vi "MC_7_26_12b_JW.vi"() -> ()   [LabVIEW 2011]
uses:
  <vilib>/Utility/file.llb/Read From Spreadsheet File (string).vi
  <vilib>/Utility/inputDevices.llb/keyboardAcquire.vi
  <vilib>/Utility/file.llb/Write To Spreadsheet File (DBL).vi
  <vilib>/Utility/file.llb/Write To Spreadsheet File (string).vi
  <vilib>/regexp/Match Regular Expression.xnode
panel:
  in  "Room Temp":dbl=294.0
  out "No Image 2":path=path "\\\\acad1\\physics/Jurchescu-group/JW-PD/Image Not Found.png"
  out "Save1 Array":string[][](array[string])
  out "XY Graph-Lin":cluster{dbl[], dbl[]}[](graph)
  out "Lin Vd":dbl
  out "Lin-Vg Array-Used":dbl[](array[numeric])
  out "Lin Id-Used":dbl[](array[numeric])
  out "Comments":string
  out "Folder Index":dbl caption="Length"
  out "Current \nRecord":string[](array[string])
  out "Transformer \nHeaders":string[](array[string])
  out "Current Device ID":string
  out "Column":string
  out "Row":string
  out "Rec: Concentration":dbl
  out "Rec: Solvent":string
  out "Rec: Method":string
  in  "?":T1(tab)
  out "Rec: Material":string
  in  "Treatment Concentration (mM):":dbl=30.0
  in  "Surface Treatment:":string
  in  "# Drops*:":dbl=inf
  in  "Solution Temp (C):":dbl=55.0
  in  "Relative Humidity (%):":dbl=nan
  in  "Room Temp (F):":dbl=nan
  in  "Time (s):":dbl=80.0
  out "Accel (RPM/s):":dbl
  in  "RPM:":dbl=1000.0
  in  "Wait Time (s):":dbl=10.0
  in  "Sample #:":dbl=1.0
  in  "Fabricator:":string="Jeremy"
  in  "Data File":path
  out "Data Folder":path
  in  "Image Folder":path
  out "Image File":path=path "D:/UserData/Desktop/Jeremy/WFU/Research/Programs/VI mods/Image Not Found.png"
  in  "Ramp (s):":dbl=3.0
  out "Calc: On/Off":dbl caption="On/Off-Sat" format="%#_4e"
  out "Calc: Off I-Sat":dbl caption="Off I-Sat" format="%#_4e"
  in  "Manuel-Dielectric":bool
  in  "Manuel-Length":bool
  out "Calc: VT-Lin":dbl
  out "New: VT-Lin":dbl
  out "Rec: VT-Lin":dbl caption="VT-Lin" format="%#_3g"
  out "Calc: Trap Density-STS":dbl format="%#_3e"
  out "New: Trap Density-STS":dbl format="%#_3e"
  out "Rec: Trap Density-STS":dbl caption="N-Sat (STS)" format="%#_3e"
  out "Calc: Trap Density-VT":dbl format="%#_3e"
  out "New: Trap Density-VT":dbl format="%#_3e"
  out "Rec: Trap Density-VT":dbl caption="N-Sat (VT)" format="%#_3e"
  out "Calc: Mobility-Lin":dbl format="%#_4e"
  out "New: Mobility-Lin":dbl format="%#_4e"
  out "Rec: Mobility-Lin":dbl caption="Mobility-Lin" format="%#_4e"
  out "Calc: Mobility-Sat":dbl format="%#_4e"
  out "Rec: Length":dbl caption="Length" format="%#_3g"
  out "Rec: Width":dbl caption="Width" format="%#_4g"
  out "Rec: Dielectric (d)":dbl caption="Dielectric (d)" format="%#_3g"
  out "XY Graph":cluster{dbl[], dbl[]}[](graph)
  in  "NumPts":dbl=5.0
  in  "Cancel Button":bool
  in  "Next Button":bool
  in  "Previous Button":bool
  in  "Up Button":bool
  in  "Down Button":bool
  out "Data Name:":string
  in  "Save Changes?":bool
  in  "New: Dielectric":dbl
  in  "New: Length":dbl
  in  "New: Width":dbl
  out "New: Mobility-Sat":dbl format="%#_4e"
  in  "Slide":dbl(slide) step=1.0 scale=-14.3..89.0 scale format="%#_1p"
  in  "Blank Button":bool
  in  "Zoom":i16(slide)=-3 scale=-5.0..5.0
  out "Image Out 2":T2(plugin-control)
  out "Image Out":T2(plugin-control)
  in  "Magnification":u16(ring) items=["5x", "10x", "20x", "50x", "80x"]
  out "Total Width":dbl
  out "Distances":dbl[](array[numeric])
  in  "Undo Button":bool
  in  "Remove Button":bool
  out "Rec: Mobility-Sat":dbl caption="Mobility-Sat" format="%#_4e"
  out "Index":string
  out "Image Name":string
  in  "Export":bool
  out "Calc: VT-Sat":dbl format="%#_3g"
  out "New: VT-Sat":dbl format="%#_3g"
  in  "Manual-Width":bool caption="Manual"
  out "XY Graph 2":cluster{dbl[], dbl[]}[](graph)
  in  "Next Button 2":bool
  in  "Previous Button 2":bool
  in  "Slide 2":dbl(slide) step=1.0 scale=-1.0..82.0 scale format="%#_1p"
  out "Calc: STS":dbl format="%#_3g"
  out "New: STS":dbl format="%#_3g"
  in  "NumPts 2":dbl=5.0 caption="NumPts"
  out "Rec: VT-Sat":dbl caption="VT-Sat" format="%#_3g"
  out "Rec: STS":dbl caption="STS-Sat" format="%#_3g"
  out "Rec: On/Off":dbl caption="On/Off-Sat" format="%#_4e"
  in  "Save Changes? 2":bool
  in  "Save Changes? 3":bool
  out "Date Recorded":string="Date Recorded" caption="Measured"
  out "Date Created":string caption="Fabricated"
  out "Rec: Temp":dbl caption="Sample Temp"
  out "New: Temp":dbl
  out "Rec: Off I-Sat":dbl caption="Off I-Sat" format="%#_4e"
  out "String":string
  in  "No Image":path=path "\\\\acad1\\physics/Jurchescu-group/JW-PD/Image Not Found.png"
  in  "Project":path=path "\\\\acad1\\physics/Jurchescu-group/JW-PD/Group Library/Origin Project Files/DeviceData_7_25a_JWW.opj"
  out "Index 2":dbl
  out "Sat Id-Log-Used":dbl[](array[numeric])
  out "Vg Array-Log-Used":dbl[](array[numeric])
  out "ROI Descriptor out":T3 {"Contours"."Type" items=["No Selection", "Point", "Line", "Rectangle", "Oval", "Polygon", "Freehand Region", "Annulus", "Unused2", "Unused3", "Broken Line", "Freehand Line", "Rotated Rectangle"]}
  out "ROI Descriptor":T3 {"Contours"."Type" items=["No Selection", "Point", "Line", "Rectangle", "Oval", "Polygon", "Freehand Region", "Annulus", "Unused2", "Unused3", "Broken Line", "Freehand Line", "Rotated Rectangle"]}
  out "Numeric 3":dbl
  out "Array 6":dbl[][](array[numeric])
  out "Cluster":T4
  out "Array 5":dbl[](array[numeric])
  out "Array 4":dbl[](array[numeric])
  out "Array 3":dbl[](array[numeric])
  out "Numeric 2":dbl
  out "Numeric":dbl
  out "Sat Id-Used":dbl[](array[numeric])
  out "Sat Vg Array-Used":dbl[](array[numeric])
  out "MobVi Index":dbl
  in  "Row Start":dbl=20.0
  # "Data Locations"
  # "Data Location"
  # "Image Location"
  # "Sample Properties"
  # "*     Inf = Full coverage\n   NaN = Unknown or Not Applicable"
  # "Recorded"
  # "Calculated"
  # "Re-Calculated"
  # "Manual"
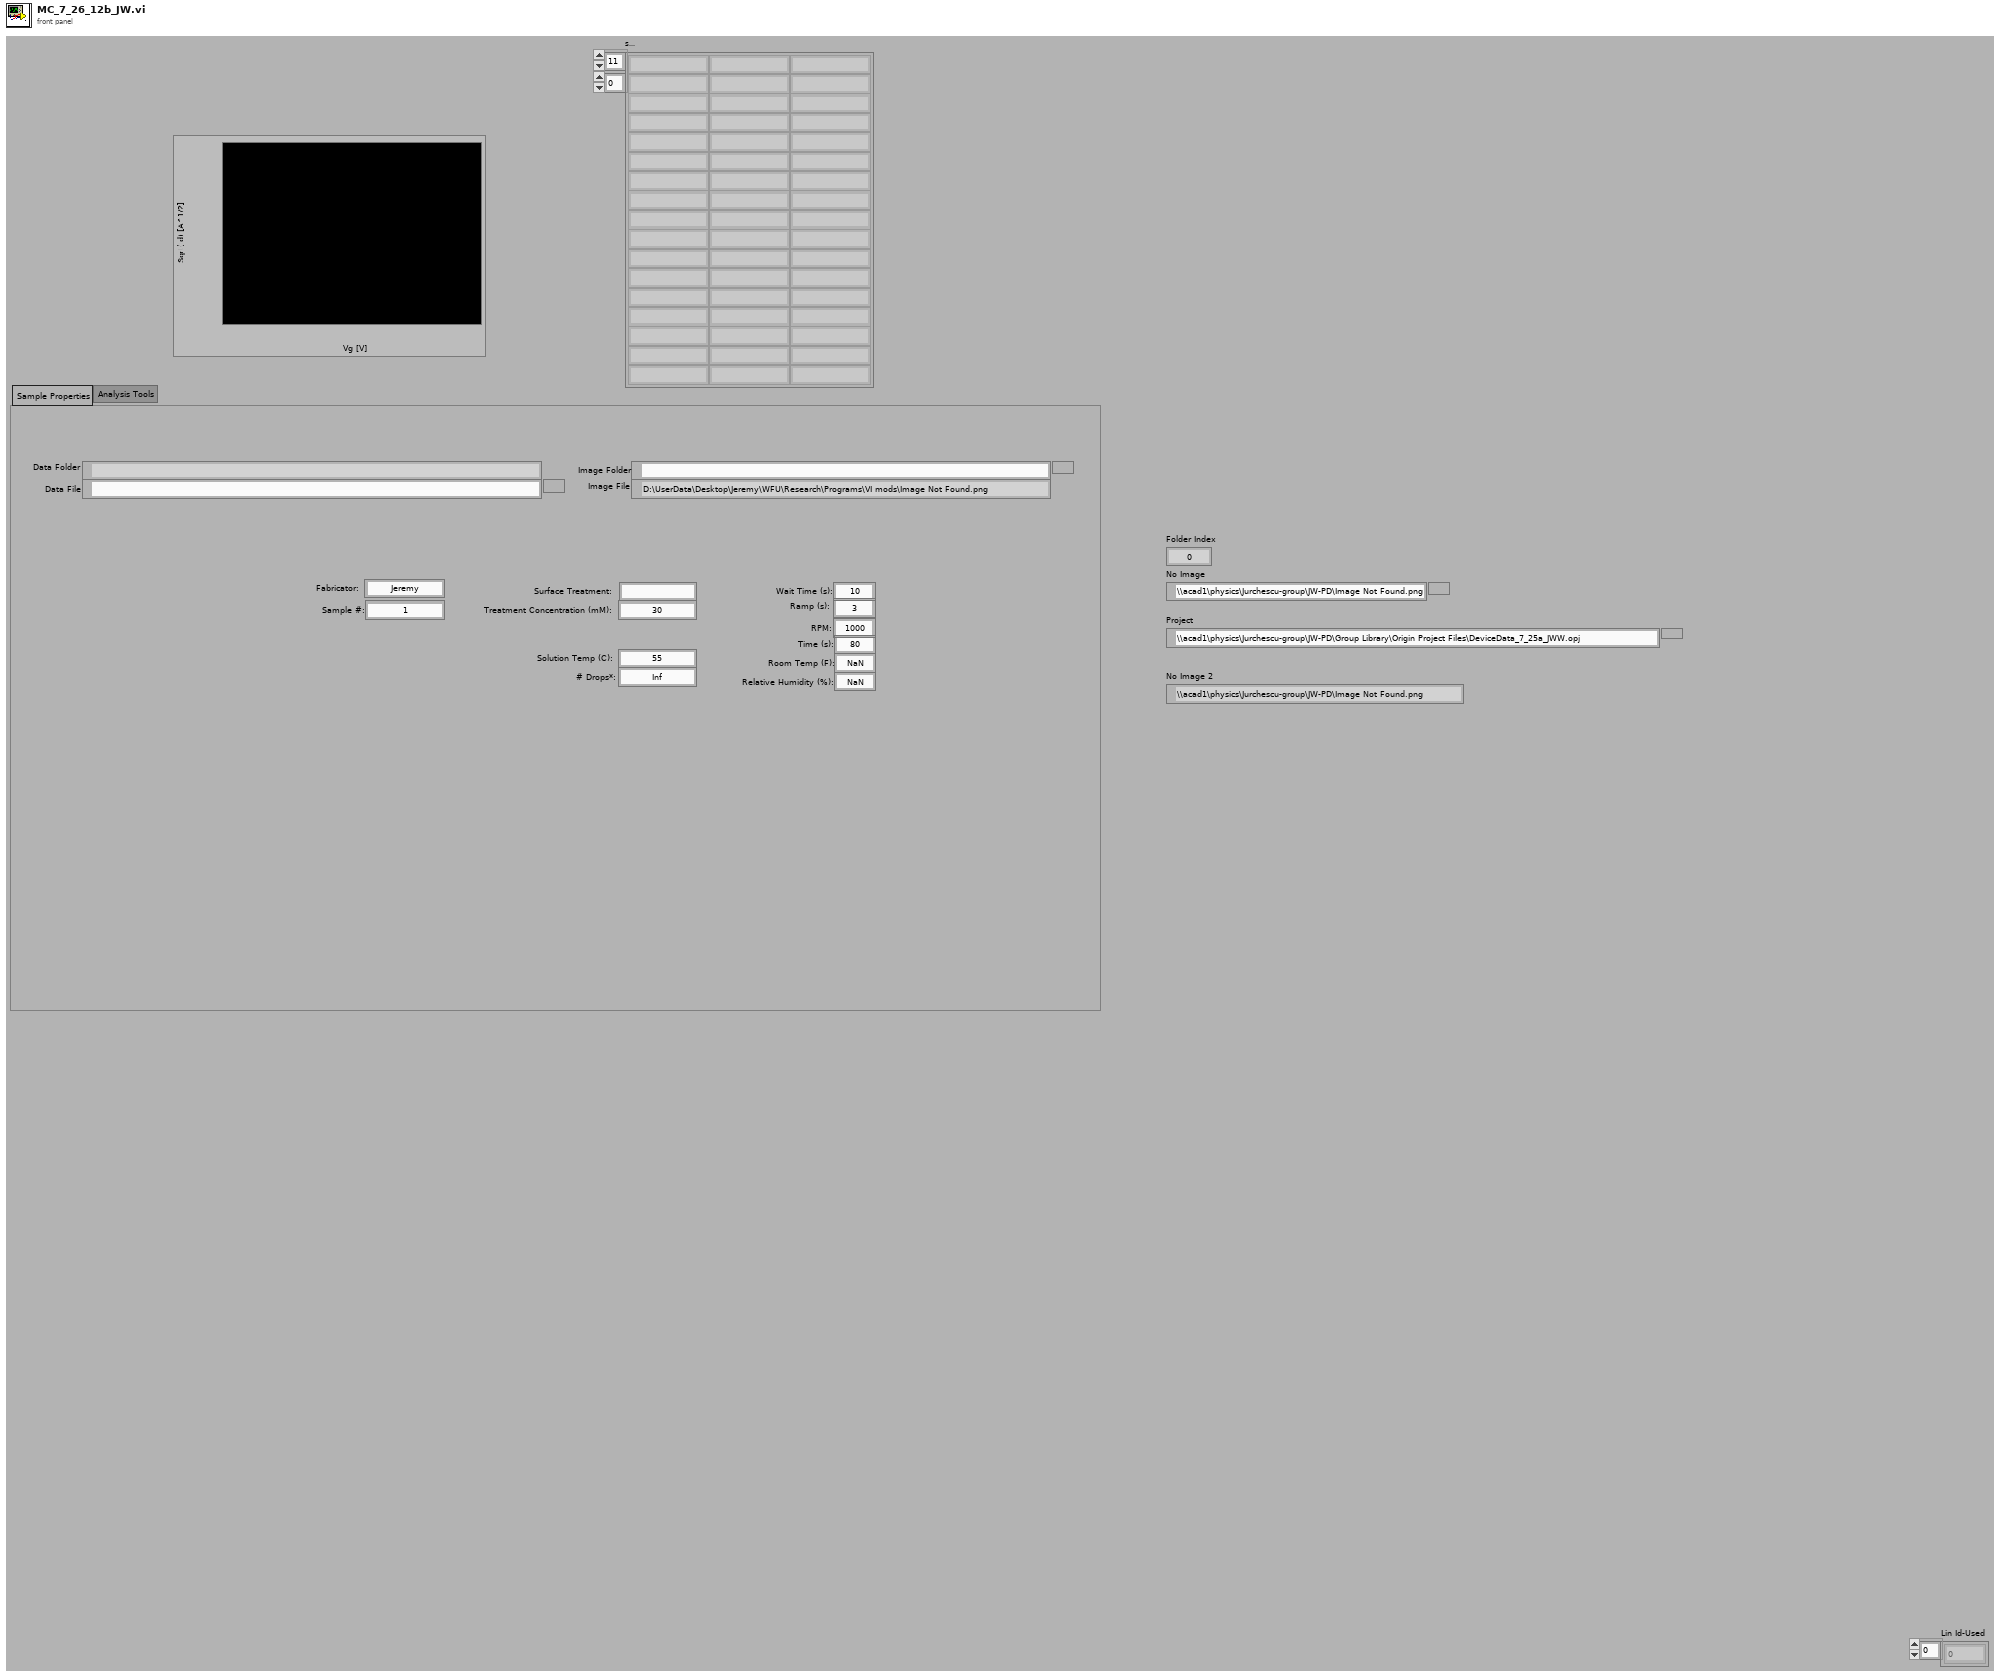
[diagram p1: front panel]
types:
  T1 = enum32{"Sample Properties", "Analysis Tools", "Current Database"}
  T2 = typedef "IMAQ Image.ctl" = refnum<image>
  T3 = typedef "ROI Descriptor" = cluster{"Global Rectangle":i32[], "Contours":cluster{"ID":enum32{"External", "Internal"}, "Type":u32, "Coordinates":i32[]}[]}
  T4 = cluster{"Numeric":dbl, "Numeric 2":dbl, "Numeric 3":dbl, "Numeric 4":dbl}
  T5 = cluster{"Mobility-Sat":dbl, "Moblitity-Lin":dbl, "On/Off":dbl, "Off Current":dbl, "Vt-Sat":dbl, "STS":dbl, "Trap Density-VT":dbl, "Trap Density-STS":dbl}
  T6 = cluster{"Date Recorded":string, "Index":string, "Length":dbl, "Width":dbl, "Sample Temp":dbl}
  T7 = cluster{"Date Created":string, "Material":string, "Solvent":string, "Concentration":dbl, "Method":string, "Dielectric (nm)":dbl, "Treatment":string, "Comments":string}
  T8 = cluster{"Mobility-Sat":dbl, "Vt-Sat":dbl, "Mobility-Lin":dbl, "Vt-Lin":dbl, "Off I-Sat":dbl, "On/Off I-Sat":dbl}
  T9 = cluster{"[0]":cluster{dbl[], dbl[]}, "[1]":cluster{dbl[], dbl[]}, "[2]":cluster{dbl[], dbl[]}, "[3]":cluster{dbl[], dbl[]}, "[4]":cluster{dbl[], dbl[]}, "[5]":cluster{dbl[], dbl[]}, "[6]":cluster{dbl[], dbl[]}, "[7]":cluster{dbl[], dbl[]}, "[8]":cluster{dbl[], dbl[]}}
  T10 = cluster{"Global Rectangle":i32[], "Contours":cluster{"Contour Type":u32, "ROI Type":u32, "Points":i32[]}[]}
  T11 = typedef "LVBoundsTypeDef.ctl" = cluster{"Width":u32, "Height":u32}
  T12 = enum16{"0", "1", "2", "3", "4", "5", "6", "7", "8", "9", "A", "B", "C", "D", "E", "F", "G", "H", "I", "J", "K", "L", "M", "N", "O", "P", "Q", "R", "S", "T", "U", "V", "W", "X", "Y", "Z", "F1", "F2", "F3", "F4", "F5", "F6", "F7", "F8", "F9", "F10", "F11", "F12", "F13", "F14", "F15", "ADD", "BACK", "BACKSLASH", "CAPITAL", "COMMA", "DECIMAL", "DELETE", "DIVIDE", "DOWN", "END", "EQUALS", "ESCAPE", "GRAVE (`)", "HOME", "INSERT", "LBRACKET", "LCONTROL", "LEFT", "L ALT", "LSHIFT", "LWIN", "MINUS", "MULTIPLY", "NEXT", "NUMLOCK", "NUMPAD_0", "NUMPAD_1", "NUMPAD_2", "NUMPAD_3", "NUMPAD_4", "NUMPAD_5", "NUMPAD_6", "NUMPAD_7", "NUMPAD_8", "NUMPAD_9", "PAUSE", "PERIOD", "PRIOR (PG UP)", "RBRACKET", "RCONTROL", "RETURN", "RIGHT", "R ALT", "RSHIFT", "RWIN", "SCROLL", "SEMICOLON", "SLASH", "SPACE", "SUBTRACT", "TAB", "UP", "ENTER (num pad)", "' (quote)"}[]
  T13 = enum16{"0", "1", "2", "3", "4", "5", "6", "7", "8", "9", "A", "B", "C", "D", "E", "F", "G", "H", "I", "J", "K", "L", "M", "N", "O", "P", "Q", "R", "S", "T", "U", "V", "W", "X", "Y", "Z", "F1", "F2", "F3", "F4", "F5", "F6", "F7", "F8", "F9", "F10", "F11", "F12", "F13", "F14", "F15", "ADD", "BACK", "BACKSLASH", "CAPITAL", "COMMA", "DECIMAL", "DELETE", "DIVIDE", "DOWN", "END", "EQUALS", "ESCAPE", "GRAVE (`)", "HOME", "INSERT", "LBRACKET", "LCONTROL", "LEFT", "L ALT", "LSHIFT", "LWIN", "MINUS", "MULTIPLY", "NEXT", "NUMLOCK", "NUMPAD_0", "NUMPAD_1", "NUMPAD_2", "NUMPAD_3", "NUMPAD_4", "NUMPAD_5", "NUMPAD_6", "NUMPAD_7", "NUMPAD_8", "NUMPAD_9", "PAUSE", "PERIOD", "PRIOR (PG UP)", "RBRACKET", "RCONTROL", "RETURN", "RIGHT", "R ALT", "RSHIFT", "RWIN", "SCROLL", "SEMICOLON", "SLASH", "SPACE", "SUBTRACT", "TAB", "UP", "ENTER (num pad)", "' (quote)"}
  T14 = cluster{"Contour Type":u32, "ROI Type":u32, "Points":i32[]}[]
  T15 = cluster{i32[], cluster{"Contour Type":u32, "ROI Type":u32, "Points":i32[]}[]}
  T16 = cluster{string, sgl, bool, bool, bool, bool, bool, bool, i32}
  T17 = cluster{i32, cluster{string, sgl, bool, bool, bool, bool, bool, bool, i32}, i32, i32}
  T18 = cluster{"Contour Type":u32, "ROI Type":u32, "Points":i32[]}
  T19 = cluster{"Points[0]":i32, "Points[1]":i32, "Points[2]":i32, "Points[3]":i32, "Points[4]":i32, "Points[5]":i32, "Points[6]":i32, "Points[7]":i32, "Points[8]":i32}
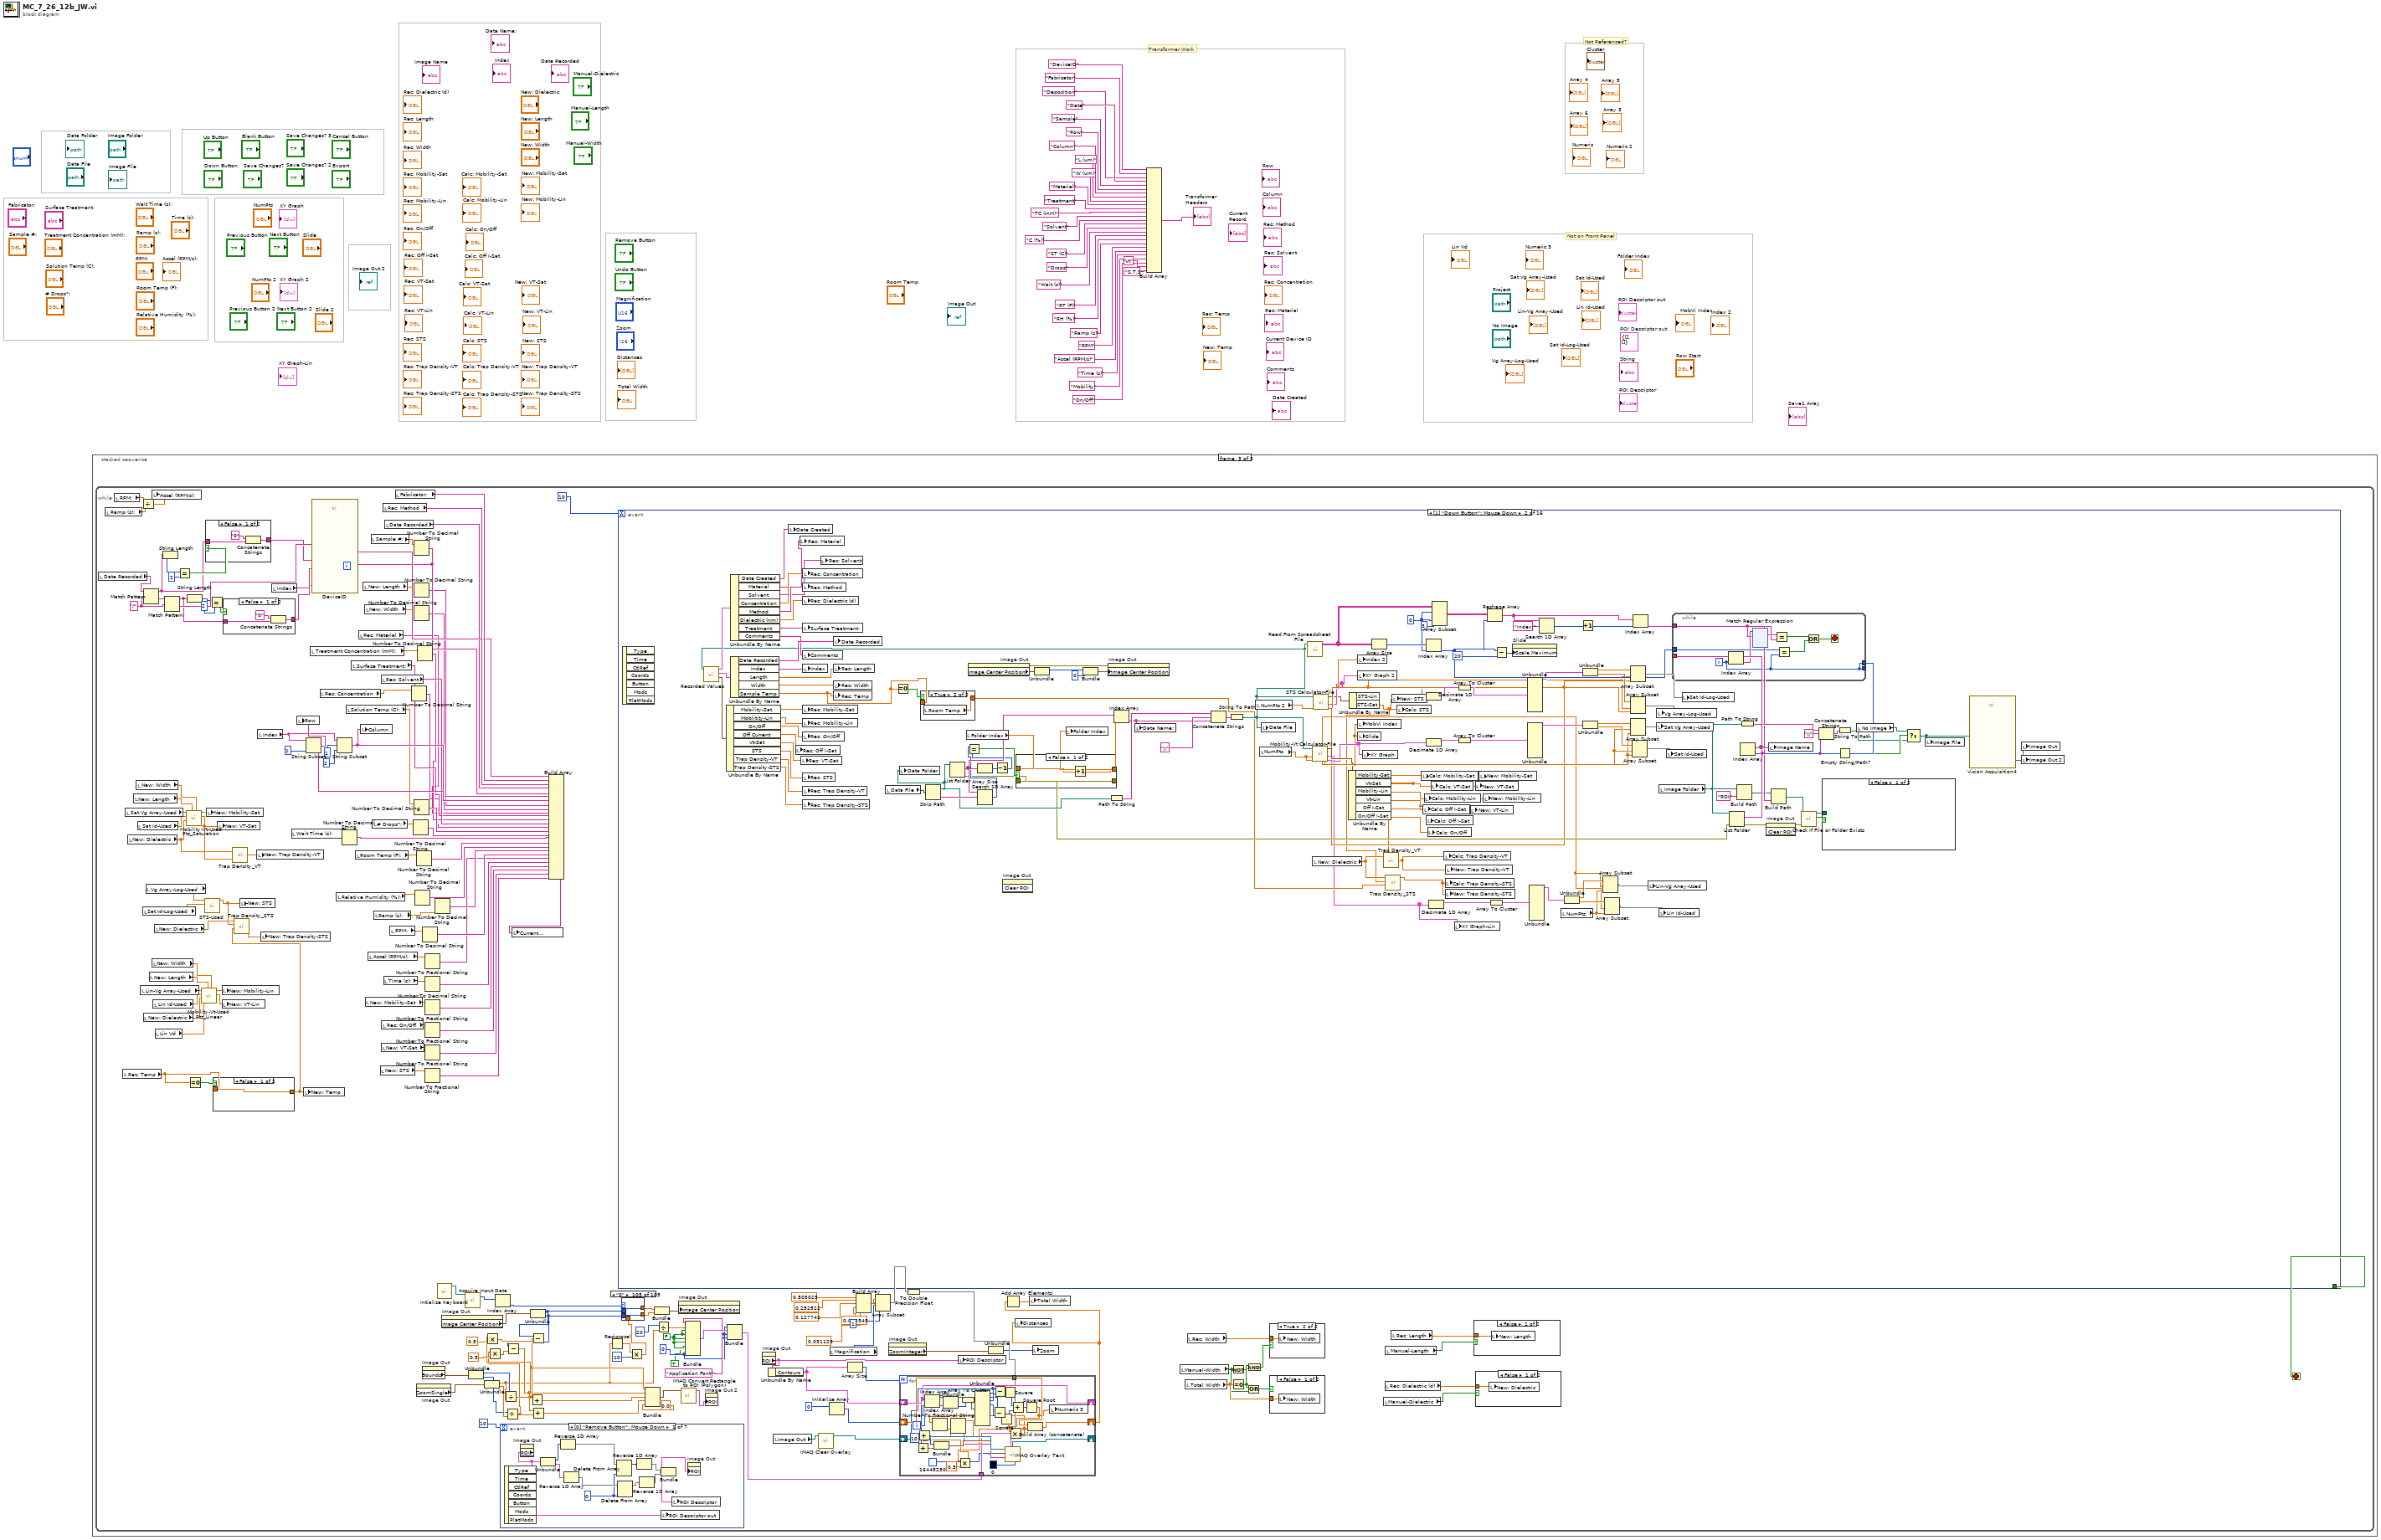
[diagram p0: block diagram]
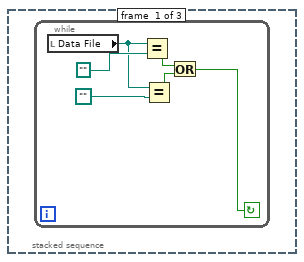
[diagram p2: hidden frame]
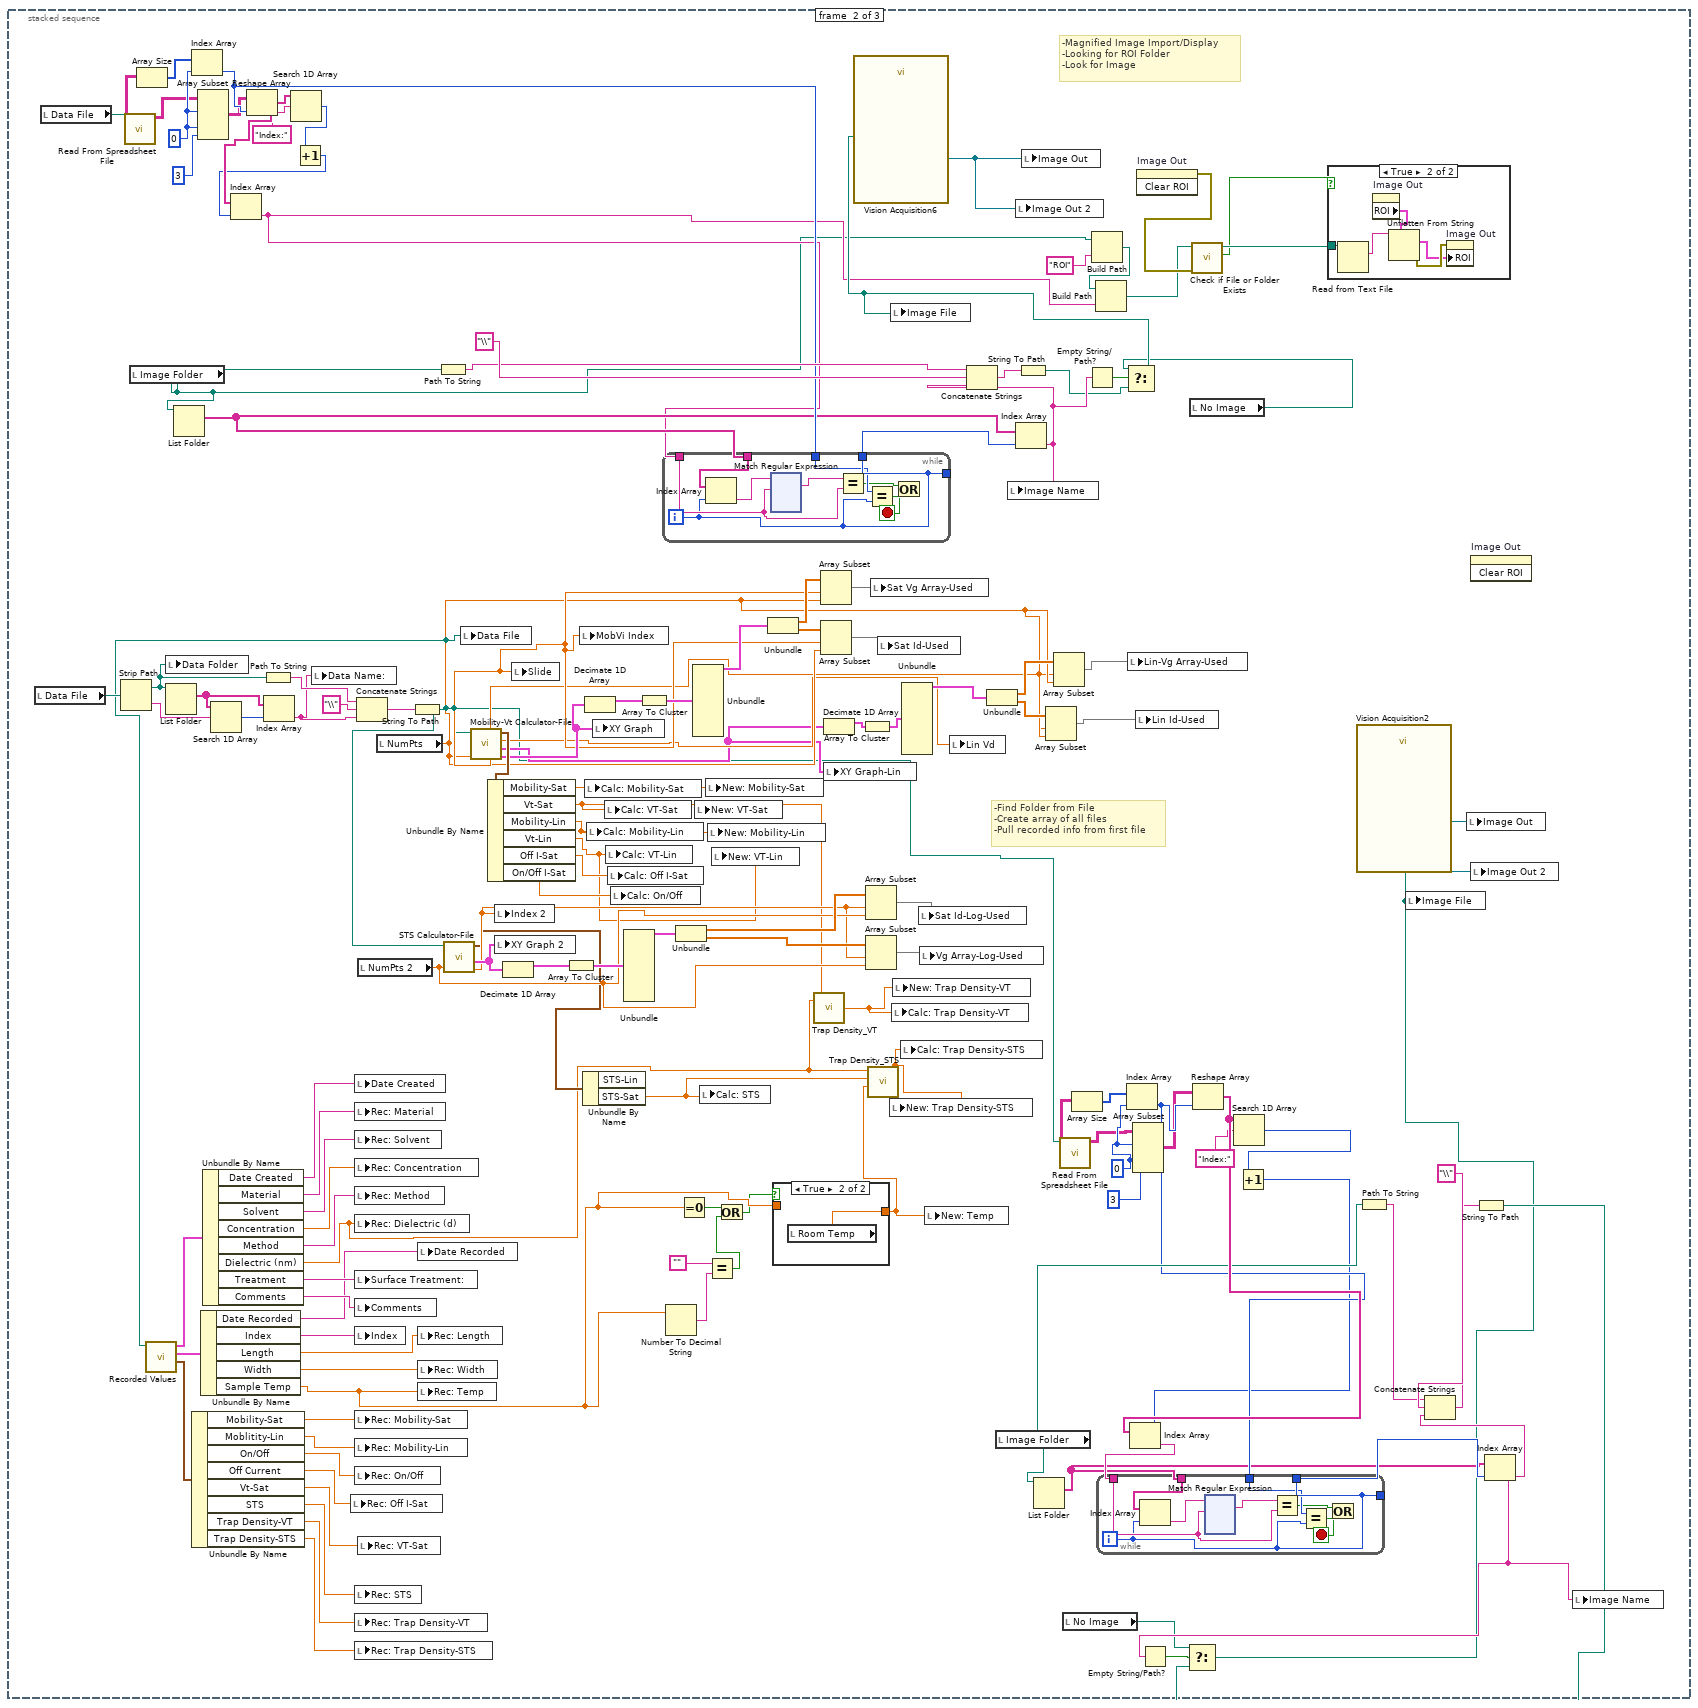
[diagram p3: hidden frame]
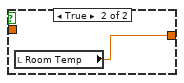
[diagram p6: hidden frame]
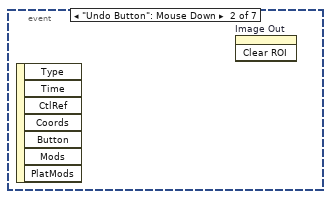
[diagram p13: hidden frame]
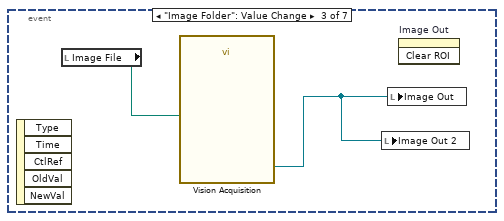
[diagram p14: hidden frame]
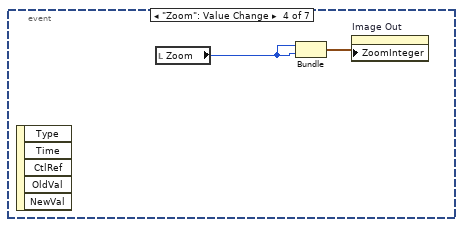
[diagram p15: hidden frame]
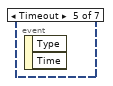
[diagram p16: hidden frame]
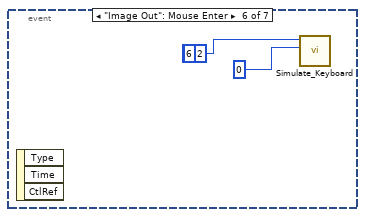
[diagram p17: hidden frame]
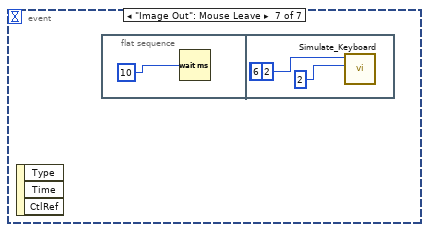
[diagram p18: hidden frame]
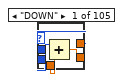
[diagram p19: hidden frame]
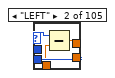
[diagram p20: hidden frame]
diagram:
  (unwired) T3 {"Global Rectangle"=[], "Contours"=[]}  # ROI Descriptor out
  # "Not Referenced?"
  # "Transformer Work"
  # "Not on Front Panel"
  n1 = stacked-sequence {
    frame #0 {
      n2 = while {
        stop <- w29 continue-if-true
        n3 = local read "Data File"() -> (w31:path)
        n4 = Equal?(x=w31, y=path "") -> (x = y?=w33:bool)
        n5 = Equal?(x=w31, y=path "") -> (x = y?=w32:bool)
        n6 = Or(x=w33, y=w32) -> (x .or. y?=w29:bool)
      }
    }
    frame #1 {
      w133 = 0
      w157 = 0
      # "-Find Folder from File\n-Create array of all files\n-Pull recorded info from first file"
      # "-Magnified Image Import/Display\n-Looking for ROI Folder\n-Look for Image"
      n7 = local read "Data File"() -> (w137:path)
      n8 = local read "Data File"() -> (w152:path)
      n9 = Strip Path(path=w137) -> (stripped path=w138:path, name=w124:string)
      n10 = call-poly <vilib>:"Read From Spreadsheet File.vi"("file path (dialog if empty)"=w152) -> ("all rows"=w155:string[][])  [unwired: 6 in, 4 out]
      n11 = local read "Image Folder"() -> (w94:path)
      n12 = Array Size(array=w155) -> (size(s)=w156:i32[])
      n13 = local write "Data Folder"(w138) -> ()
      n14 = List Folder(path=w138) -> (filenames=w128:string[])  [unwired: 3 in, 3 out]
      n15 = List Folder(path=w94) -> (filenames=w161:string[])  [unwired: 3 in, 3 out]
      n16 = Index Array(array=w156, index=w157) -> (element=w163:i32)
      n17 = Array Subset(array=w155, index (row)=w157, index (col)=w157, length (col)=3) -> (w154:string[][])  [unwired: 1 in]
      n18 = Search 1D Array(1D array=w128, element=w124) -> (index of element=w127:i32)  [unwired: 1 in]
      n19 = Reshape Array(w154, w163) -> (w168:string[])
      n20 = Path To String(path=w138) -> (string=w123:string)
      n21 = Index Array(array=w128, index=w127) -> (element=w93:string)
      n22 = Search 1D Array(1D array=w168, element="Index:") -> (index of element=w160:i32)  [unwired: 1 in]
      n23 = Increment(x=w160) -> (x+1=w159:i32)
      n24 = Index Array(array=w168, index=w159) -> (element=w95:string)
      n25 = local write "Data Name:"(w93) -> ()
      n26 = Concatenate Strings(w123, "\\", w93) -> (w125:string)
      n27 = local read "NumPts 2"() -> (w68:dbl)
      n28 = local read "NumPts"() -> (w59:dbl)
      n29 = String To Path(string=w125) -> (path=w52:path)
      n30 = call "Recorded Values.vi"("Path"=w52) -> ("Recorded Char"=w91:T5, "Recorded Prop"=w90:T6, "Fabrication Prop"=w92:T7)  [unwired: 8 in]
      n31 = Unbundle By Name(w91) -> ("Mobility-Sat"=w79:dbl, "Moblitity-Lin"=w78:dbl, "On/Off"=w77:dbl, "Off Current"=w76:dbl, "Vt-Sat"=w38:dbl, "STS"=w75:dbl, "Trap Density-VT"=w74:dbl, "Trap Density-STS"=w73:dbl)
      n32 = Unbundle By Name(w90) -> ("Date Recorded"=w83:string, "Index"=w82:string, "Length"=w81:dbl, "Width"=w80:dbl, "Sample Temp"=w44:dbl)
      n33 = Unbundle By Name(w92) -> ("Date Created"=w72:string, "Material"=w89:string, "Solvent"=w88:string, "Concentration"=w87:dbl, "Method"=w86:string, "Dielectric (nm)"=w48:dbl, "Treatment"=w85:string, "Comments"=w84:string)
      n34 = local write "Rec: Off I-Sat"(w76) -> ()
      n35 = local write "Date Created"(w72) -> ()
      n36 = local write "Rec: Material"(w89) -> ()
      n37 = local write "Rec: Solvent"(w88) -> ()
      n38 = local write "Rec: Concentration"(w87) -> ()
      n39 = local write "Rec: Method"(w86) -> ()
      n40 = local write "Rec: Dielectric (d)"(w48) -> ()
      n41 = local write "Surface Treatment:"(w85) -> ()
      n42 = local write "Comments"(w84) -> ()
      n43 = local write "Index"(w82) -> ()
      n44 = local write "Rec: Mobility-Sat"(w79) -> ()
      n45 = local write "Rec: Mobility-Lin"(w78) -> ()
      n46 = local write "Rec: On/Off"(w77) -> ()
      n47 = local write "Rec: STS"(w75) -> ()
      n48 = local write "Rec: Trap Density-VT"(w74) -> ()
      n49 = local write "Rec: Trap Density-STS"(w73) -> ()
      n50 = local write "Rec: VT-Sat"(w38) -> ()
      n51 = local write "Date Recorded"(w83) -> ()
      n52 = local write "Rec: Length"(w81) -> ()
      n53 = local write "Rec: Width"(w80) -> ()
      n54 = local write "Rec: Temp"(w44) -> ()
      n55 = Path To String(path=w94) -> (string=w165:string)
      n56 = call "STS Calculator-File.vi"("NumPts"=w68, "Path"=w52) -> ("STS Index-Sat"=w66:dbl, "XY Graph-Sat"=w67:cluster{dbl[], dbl[]}[], "Ouput"=w65:cluster{"STS-Sat":dbl, "STS-Lin":dbl})  [unwired: 5 in, 2 out]
      n57 = local write "Data File"(w52) -> ()
      n58 = call "Mobility-Vt Calculator-File.vi"("NumPts"=w59, "Path"=w52) -> ("XY Graph-Sat"=w70:cluster{dbl[], dbl[]}[], "XY Graph-Lin"=w54:cluster{dbl[], dbl[]}[], "Lin Vd"=w55:dbl, "Output"=w71:T8, "Index-Sat"=w69:dbl, "Index-Lin"=w58:dbl)  [unwired: 4 in]
      n59 = Unbundle By Name(w71) -> ("Mobility-Sat"=w47:dbl, "Vt-Sat"=w46:dbl, "Mobility-Lin"=w37:dbl, "Vt-Lin"=w35:dbl, "Off I-Sat"=w53:dbl, "On/Off I-Sat"=w36:dbl)
      n60 = local write "Index 2"(w66) -> ()
      n61 = local write "XY Graph 2"(w67) -> ()
      n62 = Decimate 1D Array(w67) -> (w115:cluster{dbl[], dbl[]}[])  [unwired: 1 out]
      n63 = local write "Slide"(w69) -> ()
      n64 = Array To Cluster(array=w115) -> (cluster=w117:T9)
      n65 = local write "MobVi Index"(w69) -> ()
      n66 = Unbundle By Name(w65) -> ("STS-Sat"=w51:dbl)  [unwired: 1 out]
      n67 = Decimate 1D Array(w70) -> (w151:cluster{dbl[], dbl[]}[])  [unwired: 1 out]
      n68 = local write "Calc: Mobility-Sat"(w47) -> ()
      n69 = local write "Calc: Mobility-Lin"(w37) -> ()
      n70 = local write "XY Graph"(w70) -> ()
      n71 = local write "Calc: VT-Sat"(w46) -> ()
      n72 = local write "Calc: VT-Lin"(w35) -> ()
      n73 = local write "Calc: Off I-Sat"(w53) -> ()
      n74 = local write "Calc: On/Off"(w36) -> ()
      n75 = Unbundle(w117) -> ("[0]"=w116:cluster{dbl[], dbl[]})  [unwired: 8 out]
      n76 = Array To Cluster(array=w151) -> (cluster=w149:T9)
      n77 = while {
        tunnel: w161 -> [w303]
        tunnel: w95 -> [w301]
        tunnel: [w300] -> _
        tunnel: [w300] -> w162
        tunnel: w163 -> [w299]
        i -> [w300]
        stop <- w296 stop-if-true
        n78 = Index Array(array=w303, index=w300) -> (element=w304:string)
        n79 = xnode "Match Regular Expression"("input string"=w304, "regular expression"=w301) -> ("whole match"=w302:string)  [unwired: 4 in, 4 out]
        n80 = Equal?(x=w302, y=w301) -> (x = y?=w298:bool)
        n81 = Equal?(x=w299, y=w300) -> (x = y?=w297:bool)
        n82 = Or(x=w298, y=w297) -> (x .or. y?=w296:bool)
      }
      n83 = Number To Decimal String(number=w44) -> (decimal integer string=w42:string)  [unwired: 1 in]
      n84 = Unbundle(w116) -> (w113:dbl[], w112:dbl[])
      n85 = Equal To 0?(x=w44) -> (x = 0?=w43:bool)
      n86 = Unbundle(w149) -> ("[0]"=w150:cluster{dbl[], dbl[]})  [unwired: 8 out]
      n87 = local write "New: VT-Sat"(w46) -> ()
      n88 = local write "Calc: STS"(w51) -> ()
      n89 = local write "New: Mobility-Sat"(w47) -> ()
      n90 = Equal?(x="", y=w42) -> (x = y?=w40:bool)
      n91 = local write "New: Mobility-Lin"(w37) -> ()
      n92 = local write "New: VT-Lin"(w35) -> ()
      n93 = Or(x=w43, y=w40) -> (x .or. y?=w39:bool)
      n94 = Unbundle(w150) -> (w114:dbl[], w118:dbl[])
      n95 = case shown="True" w39 {
        tunnel: [w169 w170] -> w50
        tunnel: w44 -> [w169 _]
        frame False {
        }
        frame True {
          n96 = local read "Room Temp"() -> (w170:dbl)
        }
      }
      n97 = call "Trap Density_VT.vi"("VT"=w46, "Dielectric"=w48) -> ("Trap Density-VT"=w45:dbl)
      n98 = Array Subset(array=w114, index=w69, length=w59) -> (w121:dbl[])
      n99 = Array Subset(array=w118, index=w69, length=w59) -> (w122:dbl[])
      n100 = Decimate 1D Array(w54) -> (w64:cluster{dbl[], dbl[]}[])  [unwired: 1 out]
      n101 = local write "XY Graph-Lin"(w54) -> ()
      n102 = Array To Cluster(array=w64) -> (cluster=w63:T9)
      n103 = Array Subset(array=w113, index=w66, length=w68) -> (w120:dbl[])
      n104 = Array Subset(array=w112, index=w66, length=w68) -> (w119:dbl[])
      n105 = call "Trap Density_STS.vi"("Temp (T) [K]"=w50, "S.T.S. (S)"=w51, "Dielectric"=w48) -> ("Trap Density (N)"=w49:dbl)  [unwired: 8 in]
      n106 = local write "Sat Vg Array-Used"(w121) -> ()
      n107 = local write "Sat Id-Used"(w122) -> ()
      n108 = local write "New: Trap Density-STS"(w49) -> ()
      n109 = local write "Calc: Trap Density-VT"(w45) -> ()
      n110 = local write "New: Trap Density-VT"(w45) -> ()
      n111 = local write "Calc: Trap Density-STS"(w49) -> ()
      n112 = Unbundle(w63) -> ("[0]"=w62:cluster{dbl[], dbl[]})  [unwired: 8 out]
      n113 = local write "Sat Id-Log-Used"(w120) -> ()
      n114 = local write "Vg Array-Log-Used"(w119) -> ()
      n115 = local write "New: Temp"(w50) -> ()
      n116 = local write "Lin Vd"(w55) -> ()
      n117 = Unbundle(w62) -> (w61:dbl[], w60:dbl[])
      n118 = local read "Image Folder"() -> (w144:path)
      n119 = Index Array(array=w161, index=w162) -> (element=w111:string)
      n120 = Concatenate Strings(w165, "\\", w111) -> (w166:string)
      n121 = local write "Image Name"(w111) -> ()
      n122 = String To Path(string=w166) -> (path=w109:path)
      n123 = List Folder(path=w144) -> (filenames=w140:string[])  [unwired: 3 in, 3 out]
      n124 = Array Subset(array=w60, index=w58, length=w59) -> (w56:dbl[])
      n125 = Array Subset(array=w61, index=w58, length=w59) -> (w57:dbl[])
      n126 = call-poly <vilib>:"Read From Spreadsheet File.vi"("file path (dialog if empty)"=w52) -> ("all rows"=w131:string[][])  [unwired: 6 in, 4 out]
      n127 = local read "No Image"() -> (w103:path)
      n128 = Array Size(array=w131) -> (size(s)=w132:i32[])
      n129 = Empty String/Path?(string/path=w111) -> (empty?=w110:bool)
      n130 = Build Path(base path=w94, name or relative path="ROI") -> (appended path=w97:path)
      n131 = Build Path(base path=w97, name or relative path=w95) -> (appended path=w96:path)
      n132 = Index Array(array=w132, index=w133) -> (element=w143:i32)
      n133 = local write "Lin-Vg Array-Used"(w57) -> ()
      n134 = Array Subset(array=w131, index (row)=w133, index (col)=w133, length (col)=3) -> (w130:string[][])  [unwired: 1 in]
      n135 = local write "Lin Id-Used"(w56) -> ()
      n136 = invoke on="Image Out" class="ImageControl" method="Clear ROI"() -> (error out=w101:errorcluster)  [unwired: 3 in, 2 out]
      n137 = local read "No Image"() -> (w102:path)
      n138 = Select(t=w102, s=w110, f=w109) -> (s? t:f=w108:path)
      n139 = call "Vision Acquisition6"("Image Path"=w108) -> ("Image Out"=w164:T2)  [unwired: 25 in, 1 out]
      n140 = local write "Image File"(w108) -> ()
      n141 = local write "Image Out 2"(w164) -> ()
      n142 = local write "Image Out"(w164) -> ()
      n143 = call <vilib>:"Check if File or Folder Exists.vi"("error in (no error)"=w101, "path"=w96) -> ("file or folder exists?"=w99:bool, "dup path"=w100:path)  [unwired: 7 in, 1 out]
      n144 = Reshape Array(w130, w143) -> (w148:string[])
      n145 = Search 1D Array(1D array=w148, element="Index:") -> (index of element=w136:i32)  [unwired: 1 in]
      n146 = Increment(x=w136) -> (x+1=w135:i32)
      n147 = Index Array(array=w148, index=w135) -> (element=w141:string)
      n148 = while {
        tunnel: w140 -> [w183]
        tunnel: w141 -> [w181]
        tunnel: [w180] -> _
        tunnel: [w180] -> w142
        tunnel: w143 -> [w179]
        i -> [w180]
        stop <- w176 stop-if-true
        n149 = Index Array(array=w183, index=w180) -> (element=w184:string)
        n150 = xnode "Match Regular Expression"("input string"=w184, "regular expression"=w181) -> ("whole match"=w182:string)  [unwired: 4 in, 4 out]
        n151 = Equal?(x=w182, y=w181) -> (x = y?=w178:bool)
        n152 = Equal?(x=w179, y=w180) -> (x = y?=w177:bool)
        n153 = Or(x=w178, y=w177) -> (x .or. y?=w176:bool)
      }
      n154 = case shown="True" w99 {
        tunnel: w100 -> [_ w171]
        frame False {
        }
        frame True {
          n155 = Read from Text File(file (use dialog)=w171) -> (text=w175:string)  [unwired: 3 in, 3 out]
          n156 = property on="Image Out" class="ImageControl"() -> ("ROI"=w172:T10)  [unwired: 2 in, 2 out]
          n157 = Unflatten From String(type=w172, binary string=w175) -> (value=w173:T10, error out=w174:errorcluster)  [unwired: 3 in, 1 out]
          n158 = property on="Image Out" class="ImageControl"(error in=w174, "ROI"=w173) -> ()  [unwired: 1 in, 2 out]
        }
      }
      n159 = Path To String(path=w144) -> (string=w145:string)
      n160 = invoke on="Image Out" class="ImageControl" method="Clear ROI"() -> ()  [unwired: 3 in, 3 out]
      n161 = Index Array(array=w140, index=w142) -> (element=w106:string)
      n162 = Empty String/Path?(string/path=w106) -> (empty?=w107:bool)
      n163 = Concatenate Strings(w145, "\\", w106) -> (w146:string)
      n164 = String To Path(string=w146) -> (path=w105:path)
      n165 = Select(t=w103, s=w107, f=w105) -> (s? t:f=w104:path)
      n166 = call "Vision Acquisition2"("Image Path"=w104) -> ("Image Out"=w139:T2)  [unwired: 25 in, 1 out]
      n167 = local write "Image File"(w104) -> ()
      n168 = local write "Image Out"(w139) -> ()
      n169 = local write "Image Out 2"(w139) -> ()
      n170 = local write "Image Name"(w106) -> ()
    }
    frame #2 {
      n171 = while {
        stop <- w581 stop-if-true
        w477 = "/"
        w531 = FALSE
        w529 = 0
        n172 = local read "Date Recorded"() -> (w480:string)
        n173 = local read "Ramp (s):"() -> (w447:dbl)
        n174 = local read "RPM:"() -> (w448:dbl)
        n175 = local read "Rec: Temp"() -> (w419:dbl)
        n176 = local read "Sat Vg Array-Used"() -> (w436:dbl[])
        n177 = local read "New: Dielectric"() -> (w421:dbl)
        n178 = local read "New: Length"() -> (w437:dbl)
        n179 = local read "New: Width"() -> (w439:dbl)
        n180 = local read "Sat Id-Used"() -> (w435:dbl[])
        n181 = local read "Lin-Vg Array-Used"() -> (w430:dbl[])
        n182 = Divide(x=w448, y=w447) -> (x/y=w446:dbl)
        n183 = local read "Sat Id-Log-Used"() -> (w434:dbl[])
        n184 = local read "New: Dielectric"() -> (w427:dbl)
        n185 = Match Pattern(string=w480, regular expression=w477) -> (before substring=w471:string, after substring=w478:string)  [unwired: 1 in, 2 out]
        n186 = local read "Vg Array-Log-Used"() -> (w433:dbl[])
        n187 = local read "New: Length"() -> (w429:dbl)
        n188 = local write "Accel (RPM/s):"(w446) -> ()
        n189 = local read "New: Width"() -> (w426:dbl)
        n190 = local read "Lin Id-Used"() -> (w431:dbl[])
        n191 = local read "New: Dielectric"() -> (w423:dbl)
        n192 = local read "Lin Vd"() -> (w425:dbl)
        n193 = String Length(string=w471) -> (length=w474:i32)
        n194 = Match Pattern(string=w478, regular expression=w477) -> (before substring=w465:string, after substring=w476:string)  [unwired: 1 in, 2 out]
        n195 = Equal?(x=w474, y=2) -> (x = y?=w472:bool)
        n196 = call "Mobility-Vt-Used Pts_Saturation.vi"("Width"=w439, "Length"=w437, "Dielectric (d)"=w421, "Sat Id Used"=w435, "Vg Used"=w436) -> ("Vt"=w422:dbl, "Mobility"=w438:dbl)  [unwired: 4 in, 1 out]
        n197 = String Length(string=w465) -> (length=w467:i32)
        n198 = Equal To 0?(x=w419) -> (x = 0?=w418:bool)
        n199 = call "Mobility-Vt-Used Pts_Linear.vi"("Width"=w426, "Length"=w429, "Vd"=w425, "Dielectric (d)"=w427, "Sat Id Used"=w431, "Vg Used"=w430) -> ("Vt"=w432:dbl, "Mobility"=w428:dbl)  [unwired: 3 in, 1 out]
        n200 = call "STS-Used.vi"("Id Used"=w434, "Vg-Used"=w433) -> ("STS"=w424:dbl)  [unwired: 9 in]
        n201 = case shown="False" w472 {
          tunnel: w471 -> [w591 w593]
          tunnel: [w590 w593] -> w470
          frame False {
            n202 = Concatenate Strings("0", w591) -> (w590:string)
          }
          frame True {
          }
        }
        n203 = local write "New: Mobility-Sat"(w438) -> ()
        n204 = Equal?(x=w467, y=2) -> (x = y?=w469:bool)
        n205 = case shown="False" w418 {
          tunnel: [w582 w583] -> w416
          tunnel: w419 -> [w582 _]
          frame False {
          }
          frame True {
            n206 = local read "Room Temp"() -> (w583:dbl)
          }
        }
        n207 = local write "New: VT-Sat"(w422) -> ()
        n208 = local write "New: Mobility-Lin"(w428) -> ()
        n209 = local write "New: VT-Lin"(w432) -> ()
        n210 = case shown="False" w469 {
          tunnel: w465 -> [w587 w589]
          tunnel: [w586 w589] -> w466
          frame False {
            n211 = Concatenate Strings("0", w587) -> (w586:string)
          }
          frame True {
          }
        }
        n212 = call "Trap Density_VT.vi"("VT"=w422, "Dielectric"=w421) -> ("Trap Density-VT"=w420:dbl)
        n213 = call "Trap Density_STS.vi"("Temp (T) [K]"=w416, "S.T.S. (S)"=w424, "Dielectric"=w423) -> ("Trap Density (N)"=w417:dbl)  [unwired: 8 in]
        n214 = local write "New: STS"(w424) -> ()
        n215 = local write "New: Trap Density-VT"(w420) -> ()
        n216 = local read "Index"() -> (w450:string)
        n217 = local write "New: Trap Density-STS"(w417) -> ()
        n218 = local read "Index"() -> (w464:string)
        n219 = local read "Wait Time (s):"() -> (w510:dbl)
        n220 = local write "New: Temp"(w416) -> ()
        n221 = String Subset(string=w450, length (rest)=1) -> (substring=w505:string)  [unwired: 1 in]
        n222 = local write "Row"(w505) -> ()
        n223 = local read "Treatment Concentration (mM):"() -> (w458:dbl)
        n224 = local read "Rec: Concentration"() -> (w445:dbl)
        n225 = local read "Relative Humidity (%):"() -> (w455:dbl)
        n226 = String Subset(string=w450, offset (0)=1, length (rest)=2) -> (substring=w506:string)
        n227 = Number To Decimal String(number=w510) -> (decimal integer string=w511:string)  [unwired: 1 in]
        n228 = local read "Solution Temp (C):"() -> (w499:dbl)
        n229 = local read "Surface Treatment:"() -> (w457:string)
        n230 = local read "Room Temp (F):"() -> (w503:dbl)
        n231 = local read "Rec: Material"() -> (w453:string)
        n232 = local write "Column"(w506) -> ()
        n233 = local read "New: Length"() -> (w463:dbl)
        n234 = local read "New: Width"() -> (w462:dbl)
        n235 = local read "New: Mobility-Sat"() -> (w492:dbl)
        n236 = local read "Accel (RPM/s):"() -> (w490:dbl)
        n237 = local read "Sample #:"() -> (w482:dbl)
        n238 = local read "# Drops*:"() -> (w500:dbl)
        n239 = local read "Ramp (s):"() -> (w508:dbl)
        n240 = local read "New: STS"() -> (w484:dbl)
        n241 = local read "Rec: Solvent"() -> (w459:string)
        n242 = local read "New: VT-Sat"() -> (w486:dbl)
        n243 = local read "Rec: On/Off"() -> (w488:dbl)
        n244 = local read "Rec: Method"() -> (w483:string)
        n245 = local read "Time (s):"() -> (w495:dbl)
        n246 = local read "Date Recorded"() -> (w479:string)
        n247 = local read "RPM:"() -> (w496:dbl)
        n248 = local read "Fabricator:"() -> (w504:string)
        n249 = Number To Decimal String(number=w445) -> (decimal integer string=w444:string)  [unwired: 1 in]
        n250 = Number To Decimal String(number=w500) -> (decimal integer string=w501:string)  [unwired: 1 in]
        n251 = Number To Decimal String(number=w482) -> (decimal integer string=w475:string)  [unwired: 1 in]
        n252 = call "DeviceID"("Sample"=w475, "Year"=w476, "Month"=w470, "Day"=w466, "Index"=w464) -> ("Result"=w481:string)  [unwired: 9 in, 1 out]
        n253 = Number To Decimal String(number=w463) -> (decimal integer string=w461:string)  [unwired: 1 in]
        n254 = Number To Decimal String(number=w462) -> (decimal integer string=w460:string)  [unwired: 1 in]
        n255 = Number To Decimal String(number=w499) -> (decimal integer string=w498:string)  [unwired: 1 in]
        n256 = Number To Decimal String(number=w455) -> (decimal integer string=w454:string)  [unwired: 1 in]
        n257 = Number To Decimal String(number=w503) -> (decimal integer string=w502:string)  [unwired: 1 in]
        n258 = property on="Image Out" class="ImageControl"() -> ("ZoomSingle"=w549:cluster{"X":sgl, "Y":sgl})  [unwired: 2 in, 2 out]
        n259 = Number To Decimal String(number=w458) -> (decimal integer string=w456:string)  [unwired: 1 in]
        n260 = property on="Image Out" class="ImageControl"() -> ("Bounds"=w550:T11)  [unwired: 2 in, 2 out]
        n261 = Number To Decimal String(number=w496) -> (decimal integer string=w497:string)  [unwired: 1 in]
        n262 = Number To Fractional String(number=w490) -> (F-format string=w491:string)  [unwired: 3 in]
        n263 = Number To Decimal String(number=w495) -> (decimal integer string=w494:string)  [unwired: 1 in]
        n264 = Number To Fractional String(number=w492) -> (F-format string=w493:string)  [unwired: 3 in]
        n265 = Number To Fractional String(number=w488) -> (F-format string=w489:string)  [unwired: 3 in]
        n266 = Number To Fractional String(number=w486) -> (F-format string=w487:string)  [unwired: 3 in]
        n267 = Number To Fractional String(number=w484) -> (F-format string=w485:string)  [unwired: 3 in]
        n268 = Number To Decimal String(number=w508) -> (decimal integer string=w509:string)  [unwired: 1 in]
        n269 = call <vilib>:"Intialize Keyboard.vi"() -> ("device ID"=w561:refnum<k1>)  [unwired: 10 in, 1 out]
        n270 = property on="Image Out" class="ImageControl"() -> ("Image Center Position"=w556:cluster{"X":u32, "Y":u32})  [unwired: 2 in, 2 out]
        n271 = call-poly <vilib>:"Acquire Input Data.vi"("device ID"=w561) -> ("keys pressed"=w560:T12)  [unwired: 16 in, 2 out]
        n272 = Unbundle(w550) -> ("Width"=w547:u32, "Height"=w546:u32)
        n273 = Unbundle(w549) -> ("X"=w524:sgl, "Y"=w548:sgl)
        n274 = Index Array(array=w560) -> (element=w564:T13)  [unwired: 1 in]
        n275 = event shown="[0] \"Remove Button\": Mouse Down" {
          selector: _ -> [_ _ _ _ _ _ _]
          dyn-events: _ -> [_ _ _ _ _ _ _]
          timeout: 10 -> [_ _ _ _ _ _ _]
          event "Remove Button": Mouse Down {
            w598 = 0
            n276 = event-data() -> ()  [unwired: 1 in, 7 out]
            n277 = property on="Image Out" class="ImageControl"() -> ("ROI"=w596:T10)  [unwired: 2 in, 2 out]
            n278 = Unbundle(w596) -> ("Global Rectangle"=w599:i32[], "Contours"=w601:T14)
            n279 = Reverse 1D Array(array=w599) -> (reversed array=w600:i32[])
            n280 = Reverse 1D Array(array=w601) -> (reversed array=w602:T14)
            n281 = Delete From Array(array=w600, index=w598) -> (array with subset deleted=w603:i32[])  [unwired: 1 in, 1 out]
            n282 = Delete From Array(array=w602, index=w598) -> (array with subset deleted=w604:T14)  [unwired: 1 in, 1 out]
            n283 = Reverse 1D Array(array=w603) -> (reversed array=w605:i32[])
            n284 = Reverse 1D Array(array=w604) -> (reversed array=w606:T14)
            n285 = Bundle(w605, w606) -> (w597:T15)  [unwired: 1 in]
            n286 = local write "ROI Descriptor out"(w596) -> ()
            n287 = local write "ROI Descriptor"(w597) -> ()
            n288 = property on="Image Out" class="ImageControl"("ROI"=w597) -> ()  [unwired: 2 in, 2 out]
          }
          event "Undo Button": Mouse Down {
            n289 = event-data() -> ()  [unwired: 1 in, 7 out]
            n290 = invoke on="Image Out" class="ImageControl" method="Clear ROI"() -> ()  [unwired: 3 in, 3 out]
          }
          event "Image Folder": Value Change {
            n291 = event-data() -> ()  [unwired: 1 in, 5 out]
            n292 = local read "Image File"() -> (w608:path)
            n293 = call "Vision Acquisition"("Image Path"=w608) -> ("Image Out"=w607:T2)  [unwired: 25 in, 1 out]
            n294 = local write "Image Out 2"(w607) -> ()
            n295 = local write "Image Out"(w607) -> ()
            n296 = invoke on="Image Out" class="ImageControl" method="Clear ROI"() -> ()  [unwired: 3 in, 3 out]
          }
          event "Zoom": Value Change {
            n297 = event-data() -> ()  [unwired: 1 in, 5 out]
            n298 = local read "Zoom"() -> (w609:i16)
            n299 = Bundle("Zoom"=w609, "Zoom"=w609) -> (w610:cluster{"Zoom":i16, "Zoom":i16})  [unwired: 1 in]
            n300 = property on="Image Out" class="ImageControl"("ZoomInteger"=w610) -> ()  [unwired: 2 in, 2 out]
          }
          event Timeout {
            n301 = event-data() -> ()  [unwired: 1 in, 2 out]
          }
          event "Image Out": Mouse Enter {
            (unwired) 6
            n302 = event-data() -> ()  [unwired: 1 in, 3 out]
            n303 = call "Simulate_Keyboard.vi"("Action"=0, "Virtual Key"=162) -> ()  [unwired: 7 in, 1 out]
          }
          event "Image Out": Mouse Leave {
            n304 = event-data() -> ()  [unwired: 1 in, 3 out]
            n305 = flat-sequence {
              frame #0 {
                n306 = Wait (ms)(milliseconds to wait=10) -> ()  [unwired: 1 out]
              }
              frame #1 {
                (unwired) 6
                n307 = call "Simulate_Keyboard.vi"("Action"=2, "Virtual Key"=162) -> ()  [unwired: 7 in, 1 out]
              }
            }
          }
        }
        n308 = Divide(x=w547, y=w524) -> (x/y=w537:sgl)
        n309 = Multiply(x=w537, y=0.5) -> (x*y=w543:dbl)
        n310 = Divide(x=w546, y=w548) -> (x/y=w536:sgl)
        n311 = Multiply(x=w536, y=0.5) -> (x*y=w542:dbl)
        n312 = Unbundle(w556) -> ("X"=w538:u32, "Y"=w539:u32)
        n313 = Subtract(x=w539, y=w542) -> (x-y=w540:dbl)
        n314 = Subtract(x=w538, y=w543) -> (x-y=w541:dbl)
        n315 = Add(x=w541, y=w537) -> (x+y=w555:dbl)
        n316 = Add(x=w540, y=w536) -> (x+y=w554:dbl)
        n317 = Build Array(w481, w504, w483, w479, w475, w505, w506, w461, w460, w453, w457, w456, w459, w444, w498, w501, w511, w502, w454, w509, w497, w491, w494, w493, w489, w487, w485) -> (w507:string[])
        n318 = local write "Current \nRecord"(w507) -> ()
        n319 = Reciprocal(x=w524) -> (1/x=w523:sgl)
        n320 = event shown="[1] \"Down Button\": Mouse Down" {
          selector: _ -> [_ _ _ _ _ _ _ _ _ _ _ _ _ _ _ _]
          dyn-events: _ -> [_ _ _ _ _ _ _ _ _ _ _ _ _ _ _ _]
          timeout: 10 -> [_ _ _ _ _ _ _ _ _ _ _ _ _ _ _ _]
          tunnel: [_ _ _ _ _ _ _ _ _ _ _ _ _ TRUE _ TRUE] -> w581
          event Timeout {
            n321 = event-data() -> ()  [unwired: 1 in, 2 out]
          }
          event "Down Button": Mouse Down {
            w950 = 0
            n322 = event-data() -> ()  [unwired: 1 in, 7 out]
            n323 = local read "Data File"() -> (w955:path)
            n324 = Strip Path(path=w955) -> (stripped path=w946:path, name=w964:string)
            n325 = local write "Data Folder"(w946) -> ()
            n326 = List Folder(path=w946) -> (filenames=w960:string[], error out=w900:errorcluster)  [unwired: 3 in, 2 out]
            n327 = local read "Folder Index"() -> (w902:dbl)
            n328 = property on="Image Out" class="ImageControl"() -> (error out=w903:errorcluster, "Image Center Position"=w907:cluster{"X":u32, "Y":u32})  [unwired: 2 in, 1 out]
            n329 = Array Size(array=w960) -> (size(s)=w956:i32)
            n330 = Search 1D Array(1D array=w960, element=w964) -> (index of element=w957:i32)  [unwired: 1 in]
            n331 = Decrement(x=w956) -> (x-1=w958:i32)
            n332 = Equal?(x=w957, y=w958) -> (x = y?=w959:bool)
            n333 = invoke on="Image Out" class="ImageControl" method="Clear ROI"() -> ()  [unwired: 3 in, 3 out]
            n334 = case shown="False" w959 {
              tunnel: w902 -> [w1117 _]
              tunnel: [w1116 0] -> w901
              tunnel: w900 -> [w1115 w1118]
              tunnel: [w1115 w1118] -> w899
              frame False {
                n335 = Increment(x=w1117) -> (x+1=w1116:dbl)
              }
              frame True {
              }
            }
            n336 = Unbundle(w907) -> ("X"=w905:u32)  [unwired: 1 out]
            n337 = local write "Folder Index"(w901) -> ()
            n338 = Bundle("X"=w905, 0) -> (w906:cluster{"X":u32, i32})  [unwired: 1 in]
            n339 = property on="Image Out" class="ImageControl"(error in=w903, "Image Center Position"=w906) -> ()  [unwired: 1 in, 2 out]
            n340 = Path To String(path=w946) -> (string=w965:string)
            n341 = Index Array(array=w960, index=w901) -> (element=w961:string)
            n342 = local write "Data Name:"(w961) -> ()
            n343 = Concatenate Strings(w965, "\\", w961) -> (w963:string)
            n344 = String To Path(string=w963) -> (path=w873:path)
            n345 = call "Recorded Values.vi"("Path"=w873) -> ("Recorded Char"=w967:T5, "Recorded Prop"=w968:T6, "Fabrication Prop"=w966:T7)  [unwired: 8 in]
            n346 = Unbundle By Name(w967) -> ("Mobility-Sat"=w980:dbl, "Moblitity-Lin"=w981:dbl, "On/Off"=w982:dbl, "Off Current"=w983:dbl, "Vt-Sat"=w868:dbl, "STS"=w984:dbl, "Trap Density-VT"=w985:dbl, "Trap Density-STS"=w986:dbl)
            n347 = Unbundle By Name(w966) -> ("Date Created"=w987:string, "Material"=w969:string, "Solvent"=w970:string, "Concentration"=w971:dbl, "Method"=w972:string, "Dielectric (nm)"=w973:dbl, "Treatment"=w974:string, "Comments"=w975:string)
            n348 = Unbundle By Name(w968) -> ("Date Recorded"=w976:string, "Index"=w977:string, "Length"=w978:dbl, "Width"=w979:dbl, "Sample Temp"=w870:dbl)
            n349 = local write "Date Created"(w987) -> ()
            n350 = local write "Rec: Off I-Sat"(w983) -> ()
            n351 = local write "Rec: Material"(w969) -> ()
            n352 = local write "Rec: VT-Sat"(w868) -> ()
            n353 = local write "Rec: Concentration"(w971) -> ()
            n354 = local write "Rec: Method"(w972) -> ()
            n355 = local write "Rec: Dielectric (d)"(w973) -> ()
            n356 = local write "Surface Treatment:"(w974) -> ()
            n357 = local write "Comments"(w975) -> ()
            n358 = local write "Index"(w977) -> ()
            n359 = local write "Rec: Mobility-Sat"(w980) -> ()
            n360 = local write "Rec: Mobility-Lin"(w981) -> ()
            n361 = local write "Rec: On/Off"(w982) -> ()
            n362 = local write "Rec: STS"(w984) -> ()
            n363 = local write "Rec: Trap Density-VT"(w985) -> ()
            n364 = local write "Rec: Trap Density-STS"(w986) -> ()
            n365 = local write "Rec: Solvent"(w970) -> ()
            n366 = local write "Date Recorded"(w976) -> ()
            n367 = local write "Rec: Length"(w978) -> ()
            n368 = local write "Rec: Width"(w979) -> ()
            n369 = local write "Rec: Temp"(w870) -> ()
            n370 = Equal To 0?(x=w870) -> (x = 0?=w871:bool)
            n371 = case shown="True" w871 {
              tunnel: [w988 w989] -> w869
              tunnel: w870 -> [w988 _]
              frame False {
              }
              frame True {
                n372 = local read "Room Temp"() -> (w989:dbl)
              }
            }
            n373 = local read "NumPts 2"() -> (w894:dbl)
            n374 = local read "NumPts"() -> (w898:dbl)
            n375 = local write "Data File"(w873) -> ()
            n376 = call-poly <vilib>:"Read From Spreadsheet File.vi"("file path (dialog if empty)"=w873) -> ("all rows"=w952:string[][])  [unwired: 6 in, 4 out]
            n377 = call "Mobility-Vt Calculator-File.vi"("NumPts"=w898, "Path"=w873) -> ("XY Graph-Sat"=w896:cluster{dbl[], dbl[]}[], "XY Graph-Lin"=w867:cluster{dbl[], dbl[]}[], "Output"=w897:T8, "Index-Sat"=w895:dbl, "Index-Lin"=w881:dbl)  [unwired: 4 in, 1 out]
            n378 = local read "New: Dielectric"() -> (w878:dbl)
            n379 = call "STS Calculator-File.vi"("NumPts"=w894, "Path"=w873) -> ("STS Index-Sat"=w893:dbl, "XY Graph-Sat"=w892:cluster{dbl[], dbl[]}[], "Ouput"=w891:cluster{"STS-Sat":dbl, "STS-Lin":dbl})  [unwired: 5 in, 2 out]
            n380 = Unbundle By Name(w897) -> ("Mobility-Sat"=w890:dbl, "Vt-Sat"=w877:dbl, "Mobility-Lin"=w889:dbl, "Vt-Lin"=w888:dbl, "Off I-Sat"=w874:dbl, "On/Off I-Sat"=w866:dbl)
            n381 = Unbundle By Name(w891) -> ("STS-Sat"=w872:dbl)  [unwired: 1 out]
            n382 = local write "Index 2"(w893) -> ()
            n383 = local write "XY Graph 2"(w892) -> ()
            n384 = local write "MobVi Index"(w895) -> ()
            n385 = local write "Slide"(w895) -> ()
            n386 = local write "XY Graph"(w896) -> ()
            n387 = Array Size(array=w952) -> (size(s)=w951:i32[])
            n388 = call "Trap Density_VT.vi"("VT"=w877, "Dielectric"=w878) -> ("Trap Density-VT"=w876:dbl)
            n389 = call "Trap Density_STS.vi"("Temp (T) [K]"=w869, "S.T.S. (S)"=w872, "Dielectric"=w878) -> ("Trap Density (N)"=w875:dbl)  [unwired: 8 in]
            n390 = local write "New: STS"(w872) -> ()
            n391 = local write "Calc: STS"(w872) -> ()
            n392 = local write "Calc: Mobility-Sat"(w890) -> ()
            n393 = local write "Calc: Off I-Sat"(w888) -> ()
            n394 = local write "Calc: Mobility-Lin"(w889) -> ()
            n395 = Index Array(array=w951, index=w950) -> (element=w932:i32)
            n396 = Decimate 1D Array(w892) -> (w926:cluster{dbl[], dbl[]}[])  [unwired: 1 out]
            n397 = Decimate 1D Array(w896) -> (w936:cluster{dbl[], dbl[]}[])  [unwired: 1 out]
            n398 = local write "Calc: Off I-Sat"(w874) -> ()
            n399 = local write "Calc: On/Off"(w866) -> ()
            n400 = Decimate 1D Array(w867) -> (w887:cluster{dbl[], dbl[]}[])  [unwired: 1 out]
            n401 = local write "Calc: VT-Sat"(w877) -> ()
            n402 = Array Subset(array=w952, index (row)=w950, index (col)=w950, length (col)=3) -> (w953:string[][])  [unwired: 1 in]
            n403 = local write "Calc: Trap Density-VT"(w876) -> ()
            n404 = local write "Calc: Trap Density-STS"(w875) -> ()
            n405 = local write "New: Trap Density-STS"(w875) -> ()
            n406 = local write "New: Trap Density-VT"(w876) -> ()
            n407 = local write "XY Graph-Lin"(w867) -> ()
            n408 = Array To Cluster(array=w926) -> (cluster=w924:T9)
            n409 = Array To Cluster(array=w936) -> (cluster=w938:T9)
            n410 = local write "New: VT-Lin"(w888) -> ()
            n411 = local write "New: VT-Sat"(w877) -> ()
            n412 = local write "New: Mobility-Sat"(w890) -> ()
            n413 = local write "New: Mobility-Lin"(w889) -> ()
            n414 = Reshape Array(w953, w932) -> (w939:string[])
            n415 = Array To Cluster(array=w887) -> (cluster=w886:T9)
            n416 = Subtract(x=w932, y=20) -> (x-y=w931:i32)
            n417 = property on="Slide" class="Slide (strict)"("Scale.Maximum"=w931) -> ()  [unwired: 2 in, 2 out]
            n418 = Unbundle(w924) -> ("[0]"=w925:cluster{dbl[], dbl[]})  [unwired: 8 out]
            n419 = Unbundle(w938) -> ("[0]"=w937:cluster{dbl[], dbl[]})  [unwired: 8 out]
            n420 = Unbundle(w886) -> ("[0]"=w883:cluster{dbl[], dbl[]})  [unwired: 8 out]
            n421 = Search 1D Array(1D array=w939, element="Index:") -> (index of element=w947:i32)  [unwired: 1 in]
            n422 = local read "NumPts"() -> (w882:dbl)
            n423 = Unbundle(w883) -> (w885:dbl[], w884:dbl[])
            n424 = Increment(x=w947) -> (x+1=w948:i32)
            n425 = Unbundle(w925) -> (w923:dbl[], w922:dbl[])
            n426 = Unbundle(w937) -> (w928:dbl[], w927:dbl[])
            n427 = Array Subset(array=w885, index=w881, length=w882) -> (w880:dbl[])
            n428 = Array Subset(array=w884, index=w881, length=w882) -> (w879:dbl[])
            n429 = Array Subset(array=w923, index=w893, length=w894) -> (w930:dbl[])
            n430 = Array Subset(array=w922, index=w893, length=w894) -> (w929:dbl[])
            n431 = Array Subset(array=w928, index=w895, length=w898) -> (w935:dbl[])
            n432 = Array Subset(array=w927, index=w895, length=w898) -> (w934:dbl[])
            n433 = Index Array(array=w939, index=w948) -> (element=w911:string)
            n434 = local write "Lin-Vg Array-Used"(w880) -> ()
            n435 = local write "Sat Vg Array-Used"(w935) -> ()
            n436 = local write "Vg Array-Log-Used"(w929) -> ()
            n437 = local write "Lin Id-Used"(w879) -> ()
            n438 = local read "Image Folder"() -> (w909:path)
            n439 = local write "Sat Id-Used"(w934) -> ()
            n440 = local write "Sat Id-Log-Used"(w930) -> ()
            n441 = List Folder(path=w909, error in=w899) -> (filenames=w945:string[], error out=w912:errorcluster)  [unwired: 2 in, 2 out]
            n442 = while {
              tunnel: w945 -> [w1002]
              tunnel: w911 -> [w1000]
              tunnel: [w999] -> _
              tunnel: [w999] -> w944
              tunnel: w932 -> [w998]
              i -> [w999]
              stop <- w995 stop-if-true
              n443 = Index Array(array=w1002, index=w999) -> (element=w1003:string)
              n444 = xnode "Match Regular Expression"("input string"=w1003, "regular expression"=w1000) -> ("whole match"=w1001:string)  [unwired: 4 in, 4 out]
              n445 = Equal?(x=w1001, y=w1000) -> (x = y?=w997:bool)
              n446 = Equal?(x=w998, y=w999) -> (x = y?=w996:bool)
              n447 = Or(x=w997, y=w996) -> (x .or. y?=w995:bool)
            }
            n448 = Build Path(base path=w909, name or relative path="ROI") -> (appended path=w908:path)
            n449 = Path To String(path=w909) -> (string=w942:string)
            n450 = Index Array(array=w945, index=w944) -> (element=w920:string)
            n451 = invoke on="Image Out" class="ImageControl" method="Clear ROI"(error in=w912) -> (error out=w915:errorcluster)  [unwired: 2 in, 2 out]
            n452 = local write "Image Name"(w920) -> ()
            n453 = Build Path(base path=w908, name or relative path=w911) -> (appended path=w916:path)
            n454 = call <vilib>:"Check if File or Folder Exists.vi"("error in (no error)"=w915, "path"=w916) -> ("file or folder exists?"=w913:bool, "dup path"=w914:path)  [unwired: 7 in, 1 out]
            n455 = Concatenate Strings(w942, "\\", w920) -> (w941:string)
            n456 = case shown="False" w913 {
              tunnel: w914 -> [_ w990]
              frame False {
              }
              frame True {
                n457 = Read from Text File(file (use dialog)=w990) -> (text=w994:string)  [unwired: 3 in, 3 out]
                n458 = property on="Image Out" class="ImageControl"() -> ("ROI"=w991:T10)  [unwired: 2 in, 2 out]
                n459 = Unflatten From String(type=w991, binary string=w994) -> (value=w992:T10, error out=w993:errorcluster)  [unwired: 3 in, 1 out]
                n460 = property on="Image Out" class="ImageControl"(error in=w993, "ROI"=w992) -> ()  [unwired: 1 in, 2 out]
              }
            }
            n461 = String To Path(string=w941) -> (path=w919:path)
            n462 = Empty String/Path?(string/path=w920) -> (empty?=w921:bool)
            n463 = local read "No Image"() -> (w917:path)
            n464 = Select(t=w917, s=w921, f=w919) -> (s? t:f=w918:path)
            n465 = local write "Image File"(w918) -> ()
            n466 = call "Vision Acquisition4"("Image Path"=w918) -> ("Image Out"=w943:T2)  [unwired: 25 in, 1 out]
            n467 = local write "Image Out"(w943) -> ()
            n468 = local write "Image Out 2"(w943) -> ()
          }
          event "Data File": Value Change {
            w1226 = 0
            n469 = event-data() -> ()  [unwired: 1 in, 5 out]
            n470 = local read "Data File"() -> (w1222:path)
            n471 = Strip Path(path=w1222) -> (stripped path=w1221:path, name=w1235:string)
            n472 = local write "Data Folder"(w1221) -> ()
            n473 = property on="Image Out" class="ImageControl"() -> (error out=w1177:errorcluster, "Image Center Position"=w1181:cluster{"X":u32, "Y":u32})  [unwired: 2 in, 1 out]
            n474 = List Folder(path=w1221) -> (filenames=w1231:string[], error out=w1187:errorcluster)  [unwired: 3 in, 2 out]
            n475 = Search 1D Array(1D array=w1231, element=w1235) -> (index of element=w1176:i32)  [unwired: 1 in]
            n476 = local write "Folder Index"(w1176) -> ()
            n477 = Unbundle(w1181) -> ("X"=w1179:u32)  [unwired: 1 out]
            n478 = Path To String(path=w1221) -> (string=w1236:string)
            n479 = Index Array(array=w1231, index=w1176) -> (element=w1232:string)
            n480 = Bundle("X"=w1179, 0) -> (w1180:cluster{"X":u32, i32})  [unwired: 1 in]
            n481 = local write "Data Name:"(w1232) -> ()
            n482 = property on="Image Out" class="ImageControl"(error in=w1177, "Image Center Position"=w1180) -> ()  [unwired: 1 in, 2 out]
            n483 = Concatenate Strings(w1236, "\\", w1232) -> (w1234:string)
            n484 = String To Path(string=w1234) -> (path=w1127:path)
            n485 = call "Recorded Values.vi"("Path"=w1127) -> ("Recorded Char"=w1174:T5, "Recorded Prop"=w1173:T6, "Fabrication Prop"=w1175:T7)  [unwired: 8 in]
            n486 = Unbundle By Name(w1174) -> ("Mobility-Sat"=w1161:dbl, "Moblitity-Lin"=w1160:dbl, "On/Off"=w1159:dbl, "Off Current"=w1158:dbl, "Vt-Sat"=w1123:dbl, "STS"=w1157:dbl, "Trap Density-VT"=w1156:dbl, "Trap Density-STS"=w1155:dbl)
            n487 = Unbundle By Name(w1175) -> ("Date Created"=w1154:string, "Material"=w1172:string, "Solvent"=w1171:string, "Concentration"=w1170:dbl, "Method"=w1169:string, "Dielectric (nm)"=w1168:dbl, "Treatment"=w1167:string, "Comments"=w1166:string)
            n488 = Unbundle By Name(w1173) -> ("Date Recorded"=w1165:string, "Index"=w1164:string, "Length"=w1163:dbl, "Width"=w1162:dbl, "Sample Temp"=w1125:dbl)
            n489 = local write "Date Created"(w1154) -> ()
            n490 = local write "Rec: Material"(w1172) -> ()
            n491 = local write "Rec: Off I-Sat"(w1158) -> ()
            n492 = local write "Rec: VT-Sat"(w1123) -> ()
            n493 = local write "Rec: Concentration"(w1170) -> ()
            n494 = local write "Rec: Method"(w1169) -> ()
            n495 = local write "Rec: Dielectric (d)"(w1168) -> ()
            n496 = local write "Surface Treatment:"(w1167) -> ()
            n497 = local write "Comments"(w1166) -> ()
            n498 = local write "Index"(w1164) -> ()
            n499 = local write "Rec: Mobility-Sat"(w1161) -> ()
            n500 = local write "Rec: Mobility-Lin"(w1160) -> ()
            n501 = local write "Rec: On/Off"(w1159) -> ()
            n502 = local write "Rec: STS"(w1157) -> ()
            n503 = local write "Rec: Trap Density-VT"(w1156) -> ()
            n504 = local write "Rec: Trap Density-STS"(w1155) -> ()
            n505 = local write "Rec: Solvent"(w1171) -> ()
            n506 = local write "Date Recorded"(w1165) -> ()
            n507 = local write "Rec: Length"(w1163) -> ()
            n508 = local write "Rec: Width"(w1162) -> ()
            n509 = local write "Rec: Temp"(w1125) -> ()
            n510 = Equal To 0?(x=w1125) -> (x = 0?=w1126:bool)
            n511 = case shown="False" w1126 {
              tunnel: [w1237 w1238] -> w1124
              tunnel: w1125 -> [w1237 _]
              frame False {
              }
              frame True {
                n512 = local read "Room Temp"() -> (w1238:dbl)
              }
            }
            n513 = local read "NumPts 2"() -> (w1149:dbl)
            n514 = local write "Data File"(w1127) -> ()
            n515 = local read "NumPts"() -> (w1150:dbl)
            n516 = call-poly <vilib>:"Read From Spreadsheet File.vi"("file path (dialog if empty)"=w1127) -> ("all rows"=w1228:string[][])  [unwired: 6 in, 4 out]
            n517 = local read "New: Dielectric"() -> (w1133:dbl)
            n518 = call "STS Calculator-File.vi"("NumPts"=w1149, "Path"=w1127) -> ("STS Index-Sat"=w1147:dbl, "XY Graph-Sat"=w1148:cluster{dbl[], dbl[]}[], "Ouput"=w1146:cluster{"STS-Sat":dbl, "STS-Lin":dbl})  [unwired: 5 in, 2 out]
            n519 = call "Mobility-Vt Calculator-File.vi"("NumPts"=w1150, "Path"=w1127) -> ("XY Graph-Sat"=w1153:cluster{dbl[], dbl[]}[], "XY Graph-Lin"=w1122:cluster{dbl[], dbl[]}[], "Output"=w1151:T8, "Index-Sat"=w1152:dbl, "Index-Lin"=w1139:dbl)  [unwired: 4 in, 1 out]
            n520 = Unbundle By Name(w1151) -> ("Mobility-Sat"=w1135:dbl, "Vt-Sat"=w1129:dbl, "Mobility-Lin"=w1134:dbl, "Vt-Lin"=w1120:dbl, "Off I-Sat"=w1128:dbl, "On/Off I-Sat"=w1121:dbl)
            n521 = local write "Index 2"(w1147) -> ()
            n522 = local write "XY Graph 2"(w1148) -> ()
            n523 = Unbundle By Name(w1146) -> ("STS-Sat"=w1130:dbl)  [unwired: 1 out]
            n524 = local write "MobVi Index"(w1152) -> ()
            n525 = Array Size(array=w1228) -> (size(s)=w1227:i32[])
            n526 = call "Trap Density_VT.vi"("VT"=w1129, "Dielectric"=w1133) -> ("Trap Density-VT"=w1132:dbl)
            n527 = call "Trap Density_STS.vi"("Temp (T) [K]"=w1124, "S.T.S. (S)"=w1130, "Dielectric"=w1133) -> ("Trap Density (N)"=w1131:dbl)  [unwired: 8 in]
            n528 = local write "Slide"(w1152) -> ()
            n529 = local write "Calc: Mobility-Lin"(w1134) -> ()
            n530 = local write "Calc: Mobility-Sat"(w1135) -> ()
            n531 = local write "Calc: VT-Sat"(w1129) -> ()
            n532 = local write "Calc: Off I-Sat"(w1128) -> ()
            n533 = local write "Calc: VT-Lin"(w1120) -> ()
            n534 = local write "Calc: On/Off"(w1121) -> ()
            n535 = local write "Calc: STS"(w1130) -> ()
            n536 = Decimate 1D Array(w1122) -> (w1145:cluster{dbl[], dbl[]}[])  [unwired: 1 out]
            n537 = local write "Calc: Trap Density-VT"(w1132) -> ()
            n538 = local write "Calc: Trap Density-STS"(w1131) -> ()
            n539 = local write "New: Trap Density-STS"(w1131) -> ()
            n540 = local write "New: Trap Density-VT"(w1132) -> ()
            n541 = local write "XY Graph-Lin"(w1122) -> ()
            n542 = local write "New: VT-Sat"(w1129) -> ()
            n543 = Decimate 1D Array(w1148) -> (w1202:cluster{dbl[], dbl[]}[])  [unwired: 1 out]
            n544 = Index Array(array=w1227, index=w1226) -> (element=w1208:i32)
            n545 = Decimate 1D Array(w1153) -> (w1211:cluster{dbl[], dbl[]}[])  [unwired: 1 out]
            n546 = local write "XY Graph"(w1153) -> ()
            n547 = local write "New: Mobility-Lin"(w1134) -> ()
            n548 = Array Subset(array=w1228, index (row)=w1226, index (col)=w1226, length (col)=3) -> (w1229:string[][])  [unwired: 1 in]
            n549 = local write "New: VT-Lin"(w1120) -> ()
            n550 = Array To Cluster(array=w1145) -> (cluster=w1144:T9)
            n551 = local write "New: STS"(w1130) -> ()
            n552 = local write "New: Mobility-Sat"(w1135) -> ()
            n553 = Array To Cluster(array=w1202) -> (cluster=w1200:T9)
            n554 = Array To Cluster(array=w1211) -> (cluster=w1213:T9)
            n555 = Reshape Array(w1229, w1208) -> (w1214:string[])
            n556 = Subtract(x=w1208, y=20) -> (x-y=w1206:i32)
            n557 = Unbundle(w1144) -> ("[0]"=w1143:cluster{dbl[], dbl[]})  [unwired: 8 out]
            n558 = property on="Slide" class="Slide (strict)"("Scale.Maximum"=w1206) -> ()  [unwired: 2 in, 2 out]
            n559 = local read "NumPts"() -> (w1140:dbl)
            n560 = Unbundle(w1143) -> (w1142:dbl[], w1141:dbl[])
            n561 = Unbundle(w1200) -> ("[0]"=w1201:cluster{dbl[], dbl[]})  [unwired: 8 out]
            n562 = Unbundle(w1213) -> ("[0]"=w1212:cluster{dbl[], dbl[]})  [unwired: 8 out]
            n563 = Search 1D Array(1D array=w1214, element="Index:") -> (index of element=w1223:i32)  [unwired: 1 in]
            n564 = local read "NumPts"() -> (w1136:dbl)
            n565 = Array Subset(array=w1142, index=w1139, length=w1140) -> (w1138:dbl[])
            n566 = Array Subset(array=w1141, index=w1139, length=w1140) -> (w1137:dbl[])
            n567 = Increment(x=w1223) -> (x+1=w1224:i32)
            n568 = Unbundle(w1201) -> (w1198:dbl[], w1197:dbl[])
            n569 = Unbundle(w1212) -> (w1199:dbl[], w1203:dbl[])
            n570 = local read "Image Folder"() -> (w1183:path)
            n571 = local write "Lin-Vg Array-Used"(w1138) -> ()
            n572 = Array Subset(array=w1198, index=w1147, length=w1149) -> (w1205:dbl[])
            n573 = Array Subset(array=w1197, index=w1147, length=w1149) -> (w1204:dbl[])
            n574 = Array Subset(array=w1199, index=w1152, length=w1136) -> (w1210:dbl[])
            n575 = Array Subset(array=w1203, index=w1152, length=w1136) -> (w1209:dbl[])
            n576 = Index Array(array=w1214, index=w1224) -> (element=w1185:string)
            n577 = local write "Lin Id-Used"(w1137) -> ()
            n578 = local write "Sat Vg Array-Used"(w1210) -> ()
            n579 = local write "Vg Array-Log-Used"(w1204) -> ()
            n580 = local write "Sat Id-Log-Used"(w1205) -> ()
            n581 = local write "Sat Id-Used"(w1209) -> ()
            n582 = local write "Index"(w1185) -> ()
            n583 = List Folder(path=w1183, error in=w1187) -> (filenames=w1219:string[], error out=w1186:errorcluster)  [unwired: 2 in, 2 out]
            n584 = Build Path(base path=w1183, name or relative path="ROI") -> (appended path=w1182:path)
            n585 = while {
              tunnel: w1219 -> [w1251]
              tunnel: w1185 -> [w1249]
              tunnel: [w1248] -> _
              tunnel: [w1248] -> w1218
              tunnel: w1208 -> [w1247]
              i -> [w1248]
              stop <- w1244 stop-if-true
              n586 = Index Array(array=w1251, index=w1248) -> (element=w1252:string)
              n587 = xnode "Match Regular Expression"("input string"=w1252, "regular expression"=w1249) -> ("whole match"=w1250:string)  [unwired: 4 in, 4 out]
              n588 = Equal?(x=w1250, y=w1249) -> (x = y?=w1246:bool)
              n589 = Equal?(x=w1247, y=w1248) -> (x = y?=w1245:bool)
              n590 = Or(x=w1246, y=w1245) -> (x .or. y?=w1244:bool)
            }
            n591 = invoke on="Image Out" class="ImageControl" method="Clear ROI"(error in=w1186) -> (error out=w1190:errorcluster)  [unwired: 2 in, 2 out]
            n592 = Build Path(base path=w1182, name or relative path=w1185) -> (appended path=w1191:path)
            n593 = call <vilib>:"Check if File or Folder Exists.vi"("error in (no error)"=w1190, "path"=w1191) -> ("file or folder exists?"=w1188:bool, "dup path"=w1189:path)  [unwired: 7 in, 1 out]
            n594 = case shown="True" w1188 {
              tunnel: w1189 -> [_ w1239]
              frame False {
              }
              frame True {
                n595 = Read from Text File(file (use dialog)=w1239) -> (text=w1243:string)  [unwired: 3 in, 3 out]
                n596 = property on="Image Out" class="ImageControl"() -> ("ROI"=w1240:T10)  [unwired: 2 in, 2 out]
                n597 = Unflatten From String(type=w1240, binary string=w1243) -> (value=w1241:T10, error out=w1242:errorcluster)  [unwired: 3 in, 1 out]
                n598 = property on="Image Out" class="ImageControl"(error in=w1242, "ROI"=w1241) -> ()  [unwired: 1 in, 2 out]
              }
            }
            n599 = invoke on="Image Out" class="ImageControl" method="Clear ROI"() -> ()  [unwired: 3 in, 3 out]
            n600 = Path To String(path=w1183) -> (string=w1217:string)
            n601 = Index Array(array=w1219, index=w1218) -> (element=w1195:string)
            n602 = Concatenate Strings(w1217, "\\", w1195) -> (w1216:string)
            n603 = local write "Image Name"(w1195) -> ()
            n604 = String To Path(string=w1216) -> (path=w1194:path)
            n605 = Empty String/Path?(string/path=w1195) -> (empty?=w1196:bool)
            n606 = local read "No Image"() -> (w1192:path)
            n607 = Select(t=w1192, s=w1196, f=w1194) -> (s? t:f=w1193:path)
            n608 = local write "Image File"(w1193) -> ()
            n609 = call "Vision Acquisition3"("Image Path"=w1193) -> ("Image Out"=w1220:T2)  [unwired: 25 in, 1 out]
            n610 = local write "Image Out"(w1220) -> ()
            n611 = local write "Image Out 2"(w1220) -> ()
          }
          event "Up Button": Mouse Down {
            w1471 = 0
            n612 = event-data() -> ()  [unwired: 1 in, 5 out]
            n613 = local read "Data File"() -> (w1467:path)
            n614 = Strip Path(path=w1467) -> (stripped path=w1466:path, name=w1482:string)
            n615 = local write "Data Folder"(w1466) -> ()
            n616 = List Folder(path=w1466) -> (filenames=w1476:string[], error out=w1433:errorcluster)  [unwired: 3 in, 2 out]
            n617 = Array Size(array=w1476) -> (size(s)=w1421:i32)
            n618 = Search 1D Array(1D array=w1476, element=w1482) -> (index of element=w1477:i32)  [unwired: 1 in]
            n619 = Equal To 0?(x=w1477) -> (x = 0?=w1478:bool)
            n620 = local read "Folder Index"() -> (w1420:dbl)
            n621 = property on="Image Out" class="ImageControl"() -> (error out=w1423:errorcluster, "Image Center Position"=w1427:cluster{"X":u32, "Y":u32})  [unwired: 2 in, 1 out]
            n622 = case shown="True" w1478 {
              tunnel: w1420 -> [w1612 _]
              tunnel: [w1611 w1613] -> w1419
              tunnel: w1421 -> [_ w1614]
              frame False {
                n623 = Decrement(x=w1612) -> (x-1=w1611:dbl)
              }
              frame True {
                n624 = Decrement(x=w1614) -> (x-1=w1613:i32)
              }
            }
            n625 = Unbundle(w1427) -> ("X"=w1425:u32)  [unwired: 1 out]
            n626 = local write "Folder Index"(w1419) -> ()
            n627 = Bundle("X"=w1425, 0) -> (w1426:cluster{"X":u32, i32})  [unwired: 1 in]
            n628 = Path To String(path=w1466) -> (string=w1483:string)
            n629 = Index Array(array=w1476, index=w1419) -> (element=w1479:string)
            n630 = local write "Data Name:"(w1479) -> ()
            n631 = property on="Image Out" class="ImageControl"(error in=w1423, "Image Center Position"=w1426) -> ()  [unwired: 1 in, 2 out]
            n632 = Concatenate Strings(w1483, "\\", w1479) -> (w1481:string)
            n633 = String To Path(string=w1481) -> (path=w1370:path)
            n634 = call "Recorded Values.vi"("Path"=w1370) -> ("Recorded Char"=w1417:T5, "Recorded Prop"=w1416:T6, "Fabrication Prop"=w1418:T7)  [unwired: 8 in]
            n635 = Unbundle By Name(w1417) -> ("Mobility-Sat"=w1404:dbl, "Moblitity-Lin"=w1403:dbl, "On/Off"=w1402:dbl, "Off Current"=w1401:dbl, "Vt-Sat"=w1366:dbl, "STS"=w1400:dbl, "Trap Density-VT"=w1399:dbl, "Trap Density-STS"=w1398:dbl)
            n636 = Unbundle By Name(w1418) -> ("Date Created"=w1397:string, "Material"=w1415:string, "Solvent"=w1414:string, "Concentration"=w1413:dbl, "Method"=w1412:string, "Dielectric (nm)"=w1411:dbl, "Treatment"=w1410:string, "Comments"=w1409:string)
            n637 = Unbundle By Name(w1416) -> ("Date Recorded"=w1408:string, "Index"=w1407:string, "Length"=w1406:dbl, "Width"=w1405:dbl, "Sample Temp"=w1367:dbl)
            n638 = local write "Date Created"(w1397) -> ()
            n639 = local write "Rec: Material"(w1415) -> ()
            n640 = local write "Rec: Off I-Sat"(w1401) -> ()
            n641 = local write "Rec: VT-Sat"(w1366) -> ()
            n642 = local write "Rec: Solvent"(w1414) -> ()
            n643 = local write "Rec: Concentration"(w1413) -> ()
            n644 = local write "Rec: Method"(w1412) -> ()
            n645 = local write "Rec: Dielectric (d)"(w1411) -> ()
            n646 = local write "Surface Treatment:"(w1410) -> ()
            n647 = local write "Comments"(w1409) -> ()
            n648 = local write "Index"(w1407) -> ()
            n649 = local write "Rec: Mobility-Sat"(w1404) -> ()
            n650 = local write "Rec: Mobility-Lin"(w1403) -> ()
            n651 = local write "Rec: On/Off"(w1402) -> ()
            n652 = local write "Rec: STS"(w1400) -> ()
            n653 = local write "Rec: Trap Density-VT"(w1399) -> ()
            n654 = local write "Rec: Trap Density-STS"(w1398) -> ()
            n655 = local write "Date Recorded"(w1408) -> ()
            n656 = local write "Rec: Length"(w1406) -> ()
            n657 = local write "Rec: Width"(w1405) -> ()
            n658 = local write "Rec: Temp"(w1367) -> ()
            n659 = Equal To 0?(x=w1367) -> (x = 0?=w1369:bool)
            n660 = case shown="False" w1369 {
              tunnel: [w1484 w1485] -> w1368
              tunnel: w1367 -> [w1484 _]
              frame False {
              }
              frame True {
                n661 = local read "Room Temp"() -> (w1485:dbl)
              }
            }
            n662 = local read "NumPts 2"() -> (w1392:dbl)
            n663 = local write "Data File"(w1370) -> ()
            n664 = local read "NumPts"() -> (w1396:dbl)
            n665 = local read "New: Dielectric"() -> (w1376:dbl)
            n666 = call "Mobility-Vt Calculator-File.vi"("NumPts"=w1396, "Path"=w1370) -> ("XY Graph-Sat"=w1394:cluster{dbl[], dbl[]}[], "XY Graph-Lin"=w1365:cluster{dbl[], dbl[]}[], "Output"=w1395:T8, "Index-Sat"=w1393:dbl, "Index-Lin"=w1380:dbl)  [unwired: 4 in, 1 out]
            n667 = call "STS Calculator-File.vi"("NumPts"=w1392, "Path"=w1370) -> ("STS Index-Sat"=w1391:dbl, "XY Graph-Sat"=w1390:cluster{dbl[], dbl[]}[], "Ouput"=w1389:cluster{"STS-Sat":dbl, "STS-Lin":dbl})  [unwired: 5 in, 2 out]
            n668 = call-poly <vilib>:"Read From Spreadsheet File.vi"("file path (dialog if empty)"=w1370) -> ("all rows"=w1473:string[][])  [unwired: 6 in, 4 out]
            n669 = Unbundle By Name(w1395) -> ("Mobility-Sat"=w1379:dbl, "Vt-Sat"=w1372:dbl, "Mobility-Lin"=w1378:dbl, "Vt-Lin"=w1377:dbl, "Off I-Sat"=w1371:dbl, "On/Off I-Sat"=w1364:dbl)
            n670 = Unbundle By Name(w1389) -> ("STS-Sat"=w1373:dbl)  [unwired: 1 out]
            n671 = local write "Index 2"(w1391) -> ()
            n672 = local write "XY Graph 2"(w1390) -> ()
            n673 = local write "MobVi Index"(w1393) -> ()
            n674 = local write "Slide"(w1393) -> ()
            n675 = local write "XY Graph"(w1394) -> ()
            n676 = local write "Calc: Mobility-Sat"(w1379) -> ()
            n677 = local write "Calc: VT-Sat"(w1372) -> ()
            n678 = local write "Calc: Mobility-Lin"(w1378) -> ()
            n679 = local write "Calc: Off I-Sat"(w1371) -> ()
            n680 = local write "Calc: On/Off"(w1364) -> ()
            n681 = Array Size(array=w1473) -> (size(s)=w1472:i32[])
            n682 = local write "Calc: VT-Lin"(w1377) -> ()
            n683 = call "Trap Density_VT.vi"("VT"=w1372, "Dielectric"=w1376) -> ("Trap Density-VT"=w1375:dbl)
            n684 = call "Trap Density_STS.vi"("Temp (T) [K]"=w1368, "S.T.S. (S)"=w1373, "Dielectric"=w1376) -> ("Trap Density (N)"=w1374:dbl)  [unwired: 8 in]
            n685 = local write "Calc: STS"(w1373) -> ()
            n686 = local write "New: STS"(w1373) -> ()
            n687 = Decimate 1D Array(w1365) -> (w1388:cluster{dbl[], dbl[]}[])  [unwired: 1 out]
            n688 = local write "Calc: Trap Density-VT"(w1375) -> ()
            n689 = local write "New: VT-Sat"(w1372) -> ()
            n690 = local write "Calc: Trap Density-STS"(w1374) -> ()
            n691 = local write "New: Trap Density-STS"(w1374) -> ()
            n692 = local write "New: Trap Density-VT"(w1375) -> ()
            n693 = local write "XY Graph-Lin"(w1365) -> ()
            n694 = local write "New: VT-Lin"(w1377) -> ()
            n695 = local write "New: Mobility-Sat"(w1379) -> ()
            n696 = local write "New: Mobility-Lin"(w1378) -> ()
            n697 = Decimate 1D Array(w1390) -> (w1450:cluster{dbl[], dbl[]}[])  [unwired: 1 out]
            n698 = Index Array(array=w1472, index=w1471) -> (element=w1456:i32)
            n699 = Decimate 1D Array(w1394) -> (w1460:cluster{dbl[], dbl[]}[])  [unwired: 1 out]
            n700 = Array To Cluster(array=w1388) -> (cluster=w1387:T9)
            n701 = Array Subset(array=w1473, index (row)=w1471, index (col)=w1471, length (col)=3) -> (w1474:string[][])  [unwired: 1 in]
            n702 = Array To Cluster(array=w1450) -> (cluster=w1448:T9)
            n703 = Array To Cluster(array=w1460) -> (cluster=w1462:T9)
            n704 = Reshape Array(w1474, w1456) -> (w1463:string[])
            n705 = Subtract(x=w1456, y=20) -> (x-y=w1455:i32)
            n706 = Unbundle(w1387) -> ("[0]"=w1384:cluster{dbl[], dbl[]})  [unwired: 8 out]
            n707 = property on="Slide" class="Slide (strict)"("Scale.Maximum"=w1455) -> ()  [unwired: 2 in, 2 out]
            n708 = Unbundle(w1448) -> ("[0]"=w1449:cluster{dbl[], dbl[]})  [unwired: 8 out]
            n709 = Unbundle(w1462) -> ("[0]"=w1461:cluster{dbl[], dbl[]})  [unwired: 8 out]
            n710 = local read "NumPts"() -> (w1381:dbl)
            n711 = Unbundle(w1384) -> (w1383:dbl[], w1382:dbl[])
            n712 = Search 1D Array(1D array=w1463, element="Index:") -> (index of element=w1468:i32)  [unwired: 1 in]
            n713 = Increment(x=w1468) -> (x+1=w1469:i32)
            n714 = Unbundle(w1449) -> (w1447:dbl[], w1446:dbl[])
            n715 = Unbundle(w1461) -> (w1454:dbl[], w1453:dbl[])
            n716 = Array Subset(array=w1383, index=w1380, length=w1381) -> (w1385:dbl[])
            n717 = Array Subset(array=w1382, index=w1380, length=w1381) -> (w1386:dbl[])
            n718 = local read "Image Folder"() -> (w1422:path)
            n719 = local write "Lin-Vg Array-Used"(w1385) -> ()
            n720 = Array Subset(array=w1447, index=w1391, length=w1392) -> (w1452:dbl[])
            n721 = Array Subset(array=w1446, index=w1391, length=w1392) -> (w1451:dbl[])
            n722 = Array Subset(array=w1454, index=w1393, length=w1396) -> (w1459:dbl[])
            n723 = Array Subset(array=w1453, index=w1393, length=w1396) -> (w1458:dbl[])
            n724 = local write "Lin Id-Used"(w1386) -> ()
            n725 = Index Array(array=w1463, index=w1469) -> (element=w1429:string)
            n726 = local write "Sat Vg Array-Used"(w1459) -> ()
            n727 = local write "Vg Array-Log-Used"(w1451) -> ()
            n728 = local write "Sat Id-Log-Used"(w1452) -> ()
            n729 = local write "Sat Id-Used"(w1458) -> ()
            n730 = local write "Index"(w1429) -> ()
            n731 = List Folder(path=w1422, error in=w1433) -> (filenames=w1465:string[], error out=w1432:errorcluster)  [unwired: 2 in, 2 out]
            n732 = Build Path(base path=w1422, name or relative path="ROI") -> (appended path=w1430:path)
            n733 = while {
              tunnel: w1465 -> [w1498]
              tunnel: w1429 -> [w1496]
              tunnel: [w1495] -> w1464
              tunnel: w1456 -> [w1494]
              i -> [w1495]
              stop <- w1491 stop-if-true
              n734 = Index Array(array=w1498, index=w1495) -> (element=w1499:string)
              n735 = xnode "Match Regular Expression"("input string"=w1499, "regular expression"=w1496) -> ("whole match"=w1497:string)  [unwired: 4 in, 4 out]
              n736 = Equal?(x=w1497, y=w1496) -> (x = y?=w1493:bool)
              n737 = Equal?(x=w1494, y=w1495) -> (x = y?=w1492:bool)
              n738 = Or(x=w1493, y=w1492) -> (x .or. y?=w1491:bool)
            }
            n739 = invoke on="Image Out" class="ImageControl" method="Clear ROI"(error in=w1432) -> (error out=w1436:errorcluster)  [unwired: 2 in, 2 out]
            n740 = Build Path(base path=w1430, name or relative path=w1429) -> (appended path=w1428:path)
            n741 = call <vilib>:"Check if File or Folder Exists.vi"("error in (no error)"=w1436, "path"=w1428) -> ("file or folder exists?"=w1434:bool, "dup path"=w1435:path)  [unwired: 7 in, 1 out]
            n742 = case shown="True" w1434 {
              tunnel: w1435 -> [_ w1486]
              frame False {
              }
              frame True {
                n743 = Read from Text File(file (use dialog)=w1486) -> (text=w1490:string)  [unwired: 3 in, 3 out]
                n744 = property on="Image Out" class="ImageControl"() -> ("ROI"=w1487:T10)  [unwired: 2 in, 2 out]
                n745 = Unflatten From String(type=w1487, binary string=w1490) -> (value=w1488:T10, error out=w1489:errorcluster)  [unwired: 3 in, 1 out]
                n746 = property on="Image Out" class="ImageControl"(error in=w1489, "ROI"=w1488) -> ()  [unwired: 1 in, 2 out]
              }
            }
            n747 = Index Array(array=w1465, index=w1464) -> (element=w1438:string)
            n748 = local write "Image Name"(w1438) -> ()
            n749 = Empty String/Path?(string/path=w1438) -> (empty?=w1445:bool)
            n750 = Build Path(base path=w1422, name or relative path=w1438) -> (appended path=w1437:path)
            n751 = local read "No Image"() -> (w1444:path)
            n752 = Select(t=w1444, s=w1445, f=w1437) -> (s? t:f=w1439:path)
            n753 = call <vilib>:"Get File Extension.vi"("file"=w1439) -> ("lowercase file extension"=w1441:string)  [unwired: 7 in, 3 out]
            n754 = local write "Image File"(w1439) -> ()
            n755 = local write "String"(w1441) -> ()
            n756 = Search 1D Array(1D array=string[] ["bmp", "jpeg", "png", "jpg", "gif"], element=w1441) -> (index of element=w1440:i32)  [unwired: 1 in]
            n757 = call "Vision Acquisition5"("Image Path"=w1439) -> ("Image Out"=w1443:T2)  [unwired: 25 in, 1 out]
            n758 = Less Than 0?(x=w1440) -> ()  [unwired: 1 out]
            n759 = local write "Image Out"(w1443) -> ()
            n760 = local write "Image Out 2"(w1443) -> ()
          }
          event "Save Changes? 3": Mouse Down {
            n761 = event-data() -> ()  [unwired: 1 in, 7 out]
            n762 = local read "Image Folder"() -> (w1615:path)
            n763 = Build Path(base path=w1615, name or relative path="ROI") -> (appended path=w1622:path)
            n764 = call <vilib>:"Check if File or Folder Exists.vi"("path"=w1622) -> ("file or folder exists?"=w1624:bool, "dup path"=w1621:path)  [unwired: 8 in, 1 out]
            n765 = case shown="False" w1624 {
              tunnel: w1621 -> [w1626 w1627]
              tunnel: [w1625 w1627] -> w1616
              frame False {
                n766 = Create Folder(path (use dialog)=w1626) -> (created path=w1625:path)  [unwired: 2 in, 2 out]
              }
              frame True {
              }
            }
            n767 = local read "Index"() -> (w1618:string)
            n768 = property on="Image Out" class="ImageControl"() -> ("ROI"=w1620:T10)  [unwired: 2 in, 2 out]
            n769 = Build Path(base path=w1616, name or relative path=w1618) -> (appended path=w1617:path)
            n770 = Flatten To String(anything=w1620) -> (data string=w1619:string)  [unwired: 3 in, 2 out]
            n771 = Write to Text File(file (use dialog)=w1617, text=w1619) -> ()  [unwired: 2 in, 3 out]
          }
          event "Next Button": Mouse Down {
            n772 = event-data() -> ()  [unwired: 1 in, 5 out]
            n773 = local read "XY Graph"() -> (w1640:cluster{dbl[], dbl[]}[])
            n774 = Decimate 1D Array(w1640) -> (w1636:cluster{dbl[], dbl[]}[], w1635:cluster{dbl[], dbl[]}[])
            n775 = Array To Cluster(array=w1636) -> (cluster=w1646:T9)
            n776 = local read "MobVi Index"() -> (w1642:dbl)
            n777 = Unbundle(w1646) -> ("[0]"=w1645:cluster{dbl[], dbl[]})  [unwired: 8 out]
            n778 = local read "NumPts"() -> (w1641:dbl)
            n779 = Unbundle(w1645) -> (w1644:dbl[], w1643:dbl[])
            n780 = Increment(x=w1642) -> (x+1=w1637:dbl)
            n781 = local read "New: Dielectric"() -> (w1631:dbl)
            n782 = local read "New: Length"() -> (w1630:dbl)
            n783 = local read "New: Width"() -> (w1629:dbl)
            n784 = local write "MobVi Index"(w1637) -> ()
            n785 = Array Subset(array=w1644, index=w1637, length=w1641) -> (w1633:dbl[])
            n786 = Array Subset(array=w1643, index=w1637, length=w1641) -> (w1632:dbl[])
            n787 = local write "Sat Vg Array-Used"(w1633) -> ()
            n788 = local write "Sat Id-Used"(w1632) -> ()
            n789 = call "Mobility-Vt-Used Pts_Saturation.vi"("Width"=w1629, "Length"=w1630, "Dielectric (d)"=w1631, "Sat Id Used"=w1632, "Vg Used"=w1633) -> ("Vt"=w1628:dbl, "Mobility"=w1634:dbl)  [unwired: 4 in, 1 out]
            n790 = Bundle(w1633, w1632) -> (w1639:cluster{dbl[], dbl[]})  [unwired: 1 in]
            n791 = Build Array (concatenate)(w1636, w1635, w1639) -> (w1638:cluster{dbl[], dbl[]}[])
            n792 = local write "New: Mobility-Sat"(w1634) -> ()
            n793 = local write "New: VT-Sat"(w1628) -> ()
            n794 = local write "XY Graph"(w1638) -> ()
          }
          event "Next Button 2": Mouse Down {
            n795 = event-data() -> ()  [unwired: 1 in, 7 out]
            n796 = local read "XY Graph 2"() -> (w1655:cluster{dbl[], dbl[]}[])
            n797 = Decimate 1D Array(w1655) -> (w1651:cluster{dbl[], dbl[]}[], w1650:cluster{dbl[], dbl[]}[])
            n798 = Array To Cluster(array=w1651) -> (cluster=w1661:T9)
            n799 = local read "Index 2"() -> (w1657:dbl)
            n800 = Unbundle(w1661) -> ("[0]"=w1660:cluster{dbl[], dbl[]})  [unwired: 8 out]
            n801 = local read "NumPts 2"() -> (w1656:dbl)
            n802 = Unbundle(w1660) -> (w1659:dbl[], w1658:dbl[])
            n803 = Increment(x=w1657) -> (x+1=w1652:dbl)
            n804 = local write "Index 2"(w1652) -> ()
            n805 = Array Subset(array=w1658, index=w1652, length=w1656) -> (w1647:dbl[])
            n806 = Array Subset(array=w1659, index=w1652, length=w1656) -> (w1648:dbl[])
            n807 = call "STS-Used.vi"("Id Used"=w1648, "Vg-Used"=w1647) -> ("STS"=w1649:dbl)  [unwired: 9 in]
            n808 = Bundle(w1648, w1647) -> (w1654:cluster{dbl[], dbl[]})  [unwired: 1 in]
            n809 = local write "Vg Array-Log-Used"(w1647) -> ()
            n810 = local write "Sat Id-Log-Used"(w1648) -> ()
            n811 = local write "New: STS"(w1649) -> ()
            n812 = Build Array (concatenate)(w1651, w1650, w1654) -> (w1653:cluster{dbl[], dbl[]}[])
            n813 = local write "XY Graph 2"(w1653) -> ()
          }
          event "Previous Button 2": Mouse Down {
            n814 = event-data() -> ()  [unwired: 1 in, 7 out]
            n815 = local read "XY Graph 2"() -> (w1671:cluster{dbl[], dbl[]}[])
            n816 = Decimate 1D Array(w1671) -> (w1668:cluster{dbl[], dbl[]}[], w1667:cluster{dbl[], dbl[]}[])
            n817 = Array To Cluster(array=w1668) -> (cluster=w1676:T9)
            n818 = local read "Index 2"() -> (w1664:dbl)
            n819 = Unbundle(w1676) -> ("[0]"=w1675:cluster{dbl[], dbl[]})  [unwired: 8 out]
            n820 = local read "NumPts 2"() -> (w1672:dbl)
            n821 = Unbundle(w1675) -> (w1674:dbl[], w1673:dbl[])
            n822 = Decrement(x=w1664) -> (x-1=w1665:dbl)
            n823 = local write "Index 2"(w1665) -> ()
            n824 = Array Subset(array=w1674, index=w1665, length=w1672) -> (w1662:dbl[])
            n825 = Array Subset(array=w1673, index=w1665, length=w1672) -> (w1663:dbl[])
            n826 = local write "Vg Array-Log-Used"(w1663) -> ()
            n827 = local write "Sat Id-Log-Used"(w1662) -> ()
            n828 = Bundle(w1662, w1663) -> (w1670:cluster{dbl[], dbl[]})  [unwired: 1 in]
            n829 = call "STS-Used.vi"("Id Used"=w1662, "Vg-Used"=w1663) -> ("STS"=w1666:dbl)  [unwired: 9 in]
            n830 = Build Array (concatenate)(w1668, w1667, w1670) -> (w1669:cluster{dbl[], dbl[]}[])
            n831 = local write "New: STS"(w1666) -> ()
            n832 = local write "XY Graph 2"(w1669) -> ()
          }
          event "Previous Button": Mouse Down {
            n833 = event-data() -> ()  [unwired: 1 in, 5 out]
            n834 = local read "XY Graph"() -> (w1690:cluster{dbl[], dbl[]}[])
            n835 = Decimate 1D Array(w1690) -> (w1687:cluster{dbl[], dbl[]}[], w1686:cluster{dbl[], dbl[]}[])
            n836 = Array To Cluster(array=w1687) -> (cluster=w1695:T9)
            n837 = local read "MobVi Index"() -> (w1685:dbl)
            n838 = Unbundle(w1695) -> ("[0]"=w1694:cluster{dbl[], dbl[]})  [unwired: 8 out]
            n839 = local read "NumPts"() -> (w1691:dbl)
            n840 = Unbundle(w1694) -> (w1693:dbl[], w1692:dbl[])
            n841 = Decrement(x=w1685) -> (x-1=w1684:dbl)
            n842 = local read "New: Dielectric"() -> (w1678:dbl)
            n843 = local read "New: Length"() -> (w1679:dbl)
            n844 = local read "New: Width"() -> (w1680:dbl)
            n845 = local write "MobVi Index"(w1684) -> ()
            n846 = Array Subset(array=w1693, index=w1684, length=w1691) -> (w1683:dbl[])
            n847 = Array Subset(array=w1692, index=w1684, length=w1691) -> (w1682:dbl[])
            n848 = local write "Sat Vg Array-Used"(w1683) -> ()
            n849 = local write "Sat Id-Used"(w1682) -> ()
            n850 = call "Mobility-Vt-Used Pts_Linear.vi"("Width"=w1680, "Length"=w1679, "Dielectric (d)"=w1678, "Sat Id Used"=w1682, "Vg Used"=w1683) -> ("Vt"=w1677:dbl, "Mobility"=w1681:dbl)  [unwired: 4 in, 1 out]
            n851 = Bundle(w1683, w1682) -> (w1689:cluster{dbl[], dbl[]})  [unwired: 1 in]
            n852 = local write "New: VT-Sat"(w1677) -> ()
            n853 = Build Array (concatenate)(w1687, w1686, w1689) -> (w1688:cluster{dbl[], dbl[]}[])
            n854 = local write "New: Mobility-Sat"(w1681) -> ()
            n855 = local write "XY Graph"(w1688) -> ()
          }
          event "Slide": Value Change {
            n856 = event-data() -> ()  [unwired: 1 in, 5 out]
            n857 = local read "XY Graph"() -> (w1708:cluster{dbl[], dbl[]}[])
            n858 = Decimate 1D Array(w1708) -> (w1705:cluster{dbl[], dbl[]}[], w1704:cluster{dbl[], dbl[]}[])
            n859 = Array To Cluster(array=w1705) -> (cluster=w1713:T9)
            n860 = Unbundle(w1713) -> ("[0]"=w1712:cluster{dbl[], dbl[]})  [unwired: 8 out]
            n861 = local read "NumPts"() -> (w1709:dbl)
            n862 = local read "Slide"() -> (w1697:dbl)
            n863 = Unbundle(w1712) -> (w1711:dbl[], w1710:dbl[])
            n864 = local read "New: Dielectric"() -> (w1698:dbl)
            n865 = local read "New: Length"() -> (w1699:dbl)
            n866 = local read "New: Width"() -> (w1700:dbl)
            n867 = local write "MobVi Index"(w1697) -> ()
            n868 = Array Subset(array=w1711, index=w1697, length=w1709) -> (w1703:dbl[])
            n869 = Array Subset(array=w1710, index=w1697, length=w1709) -> (w1702:dbl[])
            n870 = local write "Sat Vg Array-Used"(w1703) -> ()
            n871 = local write "Sat Id-Used"(w1702) -> ()
            n872 = call "Mobility-Vt-Used Pts_Linear.vi"("Width"=w1700, "Length"=w1699, "Dielectric (d)"=w1698, "Sat Id Used"=w1702, "Vg Used"=w1703) -> ("Vt"=w1696:dbl, "Mobility"=w1701:dbl)  [unwired: 4 in, 1 out]
            n873 = Bundle(w1703, w1702) -> (w1707:cluster{dbl[], dbl[]})  [unwired: 1 in]
            n874 = local write "New: VT-Sat"(w1696) -> ()
            n875 = Build Array (concatenate)(w1705, w1704, w1707) -> (w1706:cluster{dbl[], dbl[]}[])
            n876 = local write "New: Mobility-Sat"(w1701) -> ()
            n877 = local write "XY Graph"(w1706) -> ()
          }
          event "Slide 2": Value Change {
            n878 = event-data() -> ()  [unwired: 1 in, 5 out]
            n879 = local read "XY Graph 2"() -> (w1722:cluster{dbl[], dbl[]}[])
            n880 = Decimate 1D Array(w1722) -> (w1719:cluster{dbl[], dbl[]}[], w1718:cluster{dbl[], dbl[]}[])
            n881 = Array To Cluster(array=w1719) -> (cluster=w1727:T9)
            n882 = Unbundle(w1727) -> ("[0]"=w1726:cluster{dbl[], dbl[]})  [unwired: 8 out]
            n883 = local read "NumPts 2"() -> (w1723:dbl)
            n884 = local read "Slide 2"() -> (w1717:dbl)
            n885 = Unbundle(w1726) -> (w1725:dbl[], w1724:dbl[])
            n886 = local write "Index 2"(w1717) -> ()
            n887 = Array Subset(array=w1725, index=w1717, length=w1723) -> (w1715:dbl[])
            n888 = Array Subset(array=w1724, index=w1717, length=w1723) -> (w1714:dbl[])
            n889 = local write "Vg Array-Log-Used"(w1714) -> ()
            n890 = local write "Sat Id-Log-Used"(w1715) -> ()
            n891 = call "STS-Used.vi"("Id Used"=w1715, "Vg-Used"=w1714) -> ("STS"=w1716:dbl)  [unwired: 9 in]
            n892 = Bundle(w1715, w1714) -> (w1721:cluster{dbl[], dbl[]})  [unwired: 1 in]
            n893 = local write "New: STS"(w1716) -> ()
            n894 = Build Array (concatenate)(w1719, w1718, w1721) -> (w1720:cluster{dbl[], dbl[]}[])
            n895 = local write "XY Graph 2"(w1720) -> ()
          }
          event "Save Changes?": Mouse Down {
            n896 = event-data() -> ()  [unwired: 1 in, 5 out]
            n897 = flat-sequence {
              tunnel: [w1755] -> w1732
              tunnel: [w1749] -> w1731
              tunnel: [w1735] -> w1730
              tunnel: w1732 -> [w2036]
              tunnel: w1731 -> [w2033]
              tunnel: [w2034] -> w1729
              tunnel: w1730 -> [w2034]
              tunnel: [w2033] -> w1728
              tunnel: w1729 -> [w2041]
              tunnel: w1728 -> [w2040]
              frame #0 {
                n898 = local read "New: Temp"() -> (w1736:dbl)
                n899 = local read "Data File"() -> (w1755:path)
                n900 = local read "New: Length"() -> (w1740:dbl)
                n901 = local read "New: Width"() -> (w1738:dbl)
                n902 = To Single Precision Float(number=w1736) -> (single precision float=w1737:sgl)
                n903 = call-poly <vilib>:"Read From Spreadsheet File.vi"("file path (dialog if empty)"=w1755) -> ("all rows"=w1733:string[][])  [unwired: 6 in, 4 out]
                n904 = Number To Decimal String(number=w1737) -> (decimal integer string=w1752:string)  [unwired: 1 in]
                n905 = To Single Precision Float(number=w1738) -> (single precision float=w1739:sgl)
                n906 = To Single Precision Float(number=w1740) -> (single precision float=w1741:sgl)
                n907 = local read "Index"() -> (w1758:string)
                n908 = Strip Path(path=w1755) -> (stripped path=w1763:path)  [unwired: 1 out]
                n909 = Number To Decimal String(number=w1741) -> (decimal integer string=w1756:string)  [unwired: 1 in]
                n910 = Number To Decimal String(number=w1739) -> (decimal integer string=w1757:string)  [unwired: 1 in]
                n911 = Array Size(array=w1733) -> (size(s)=w1746:i32[])
                n912 = Concatenate Strings("_", w1752, "K") -> (w1750:string)
                n913 = Array Subset(array=w1733, index (row)=0, index (col)=0, length (col)=3) -> (w1742:string[][])  [unwired: 1 in]
                n914 = Index Array(array=w1746, index=0) -> (element=w1748:i32)
                n915 = call "Build Text"("Temp"=w1750, "Index"=w1758, "Length"=w1756, "Width"=w1757) -> ("Result"=w1759:string)  [unwired: 10 in, 1 out]
                n916 = flat-sequence {
                  tunnel: [w1990] -> w1754
                  tunnel: w1754 -> [w2007]
                  frame #0 {
                    # "Makes Empty File for Transformer Data"
                    n917 = local read "Data Folder"() -> (w1979:path)
                    n918 = Build Path(base path=w1979, name or relative path="Stats") -> (appended path=w1981:path)
                    n919 = call <vilib>:"Check if File or Folder Exists.vi"("path"=w1981) -> ("file or folder exists?"=w1982:bool, "dup path"=w1983:path)  [unwired: 8 in, 1 out]
                    n920 = case shown="False" w1982 {
                      tunnel: [w1987 w1989] -> w1984
                      tunnel: w1983 -> [w1988 w1989]
                      frame False {
                        n921 = Create Folder(path (use dialog)=w1988) -> (created path=w1987:path)  [unwired: 2 in, 2 out]
                      }
                      frame True {
                      }
                    }
                    n922 = Build Path(base path=w1984, name or relative path="Tranformer Data.txt") -> (appended path=w1986:path)
                    n923 = call-poly <vilib>:"Write To Spreadsheet File.vi"("append to file? (new file:F)"=TRUE, "file path (dialog if empty)"=w1986) -> ()  [unwired: 6 in, 1 out]
                  }
                  frame #1 {
                    # "Adds Headers if they don't exist"
                    n924 = Concatenate Strings("Stats\\", "Tranformer Data.txt") -> (w1997:string)
                    n925 = local read "Data Folder"() -> (w1996:path)
                    n926 = Build Path(base path=w1996, name or relative path=w1997) -> (appended path=w1990:path)
                    n927 = call-poly <vilib>:"Read From Spreadsheet File.vi"("file path (dialog if empty)"=w1990) -> ("first row"=w1995:string[])  [unwired: 6 in, 4 out]
                    n928 = Search 1D Array(1D array=w1995, element="DeviceID") -> (index of element=w1993:i32)  [unwired: 1 in]
                    n929 = Equal?(x=w1993, y=0) -> (x = y?=w1991:bool)
                    n930 = case shown="False" w1991 {
                      tunnel: w1990 -> [w2001 _]
                      frame False {
                        n931 = local read "Transformer \nHeaders"() -> (w2000:string[])
                        n932 = call-poly <vilib>:"Write To Spreadsheet File.vi"("1D data"=w2000, "file path (dialog if empty)"=w2001) -> ()  [unwired: 6 in, 1 out]
                      }
                      frame True {
                      }
                    }
                  }
                  frame #2 {
                    # "Adds current device if it doesn't exist"
                    n933 = local read "Current \nRecord"() -> (w2006:string[])
                    n934 = Index Array(array=w2006, index=0) -> (element=w2005:string)
                    n935 = Concatenate Strings("Stats\\", "Tranformer Data.txt") -> (w2010:string)
                    n936 = local read "Data Folder"() -> (w2009:path)
                    n937 = local write "Current Device ID"(w2005) -> ()
                    n938 = local read "Current Device ID"() -> (w2015:string)
                    n939 = Build Path(base path=w2009, name or relative path=w2010) -> (appended path=w2008:path)
                    n940 = call-poly <vilib>:"Read From Spreadsheet File.vi"("file path (dialog if empty)"=w2008) -> ("all rows"=w2002:string[][])  [unwired: 6 in, 4 out]
                    n941 = Index Array(array=w2002, index (col)=0) -> (element=w2003:string[])  [unwired: 1 in]
                    n942 = Search 1D Array(1D array=w2003, element=w2015) -> (index of element=w2004:i32)  [unwired: 1 in]
                    n943 = Equal?(x=w2004, y=-1) -> (x = y?=w2017:bool)
                    n944 = case shown="False" w2017 {
                      tunnel: w2007 -> [w2020 w2031]
                      tunnel: w2004 -> [w2023 _]
                      tunnel: w2002 -> [w2024 _]
                      frame False {
                        n945 = local read "Current \nRecord"() -> (w2022:string[])
                        n946 = Replace Array Subset(array=w2024, new element=w2022, index (row)=w2023) -> (w2021:string[][])  [unwired: 1 in]
                        n947 = flat-sequence {
                          tunnel: w2020 -> [w2025]
                          tunnel: w2021 -> [w2026]
                          tunnel: [w2026] -> w2019
                          tunnel: [w2025] -> w2018
                          tunnel: w2019 -> [w2028]
                          tunnel: w2018 -> [w2027]
                          frame #0 {
                            n948 = Delete(path (use dialog)=w2025) -> ()  [unwired: 4 in, 3 out]
                          }
                          frame #1 {
                            n949 = call-poly <vilib>:"Write To Spreadsheet File.vi"("append to file? (new file:F)"=TRUE, "2D data"=w2028, "file path (dialog if empty)"=w2027) -> ()  [unwired: 5 in, 1 out]
                          }
                        }
                      }
                      frame True {
                        n950 = local read "Current \nRecord"() -> (w2030:string[])
                        n951 = call-poly <vilib>:"Write To Spreadsheet File.vi"("append to file? (new file:F)"=TRUE, "1D data"=w2030, "file path (dialog if empty)"=w2031) -> ()  [unwired: 5 in, 1 out]
                      }
                    }
                  }
                }
                n952 = Reshape Array(w1742, w1748) -> (w1734:string[])
                n953 = Path To String(path=w1763) -> (string=w1761:string)
                n954 = stacked-sequence {
                  tunnel: w1734 -> [w1770 w1783 w1801 w1819 w1837 w1855 w1873 w1891 w1908 w1926 w1944 w1962]
                  tunnel: [_ _ _ _ _ _ _ _ _ _ _ w1960] -> w1735
                  frame #0 {
                    n955 = Search 1D Array(1D array=w1770, element="Dielectric (nm):") -> (index of element=w1767:i32)  [unwired: 1 in]
                    n956 = Equal?(x=w1767, y=-1) -> (x = y?=w1766:bool)
                    n957 = local read "Save1 Array"() -> (w1765:string[][])
                    n958 = case shown="False" w1766 {
                      tunnel: w1765 -> [w1776 w1780]
                      tunnel: w1767 -> [w1772 _]
                      tunnel: [w1771 w1780] -> w1764
                      frame False {
                        n959 = local read "New: Dielectric"() -> (w1778:dbl)
                        n960 = Number To Fractional String(number=w1778) -> (F-format string=w1773:string)  [unwired: 3 in]
                        n961 = Divide(x=w1772, y=3) -> (x/y=w1775:dbl)
                        n962 = To Word Integer(number=w1775) -> (16bit integer=w1774:i16)
                        n963 = Replace Array Subset(array=w1776, new element=w1773, index (row)=w1774, index (col)=1) -> (w1771:string[][])
                      }
                      frame True {
                      }
                    }
                    n964 = local write "Save1 Array"(w1764) -> ()
                  }
                  frame #1 {
                    n965 = Search 1D Array(1D array=w1783, element="Length (um):") -> (index of element=w1785:i32)  [unwired: 1 in]
                    n966 = Equal?(x=w1785, y=-1) -> (x = y?=w1784:bool)
                    n967 = local read "Save1 Array"() -> (w1782:string[][])
                    n968 = case shown="False" w1784 {
                      tunnel: w1782 -> [w1795 w1798]
                      tunnel: w1785 -> [w1792 _]
                      tunnel: [w1791 w1798] -> w1781
                      frame False {
                        n969 = local read "New: Length"() -> (w1788:dbl)
                        n970 = Divide(x=w1792, y=3) -> (x/y=w1794:dbl)
                        n971 = Format Value(format string="%#g", value (0)=w1788) -> (output string=w1789:string)  [unwired: 1 in]
                        n972 = To Word Integer(number=w1794) -> (16bit integer=w1793:i16)
                        n973 = Replace Array Subset(array=w1795, new element=w1789, index (row)=w1793, index (col)=1) -> (w1791:string[][])
                      }
                      frame True {
                      }
                    }
                    n974 = local write "Save1 Array"(w1781) -> ()
                  }
                  frame #2 {
                    n975 = Search 1D Array(1D array=w1801, element="Width (um):") -> (index of element=w1803:i32)  [unwired: 1 in]
                    n976 = Equal?(x=w1803, y=-1) -> (x = y?=w1802:bool)
                    n977 = local read "Save1 Array"() -> (w1800:string[][])
                    n978 = case shown="False" w1802 {
                      tunnel: w1803 -> [w1811 _]
                      tunnel: w1800 -> [w1810 w1816]
                      tunnel: [w1809 w1816] -> w1799
                      frame False {
                        n979 = local read "New: Width"() -> (w1806:dbl)
                        n980 = Divide(x=w1811, y=3) -> (x/y=w1813:dbl)
                        n981 = To Word Integer(number=w1813) -> (16bit integer=w1812:i16)
                        n982 = Format Value(format string="%#g", value (0)=w1806) -> (output string=w1807:string)  [unwired: 1 in]
                        n983 = Replace Array Subset(array=w1810, new element=w1807, index (row)=w1812, index (col)=1) -> (w1809:string[][])
                      }
                      frame True {
                      }
                    }
                    n984 = local write "Save1 Array"(w1799) -> ()
                  }
                  frame #3 {
                    n985 = Search 1D Array(1D array=w1819, element="Sample Temp (K):") -> (index of element=w1821:i32)  [unwired: 1 in]
                    n986 = Equal?(x=w1821, y=-1) -> (x = y?=w1820:bool)
                    n987 = local read "Save1 Array"() -> (w1818:string[][])
                    n988 = case shown="False" w1820 {
                      tunnel: w1818 -> [w1831 w1834]
                      tunnel: w1821 -> [w1828 _]
                      tunnel: [w1827 w1834] -> w1817
                      frame False {
                        n989 = local read "New: Temp"() -> (w1825:dbl)
                        n990 = Divide(x=w1828, y=3) -> (x/y=w1830:dbl)
                        n991 = Format Value(format string="%#g", value (0)=w1825) -> (output string=w1824:string)  [unwired: 1 in]
                        n992 = To Word Integer(number=w1830) -> (16bit integer=w1829:i16)
                        n993 = Replace Array Subset(array=w1831, new element=w1824, index (row)=w1829, index (col)=1) -> (w1827:string[][])
                      }
                      frame True {
                      }
                    }
                    n994 = local write "Save1 Array"(w1817) -> ()
                  }
                  frame #4 {
                    n995 = Search 1D Array(1D array=w1837, element="Mobility-Sat (cm^2/Vs):") -> (index of element=w1839:i32)  [unwired: 1 in]
                    n996 = Equal?(x=w1839, y=-1) -> (x = y?=w1838:bool)
                    n997 = local read "Save1 Array"() -> (w1835:string[][])
                    n998 = case shown="False" w1838 {
                      tunnel: w1835 -> [w1849 w1852]
                      tunnel: w1839 -> [w1846 _]
                      tunnel: [w1845 w1852] -> w1836
                      frame False {
                        n999 = local read "New: Mobility-Sat"() -> (w1842:dbl)
                        n1000 = Divide(x=w1846, y=3) -> (x/y=w1848:dbl)
                        n1001 = To Word Integer(number=w1848) -> (16bit integer=w1847:i16)
                        n1002 = Format Value(format string="%#g", value (0)=w1842) -> (output string=w1843:string)  [unwired: 1 in]
                        n1003 = Replace Array Subset(array=w1849, new element=w1843, index (row)=w1847, index (col)=1) -> (w1845:string[][])
                      }
                      frame True {
                      }
                    }
                    n1004 = local write "Save1 Array"(w1836) -> ()
                  }
                  frame #5 {
                    n1005 = Search 1D Array(1D array=w1855, element="Mobility-Lin (cm^2/Vs):") -> (index of element=w1857:i32)  [unwired: 1 in]
                    n1006 = Equal?(x=w1857, y=-1) -> (x = y?=w1856:bool)
                    n1007 = local read "Save1 Array"() -> (w1854:string[][])
                    n1008 = case shown="False" w1856 {
                      tunnel: w1854 -> [w1867 w1870]
                      tunnel: w1857 -> [w1864 _]
                      tunnel: [w1863 w1870] -> w1853
                      frame False {
                        n1009 = local read "Calc: Mobility-Lin"() -> (w1860:dbl)
                        n1010 = Divide(x=w1864, y=3) -> (x/y=w1866:dbl)
                        n1011 = To Word Integer(number=w1866) -> (16bit integer=w1865:i16)
                        n1012 = Format Value(format string="%#g", value (0)=w1860) -> (output string=w1861:string)  [unwired: 1 in]
                        n1013 = Replace Array Subset(array=w1867, new element=w1861, index (row)=w1865, index (col)=1) -> (w1863:string[][])
                      }
                      frame True {
                      }
                    }
                    n1014 = local write "Save1 Array"(w1853) -> ()
                  }
                  frame #6 {
                    n1015 = Search 1D Array(1D array=w1873, element="Off I-Sat (A):") -> (index of element=w1875:i32)  [unwired: 1 in]
                    n1016 = Equal?(x=w1875, y=-1) -> (x = y?=w1874:bool)
                    n1017 = local read "Save1 Array"() -> (w1872:string[][])
                    n1018 = case shown="False" w1874 {
                      tunnel: w1872 -> [w1885 w1888]
                      tunnel: w1875 -> [w1882 _]
                      tunnel: [w1881 w1888] -> w1871
                      frame False {
                        n1019 = local read "Calc: Off I-Sat"() -> (w1880:dbl)
                        n1020 = Divide(x=w1882, y=3) -> (x/y=w1884:dbl)
                        n1021 = Format Value(format string="%#g", value (0)=w1880) -> (output string=w1878:string)  [unwired: 1 in]
                        n1022 = To Word Integer(number=w1884) -> (16bit integer=w1883:i16)
                        n1023 = Replace Array Subset(array=w1885, new element=w1878, index (row)=w1883, index (col)=1) -> (w1881:string[][])
                      }
                      frame True {
                      }
                    }
                    n1024 = local write "Save1 Array"(w1871) -> ()
                  }
                  frame #7 {
                    n1025 = Search 1D Array(1D array=w1891, element="Vt-Sat (V):") -> (index of element=w1893:i32)  [unwired: 1 in]
                    n1026 = Equal?(x=w1893, y=-1) -> (x = y?=w1892:bool)
                    n1027 = local read "Save1 Array"() -> (w1890:string[][])
                    n1028 = case shown="False" w1892 {
                      tunnel: w1890 -> [w1901 w1905]
                      tunnel: w1893 -> [w1897 _]
                      tunnel: [w1896 w1905] -> w1889
                      frame False {
                        n1029 = local read "New: VT-Sat"() -> (w1903:dbl)
                        n1030 = Number To Fractional String(number=w1903) -> (F-format string=w1898:string)  [unwired: 3 in]
                        n1031 = Divide(x=w1897, y=3) -> (x/y=w1900:dbl)
                        n1032 = To Word Integer(number=w1900) -> (16bit integer=w1899:i16)
                        n1033 = Replace Array Subset(array=w1901, new element=w1898, index (row)=w1899, index (col)=1) -> (w1896:string[][])
                      }
                      frame True {
                      }
                    }
                    n1034 = local write "Save1 Array"(w1889) -> ()
                  }
                  frame #8 {
                    n1035 = Search 1D Array(1D array=w1908, element="VT-Lin (V):") -> (index of element=w1910:i32)  [unwired: 1 in]
                    n1036 = Equal?(x=w1910, y=-1) -> (x = y?=w1909:bool)
                    n1037 = local read "Save1 Array"() -> (w1907:string[][])
                    n1038 = case shown="False" w1909 {
                      tunnel: w1907 -> [w1920 w1923]
                      tunnel: w1910 -> [w1917 _]
                      tunnel: [w1916 w1923] -> w1906
                      frame False {
                        n1039 = local read "New: VT-Lin"() -> (w1914:dbl)
                        n1040 = Divide(x=w1917, y=3) -> (x/y=w1919:dbl)
                        n1041 = Format Value(format string="%#g", value (0)=w1914) -> (output string=w1913:string)  [unwired: 1 in]
                        n1042 = To Word Integer(number=w1919) -> (16bit integer=w1918:i16)
                        n1043 = Replace Array Subset(array=w1920, new element=w1913, index (row)=w1918, index (col)=1) -> (w1916:string[][])
                      }
                      frame True {
                      }
                    }
                    n1044 = local write "Save1 Array"(w1906) -> ()
                  }
                  frame #9 {
                    n1045 = Search 1D Array(1D array=w1926, element="STS-Sat (V/decade):") -> (index of element=w1928:i32)  [unwired: 1 in]
                    n1046 = Equal?(x=w1928, y=-1) -> (x = y?=w1927:bool)
                    n1047 = local read "Save1 Array"() -> (w1925:string[][])
                    n1048 = case shown="False" w1927 {
                      tunnel: w1925 -> [w1938 w1941]
                      tunnel: w1928 -> [w1935 _]
                      tunnel: [w1934 w1941] -> w1924
                      frame False {
                        n1049 = local read "New: STS"() -> (w1932:dbl)
                        n1050 = Divide(x=w1935, y=3) -> (x/y=w1937:dbl)
                        n1051 = Format Value(format string="%#g", value (0)=w1932) -> (output string=w1931:string)  [unwired: 1 in]
                        n1052 = To Word Integer(number=w1937) -> (16bit integer=w1936:i16)
                        n1053 = Replace Array Subset(array=w1938, new element=w1931, index (row)=w1936, index (col)=1) -> (w1934:string[][])
                      }
                      frame True {
                      }
                    }
                    n1054 = local write "Save1 Array"(w1924) -> ()
                  }
                  frame #10 {
                    n1055 = Search 1D Array(1D array=w1944, element="Trap Density-VT (Traps/Vcm^2):") -> (index of element=w1946:i32)  [unwired: 1 in]
                    n1056 = Equal?(x=w1946, y=-1) -> (x = y?=w1945:bool)
                    n1057 = local read "Save1 Array"() -> (w1943:string[][])
                    n1058 = case shown="False" w1945 {
                      tunnel: w1943 -> [w1956 w1959]
                      tunnel: w1946 -> [w1952 _]
                      tunnel: [w1951 w1959] -> w1942
                      frame False {
                        n1059 = local read "New: Trap Density-VT"() -> (w1950:dbl)
                        n1060 = Format Value(format string="%#g", value (0)=w1950) -> (output string=w1953:string)  [unwired: 1 in]
                        n1061 = Divide(x=w1952, y=3) -> (x/y=w1955:dbl)
                        n1062 = To Word Integer(number=w1955) -> (16bit integer=w1954:i16)
                        n1063 = Replace Array Subset(array=w1956, new element=w1953, index (row)=w1954, index (col)=1) -> (w1951:string[][])
                      }
                      frame True {
                      }
                    }
                    n1064 = local write "Save1 Array"(w1942) -> ()
                  }
                  frame #11 {
                    n1065 = Search 1D Array(1D array=w1962, element="Trap Density-STS (Traps/Vcm^2):") -> (index of element=w1964:i32)  [unwired: 1 in]
                    n1066 = Equal?(x=w1964, y=-1) -> (x = y?=w1963:bool)
                    n1067 = local read "Save1 Array"() -> (w1961:string[][])
                    n1068 = case shown="False" w1963 {
                      tunnel: w1961 -> [w1974 w1977]
                      tunnel: w1964 -> [w1971 _]
                      tunnel: [w1970 w1977] -> w1960
                      frame False {
                        n1069 = local read "New: Trap Density-STS"() -> (w1968:dbl)
                        n1070 = Divide(x=w1971, y=3) -> (x/y=w1973:dbl)
                        n1071 = To Word Integer(number=w1973) -> (16bit integer=w1972:i16)
                        n1072 = Format Value(format string="%#g", value (0)=w1968) -> (output string=w1967:string)  [unwired: 1 in]
                        n1073 = Replace Array Subset(array=w1974, new element=w1967, index (row)=w1972, index (col)=1) -> (w1970:string[][])
                      }
                      frame True {
                      }
                    }
                    n1074 = local write "Save1 Array"(w1960) -> ()
                  }
                }
                n1075 = Concatenate Strings(w1761, "\\", w1759) -> (w1760:string)
                n1076 = String To Path(string=w1760) -> (path=w1749:path)
                n1077 = local write "Save1 Array"(w1733) -> ()
              }
              frame #1 {
                n1078 = Equal?(x=w2036, y=w2033) -> (x = y?=w2035:bool)
                n1079 = case shown="False" w2035 {
                  tunnel: w2036 -> [w2039 _]
                  tunnel: w2033 -> [w2038 _]
                  frame False {
                    n1080 = Move(source path=w2039, 9:TRUE, 10:w2038) -> ()  [unwired: 2 in, 3 out]
                  }
                  frame True {
                  }
                }
              }
              frame #2 {
                n1081 = local write "Data File"(w2040) -> ()
                n1082 = call-poly <vilib>:"Write To Spreadsheet File.vi"("2D data"=w2041, "file path (dialog if empty)"=w2040) -> ()  [unwired: 6 in, 1 out]
              }
            }
          }
          event "Save Changes? 2": Mouse Down {
            n1083 = event-data() -> ()  [unwired: 1 in, 5 out]
            n1084 = stacked-sequence {
              seq-local: [w2101 _ _ _ _] -> [_ w2336 _ _ _]
              seq-local: [w2104 _ _ _ _] -> [_ w2337 _ _ _]
              seq-local: [w2101 _ _ _ _] -> [_ w2335 _ _ _]
              seq-local: [w2099 _ _ _ _] -> [_ w2333 _ _ _]
              seq-local: [_ w2337 _ _ _] -> [_ _ w2342 _ _]
              seq-local: [_ w2333 _ _ _] -> [_ _ w2341 _ _]
              frame #0 {
                n1085 = local read "New: Temp"() -> (w2103:dbl)
                n1086 = local read "Data File"() -> (w2104:path)
                n1087 = local read "New: Length"() -> (w2107:dbl)
                n1088 = local read "New: Width"() -> (w2105:dbl)
                n1089 = To Word Integer(number=w2103) -> (16bit integer=w2102:i16)
                n1090 = call-poly <vilib>:"Read From Spreadsheet File.vi"("file path (dialog if empty)"=w2104) -> ("all rows"=w2098:string[][])  [unwired: 6 in, 4 out]
                n1091 = Number To Decimal String(number=w2102) -> (decimal integer string=w2118:string)  [unwired: 1 in]
                n1092 = To Single Precision Float(number=w2105) -> (single precision float=w2106:sgl)
                n1093 = To Single Precision Float(number=w2107) -> (single precision float=w2108:sgl)
                n1094 = local read "Index"() -> (w2122:string)
                n1095 = Strip Path(path=w2104) -> (stripped path=w2127:path)  [unwired: 1 out]
                n1096 = Number To Decimal String(number=w2108) -> (decimal integer string=w2120:string)  [unwired: 1 in]
                n1097 = Number To Decimal String(number=w2106) -> (decimal integer string=w2121:string)  [unwired: 1 in]
                n1098 = Array Size(array=w2098) -> (size(s)=w2113:i32[])
                n1099 = Concatenate Strings("_", w2118, "K") -> (w2116:string)
                n1100 = Array Subset(array=w2098, index (row)=0, index (col)=0, length (col)=3) -> (w2109:string[][])  [unwired: 1 in]
                n1101 = Index Array(array=w2113, index=0) -> (element=w2115:i32)
                n1102 = call "Build Text2"("Temp"=w2116, "Index"=w2122, "Length"=w2120, "Width"=w2121) -> ("Result"=w2123:string)  [unwired: 10 in, 1 out]
                n1103 = Reshape Array(w2109, w2115) -> (w2100:string[])
                n1104 = Path To String(path=w2127) -> (string=w2125:string)
                n1105 = stacked-sequence {
                  tunnel: w2100 -> [w2134 w2147 w2164 w2181 w2198 w2215 w2232 w2250 w2267 w2284 w2301 w2318]
                  tunnel: [_ _ _ _ _ _ _ _ _ _ _ w2316] -> w2099
                  frame #0 {
                    n1106 = Search 1D Array(1D array=w2134, element="Dielectric (nm):") -> (index of element=w2131:i32)  [unwired: 1 in]
                    n1107 = Equal?(x=w2131, y=-1) -> (x = y?=w2130:bool)
                    n1108 = local read "Save1 Array"() -> (w2129:string[][])
                    n1109 = case shown="False" w2130 {
                      tunnel: w2129 -> [w2140 w2144]
                      tunnel: w2131 -> [w2136 _]
                      tunnel: [w2135 w2144] -> w2128
                      frame False {
                        n1110 = local read "New: Dielectric"() -> (w2142:dbl)
                        n1111 = Number To Fractional String(number=w2142) -> (F-format string=w2137:string)  [unwired: 3 in]
                        n1112 = Divide(x=w2136, y=3) -> (x/y=w2139:dbl)
                        n1113 = To Word Integer(number=w2139) -> (16bit integer=w2138:i16)
                        n1114 = Replace Array Subset(array=w2140, new element=w2137, index (row)=w2138, index (col)=1) -> (w2135:string[][])
                      }
                      frame True {
                      }
                    }
                    n1115 = local write "Save1 Array"(w2128) -> ()
                  }
                  frame #1 {
                    n1116 = Search 1D Array(1D array=w2147, element="Length (um):") -> (index of element=w2149:i32)  [unwired: 1 in]
                    n1117 = Equal?(x=w2149, y=-1) -> (x = y?=w2148:bool)
                    n1118 = local read "Save1 Array"() -> (w2146:string[][])
                    n1119 = case shown="True" w2148 {
                      tunnel: w2146 -> [w2157 w2161]
                      tunnel: w2149 -> [w2153 _]
                      tunnel: [w2152 w2161] -> w2145
                      frame False {
                        n1120 = local read "New: Length"() -> (w2159:dbl)
                        n1121 = Number To Fractional String(number=w2159) -> (F-format string=w2154:string)  [unwired: 3 in]
                        n1122 = Divide(x=w2153, y=3) -> (x/y=w2156:dbl)
                        n1123 = To Word Integer(number=w2156) -> (16bit integer=w2155:i16)
                        n1124 = Replace Array Subset(array=w2157, new element=w2154, index (row)=w2155, index (col)=1) -> (w2152:string[][])
                      }
                      frame True {
                      }
                    }
                    n1125 = local write "Save1 Array"(w2145) -> ()
                  }
                  frame #2 {
                    n1126 = Search 1D Array(1D array=w2164, element="Width (um):") -> (index of element=w2166:i32)  [unwired: 1 in]
                    n1127 = Equal?(x=w2166, y=-1) -> (x = y?=w2165:bool)
                    n1128 = local read "Save1 Array"() -> (w2163:string[][])
                    n1129 = case shown="False" w2165 {
                      tunnel: w2166 -> [w2171 _]
                      tunnel: w2163 -> [w2170 w2178]
                      tunnel: [w2169 w2178] -> w2162
                      frame False {
                        n1130 = local read "New: Width"() -> (w2176:dbl)
                        n1131 = Number To Fractional String(number=w2176) -> (F-format string=w2172:string)  [unwired: 3 in]
                        n1132 = Divide(x=w2171, y=3) -> (x/y=w2174:dbl)
                        n1133 = To Word Integer(number=w2174) -> (16bit integer=w2173:i16)
                        n1134 = Replace Array Subset(array=w2170, new element=w2172, index (row)=w2173, index (col)=1) -> (w2169:string[][])
                      }
                      frame True {
                      }
                    }
                    n1135 = local write "Save1 Array"(w2162) -> ()
                  }
                  frame #3 {
                    n1136 = Search 1D Array(1D array=w2181, element="Sample Temp (K):") -> (index of element=w2183:i32)  [unwired: 1 in]
                    n1137 = Equal?(x=w2183, y=-1) -> (x = y?=w2182:bool)
                    n1138 = local read "Save1 Array"() -> (w2180:string[][])
                    n1139 = case shown="False" w2182 {
                      tunnel: w2180 -> [w2191 w2195]
                      tunnel: w2183 -> [w2187 _]
                      tunnel: [w2186 w2195] -> w2179
                      frame False {
                        n1140 = local read "New: Temp"() -> (w2193:dbl)
                        n1141 = Number To Fractional String(number=w2193) -> (F-format string=w2188:string)  [unwired: 3 in]
                        n1142 = Divide(x=w2187, y=3) -> (x/y=w2190:dbl)
                        n1143 = To Word Integer(number=w2190) -> (16bit integer=w2189:i16)
                        n1144 = Replace Array Subset(array=w2191, new element=w2188, index (row)=w2189, index (col)=1) -> (w2186:string[][])
                      }
                      frame True {
                      }
                    }
                    n1145 = local write "Save1 Array"(w2179) -> ()
                  }
                  frame #4 {
                    n1146 = Search 1D Array(1D array=w2198, element="Mobility-Sat (cm^2/Vs):") -> (index of element=w2200:i32)  [unwired: 1 in]
                    n1147 = Equal?(x=w2200, y=-1) -> (x = y?=w2199:bool)
                    n1148 = local read "Save1 Array"() -> (w2196:string[][])
                    n1149 = case shown="False" w2199 {
                      tunnel: w2196 -> [w2208 w2212]
                      tunnel: w2200 -> [w2204 _]
                      tunnel: [w2203 w2212] -> w2197
                      frame False {
                        n1150 = local read "New: Mobility-Sat"() -> (w2210:dbl)
                        n1151 = Number To Fractional String(number=w2210) -> (F-format string=w2205:string)  [unwired: 3 in]
                        n1152 = Divide(x=w2204, y=3) -> (x/y=w2207:dbl)
                        n1153 = To Word Integer(number=w2207) -> (16bit integer=w2206:i16)
                        n1154 = Replace Array Subset(array=w2208, new element=w2205, index (row)=w2206, index (col)=1) -> (w2203:string[][])
                      }
                      frame True {
                      }
                    }
                    n1155 = local write "Save1 Array"(w2197) -> ()
                  }
                  frame #5 {
                    n1156 = Search 1D Array(1D array=w2215, element="Mobility-Lin (cm^2/Vs):") -> (index of element=w2217:i32)  [unwired: 1 in]
                    n1157 = Equal?(x=w2217, y=-1) -> (x = y?=w2216:bool)
                    n1158 = local read "Save1 Array"() -> (w2214:string[][])
                    n1159 = case shown="False" w2216 {
                      tunnel: w2214 -> [w2225 w2229]
                      tunnel: w2217 -> [w2221 _]
                      tunnel: [w2220 w2229] -> w2213
                      frame False {
                        n1160 = local read "Calc: Mobility-Lin"() -> (w2227:dbl)
                        n1161 = Number To Fractional String(number=w2227) -> (F-format string=w2222:string)  [unwired: 3 in]
                        n1162 = Divide(x=w2221, y=3) -> (x/y=w2224:dbl)
                        n1163 = To Word Integer(number=w2224) -> (16bit integer=w2223:i16)
                        n1164 = Replace Array Subset(array=w2225, new element=w2222, index (row)=w2223, index (col)=1) -> (w2220:string[][])
                      }
                      frame True {
                      }
                    }
                    n1165 = local write "Save1 Array"(w2213) -> ()
                  }
                  frame #6 {
                    n1166 = Search 1D Array(1D array=w2232, element="Off I-Sat (A):") -> (index of element=w2234:i32)  [unwired: 1 in]
                    n1167 = Equal?(x=w2234, y=-1) -> (x = y?=w2233:bool)
                    n1168 = local read "Save1 Array"() -> (w2231:string[][])
                    n1169 = case shown="False" w2233 {
                      tunnel: w2231 -> [w2244 w2247]
                      tunnel: w2234 -> [w2241 _]
                      tunnel: [w2240 w2247] -> w2230
                      frame False {
                        n1170 = local read "Calc: Off I-Sat"() -> (w2239:dbl)
                        n1171 = Format Value(format string="%#g", value (0)=w2239) -> (output string=w2238:string)  [unwired: 1 in]
                        n1172 = Divide(x=w2241, y=3) -> (x/y=w2243:dbl)
                        n1173 = To Word Integer(number=w2243) -> (16bit integer=w2242:i16)
                        n1174 = Replace Array Subset(array=w2244, new element=w2238, index (row)=w2242, index (col)=1) -> (w2240:string[][])
                      }
                      frame True {
                      }
                    }
                    n1175 = local write "Save1 Array"(w2230) -> ()
                  }
                  frame #7 {
                    n1176 = Search 1D Array(1D array=w2250, element="Vt-Sat (V):") -> (index of element=w2252:i32)  [unwired: 1 in]
                    n1177 = Equal?(x=w2252, y=-1) -> (x = y?=w2251:bool)
                    n1178 = local read "Save1 Array"() -> (w2249:string[][])
                    n1179 = case shown="False" w2251 {
                      tunnel: w2249 -> [w2260 w2264]
                      tunnel: w2252 -> [w2256 _]
                      tunnel: [w2255 w2264] -> w2248
                      frame False {
                        n1180 = local read "New: VT-Sat"() -> (w2262:dbl)
                        n1181 = Number To Fractional String(number=w2262) -> (F-format string=w2257:string)  [unwired: 3 in]
                        n1182 = Divide(x=w2256, y=3) -> (x/y=w2259:dbl)
                        n1183 = To Word Integer(number=w2259) -> (16bit integer=w2258:i16)
                        n1184 = Replace Array Subset(array=w2260, new element=w2257, index (row)=w2258, index (col)=1) -> (w2255:string[][])
                      }
                      frame True {
                      }
                    }
                    n1185 = local write "Save1 Array"(w2248) -> ()
                  }
                  frame #8 {
                    n1186 = Search 1D Array(1D array=w2267, element="VT-Lin (V):") -> (index of element=w2269:i32)  [unwired: 1 in]
                    n1187 = Equal?(x=w2269, y=-1) -> (x = y?=w2268:bool)
                    n1188 = local read "Save1 Array"() -> (w2266:string[][])
                    n1189 = case shown="True" w2268 {
                      tunnel: w2266 -> [w2277 w2281]
                      tunnel: w2269 -> [w2273 _]
                      tunnel: [w2272 w2281] -> w2265
                      frame False {
                        n1190 = local read "New: VT-Lin"() -> (w2279:dbl)
                        n1191 = Number To Fractional String(number=w2279) -> (F-format string=w2274:string)  [unwired: 3 in]
                        n1192 = Divide(x=w2273, y=3) -> (x/y=w2276:dbl)
                        n1193 = To Word Integer(number=w2276) -> (16bit integer=w2275:i16)
                        n1194 = Replace Array Subset(array=w2277, new element=w2274, index (row)=w2275, index (col)=1) -> (w2272:string[][])
                      }
                      frame True {
                      }
                    }
                    n1195 = local write "Save1 Array"(w2265) -> ()
                  }
                  frame #9 {
                    n1196 = Search 1D Array(1D array=w2284, element="STS-Sat (V/decade):") -> (index of element=w2286:i32)  [unwired: 1 in]
                    n1197 = Equal?(x=w2286, y=-1) -> (x = y?=w2285:bool)
                    n1198 = local read "Save1 Array"() -> (w2283:string[][])
                    n1199 = case shown="False" w2285 {
                      tunnel: w2283 -> [w2294 w2298]
                      tunnel: w2286 -> [w2290 _]
                      tunnel: [w2289 w2298] -> w2282
                      frame False {
                        n1200 = local read "New: STS"() -> (w2296:dbl)
                        n1201 = Number To Fractional String(number=w2296) -> (F-format string=w2291:string)  [unwired: 3 in]
                        n1202 = Divide(x=w2290, y=3) -> (x/y=w2293:dbl)
                        n1203 = To Word Integer(number=w2293) -> (16bit integer=w2292:i16)
                        n1204 = Replace Array Subset(array=w2294, new element=w2291, index (row)=w2292, index (col)=1) -> (w2289:string[][])
                      }
                      frame True {
                      }
                    }
                    n1205 = local write "Save1 Array"(w2282) -> ()
                  }
                  frame #10 {
                    n1206 = Search 1D Array(1D array=w2301, element="Trap Density-VT (Traps/Vcm^2):") -> (index of element=w2303:i32)  [unwired: 1 in]
                    n1207 = Equal?(x=w2303, y=-1) -> (x = y?=w2302:bool)
                    n1208 = local read "Save1 Array"() -> (w2300:string[][])
                    n1209 = case shown="False" w2302 {
                      tunnel: w2300 -> [w2311 w2315]
                      tunnel: w2303 -> [w2307 _]
                      tunnel: [w2306 w2315] -> w2299
                      frame False {
                        n1210 = local read "New: Trap Density-VT"() -> (w2313:dbl)
                        n1211 = Number To Fractional String(number=w2313) -> (F-format string=w2308:string)  [unwired: 3 in]
                        n1212 = Divide(x=w2307, y=3) -> (x/y=w2310:dbl)
                        n1213 = To Word Integer(number=w2310) -> (16bit integer=w2309:i16)
                        n1214 = Replace Array Subset(array=w2311, new element=w2308, index (row)=w2309, index (col)=1) -> (w2306:string[][])
                      }
                      frame True {
                      }
                    }
                    n1215 = local write "Save1 Array"(w2299) -> ()
                  }
                  frame #11 {
                    n1216 = Search 1D Array(1D array=w2318, element="Trap Density-STS (Traps/Vcm^2):") -> (index of element=w2320:i32)  [unwired: 1 in]
                    n1217 = Equal?(x=w2320, y=-1) -> (x = y?=w2319:bool)
                    n1218 = local read "Save1 Array"() -> (w2317:string[][])
                    n1219 = case shown="False" w2319 {
                      tunnel: w2317 -> [w2328 w2332]
                      tunnel: w2320 -> [w2324 _]
                      tunnel: [w2323 w2332] -> w2316
                      frame False {
                        n1220 = local read "New: Trap Density-STS"() -> (w2330:dbl)
                        n1221 = Number To Fractional String(number=w2330) -> (F-format string=w2325:string)  [unwired: 3 in]
                        n1222 = Divide(x=w2324, y=3) -> (x/y=w2327:dbl)
                        n1223 = To Word Integer(number=w2327) -> (16bit integer=w2326:i16)
                        n1224 = Replace Array Subset(array=w2328, new element=w2325, index (row)=w2326, index (col)=1) -> (w2323:string[][])
                      }
                      frame True {
                      }
                    }
                    n1225 = local write "Save1 Array"(w2316) -> ()
                  }
                }
                n1226 = Concatenate Strings(w2125, "\\", w2123) -> (w2124:string)
                n1227 = String To Path(string=w2124) -> (path=w2101:path)
                "No Image 2" <- w2101
                n1228 = local write "Save1 Array"(w2098) -> ()
              }
              frame #1 {
                n1229 = Equal?(x=w2336, y=w2335) -> (x = y?=w2334:bool)
                n1230 = case shown="False" w2334 {
                  tunnel: w2336 -> [w2340 _]
                  tunnel: w2335 -> [w2339 _]
                  frame False {
                    n1231 = Move(source path=w2340, 9:TRUE, 10:w2339) -> ()  [unwired: 2 in, 3 out]
                  }
                  frame True {
                  }
                }
              }
              frame #2 {
                n1232 = local write "Data File"(w2342) -> ()
                n1233 = call-poly <vilib>:"Write To Spreadsheet File.vi"("2D data"=w2341, "file path (dialog if empty)"=w2342) -> ()  [unwired: 6 in, 1 out]
              }
              frame #3 {
                w2442 = 0
                # "Moves to next file and displays new image/data"
                n1234 = property on="Image Out" class="ImageControl"() -> (error out=w2404:errorcluster, "Image Center Position"=w2408:cluster{"X":u32, "Y":u32})  [unwired: 2 in, 1 out]
                n1235 = local read "Data File"() -> (w2447:path)
                n1236 = Strip Path(path=w2447) -> (stripped path=w2438:path, name=w2456:string)
                n1237 = Unbundle(w2408) -> ("X"=w2406:u32)  [unwired: 1 out]
                n1238 = local write "Data Folder"(w2438) -> ()
                n1239 = Bundle("X"=w2406, 0) -> (w2407:cluster{"X":u32, i32})  [unwired: 1 in]
                n1240 = property on="Image Out" class="ImageControl"(error in=w2404, "Image Center Position"=w2407) -> ()  [unwired: 1 in, 2 out]
                n1241 = List Folder(path=w2438) -> (filenames=w2452:string[])  [unwired: 3 in, 3 out]
                n1242 = Search 1D Array(1D array=w2452, element=w2456) -> (index of element=w2449:i32)  [unwired: 1 in]
                n1243 = Array Size(array=w2452) -> (size(s)=w2448:i32)
                n1244 = Decrement(x=w2448) -> (x-1=w2450:i32)
                n1245 = Equal?(x=w2449, y=w2450) -> (x = y?=w2451:bool)
                n1246 = local read "Folder Index"() -> (w2400:dbl)
                n1247 = case shown="False" w2451 {
                  tunnel: w2400 -> [w2581 _]
                  tunnel: [w2580 0] -> w2399
                  frame False {
                    n1248 = Increment(x=w2581) -> (x+1=w2580:dbl)
                  }
                  frame True {
                  }
                }
                n1249 = invoke on="Image Out" class="ImageControl" method="Clear ROI"() -> ()  [unwired: 3 in, 3 out]
                n1250 = local write "Folder Index"(w2399) -> ()
                n1251 = Path To String(path=w2438) -> (string=w2457:string)
                n1252 = Index Array(array=w2452, index=w2399) -> (element=w2453:string)
                n1253 = local write "Data Name:"(w2453) -> ()
                n1254 = Concatenate Strings(w2457, "\\", w2453) -> (w2455:string)
                n1255 = String To Path(string=w2455) -> (path=w2351:path)
                n1256 = call "Recorded Values.vi"("Path"=w2351) -> ("Recorded Char"=w2353:T5, "Recorded Prop"=w2354:T6, "Fabrication Prop"=w2352:T7)  [unwired: 8 in]
                n1257 = Unbundle By Name(w2353) -> ("Mobility-Sat"=w2366:dbl, "Moblitity-Lin"=w2367:dbl, "On/Off"=w2368:dbl, "Off Current"=w2369:dbl, "Vt-Sat"=w2345:dbl, "STS"=w2370:dbl, "Trap Density-VT"=w2371:dbl, "Trap Density-STS"=w2372:dbl)
                n1258 = Unbundle By Name(w2354) -> ("Date Recorded"=w2362:string, "Index"=w2363:string, "Length"=w2364:dbl, "Width"=w2365:dbl, "Sample Temp"=w2348:dbl)
                n1259 = Unbundle By Name(w2352) -> ("Date Created"=w2373:string, "Material"=w2355:string, "Solvent"=w2356:string, "Concentration"=w2357:dbl, "Method"=w2358:string, "Dielectric (nm)"=w2359:dbl, "Treatment"=w2360:string, "Comments"=w2361:string)
                n1260 = local write "Rec: Off I-Sat"(w2369) -> ()
                n1261 = local write "Rec: VT-Sat"(w2345) -> ()
                n1262 = local write "Date Created"(w2373) -> ()
                n1263 = local write "Rec: Material"(w2355) -> ()
                n1264 = local write "Rec: Solvent"(w2356) -> ()
                n1265 = local write "Rec: Concentration"(w2357) -> ()
                n1266 = local write "Rec: Method"(w2358) -> ()
                n1267 = local write "Rec: Dielectric (d)"(w2359) -> ()
                n1268 = local write "Surface Treatment:"(w2360) -> ()
                n1269 = local write "Comments"(w2361) -> ()
                n1270 = local write "Index"(w2363) -> ()
                n1271 = local write "Rec: Mobility-Sat"(w2366) -> ()
                n1272 = local write "Rec: Mobility-Lin"(w2367) -> ()
                n1273 = local write "Rec: On/Off"(w2368) -> ()
                n1274 = local write "Rec: STS"(w2370) -> ()
                n1275 = local write "Rec: Trap Density-VT"(w2371) -> ()
                n1276 = local write "Rec: Trap Density-STS"(w2372) -> ()
                n1277 = local write "Date Recorded"(w2362) -> ()
                n1278 = local write "Rec: Length"(w2364) -> ()
                n1279 = local write "Rec: Width"(w2365) -> ()
                n1280 = local write "Rec: Temp"(w2348) -> ()
                n1281 = Equal To 0?(x=w2348) -> (x = 0?=w2349:bool)
                n1282 = case shown="False" w2349 {
                  tunnel: [w2458 w2459] -> w2346
                  tunnel: w2348 -> [w2458 _]
                  frame False {
                  }
                  frame True {
                    n1283 = local read "Room Temp"() -> (w2459:dbl)
                  }
                }
                n1284 = local write "Data File"(w2351) -> ()
                n1285 = local read "NumPts 2"() -> (w2395:dbl)
                n1286 = local read "NumPts"() -> (w2384:dbl)
                n1287 = local read "NumPts"() -> (w2396:dbl)
                n1288 = call-poly <vilib>:"Read From Spreadsheet File.vi"("file path (dialog if empty)"=w2351) -> ("all rows"=w2444:string[][])  [unwired: 6 in, 4 out]
                n1289 = call "Mobility-Vt Calculator-File.vi"("NumPts"=w2396, "Path"=w2351) -> ("XY Graph-Sat"=w2397:cluster{dbl[], dbl[]}[], "XY Graph-Lin"=w2379:cluster{dbl[], dbl[]}[], "Output"=w2398:T8, "Index-Sat"=w2376:dbl, "Index-Lin"=w2383:dbl)  [unwired: 4 in, 1 out]
                n1290 = Decimate 1D Array(w2379) -> (w2391:cluster{dbl[], dbl[]}[])  [unwired: 1 out]
                n1291 = Array To Cluster(array=w2391) -> (cluster=w2389:T9)
                n1292 = Unbundle(w2389) -> ("[0]"=w2390:cluster{dbl[], dbl[]})  [unwired: 8 out]
                n1293 = local write "XY Graph-Lin"(w2379) -> ()
                n1294 = Unbundle(w2390) -> (w2388:dbl[], w2387:dbl[])
                n1295 = Array Subset(array=w2387, index=w2383, length=w2384) -> (w2385:dbl[])
                n1296 = Array Subset(array=w2388, index=w2383, length=w2384) -> (w2386:dbl[])
                n1297 = call "STS Calculator-File.vi"("NumPts"=w2395, "Path"=w2351) -> ("STS Index-Sat"=w2394:dbl, "XY Graph-Sat"=w2393:cluster{dbl[], dbl[]}[], "Ouput"=w2392:cluster{"STS-Sat":dbl, "STS-Lin":dbl})  [unwired: 5 in, 2 out]
                n1298 = local read "New: Dielectric"() -> (w2378:dbl)
                n1299 = local write "Lin Id-Used"(w2385) -> ()
                n1300 = local write "Lin-Vg Array-Used"(w2386) -> ()
                n1301 = local write "MobVi Index"(w2376) -> ()
                n1302 = local write "Slide"(w2376) -> ()
                n1303 = local write "XY Graph"(w2397) -> ()
                n1304 = local write "Index 2"(w2394) -> ()
                n1305 = local write "XY Graph 2"(w2393) -> ()
                n1306 = Unbundle By Name(w2398) -> ("Mobility-Sat"=w2382:dbl, "Vt-Sat"=w2343:dbl, "Mobility-Lin"=w2381:dbl, "Mobility-Lin"=w2380:dbl, "Off I-Sat"=w2374:dbl, "On/Off I-Sat"=w2344:dbl)
                n1307 = Array Size(array=w2444) -> (size(s)=w2443:i32[])
                n1308 = local write "New: Temp"(w2346) -> ()
                n1309 = Unbundle By Name(w2392) -> ("STS-Sat"=w2377:dbl)
                n1310 = call "Trap Density_STS.vi"("Temp (T) [K]"=w2346, "S.T.S. (S)"=w2377, "Dielectric"=w2378) -> ("Trap Density (N)"=w2350:dbl)  [unwired: 8 in]
                n1311 = local write "Calc: Mobility-Lin"(w2381) -> ()
                n1312 = local write "Calc: Mobility-Sat"(w2382) -> ()
                n1313 = local write "Calc: Off I-Sat"(w2374) -> ()
                n1314 = local write "Calc: VT-Sat"(w2343) -> ()
                n1315 = local write "New: VT-Lin"(w2380) -> ()
                n1316 = local write "New: Trap Density-STS"(w2350) -> ()
                n1317 = local write "Calc: Trap Density-STS"(w2350) -> ()
                n1318 = local read "Image Folder"() -> (w2432:path)
                n1319 = local read "New: Dielectric"() -> (w2375:dbl)
                n1320 = Decimate 1D Array(w2397) -> (w2427:cluster{dbl[], dbl[]}[])  [unwired: 1 out]
                n1321 = Decimate 1D Array(w2393) -> (w2417:cluster{dbl[], dbl[]}[])  [unwired: 1 out]
                n1322 = Index Array(array=w2443, index=w2442) -> (element=w2423:i32)
                n1323 = Array Subset(array=w2444, index (row)=w2442, index (col)=w2442, length (col)=3) -> (w2445:string[][])  [unwired: 1 in]
                n1324 = local write "Calc: STS"(w2377) -> ()
                n1325 = local write "New: VT-Sat"(w2343) -> ()
                n1326 = local write "New: Mobility-Sat"(w2382) -> ()
                n1327 = local write "Calc: On/Off"(w2344) -> ()
                n1328 = local write "New: Mobility-Lin"(w2381) -> ()
                n1329 = List Folder(path=w2432) -> (filenames=w2437:string[])  [unwired: 3 in, 3 out]
                n1330 = local write "New: VT-Lin"(w2380) -> ()
                n1331 = Array To Cluster(array=w2427) -> (cluster=w2429:T9)
                n1332 = Array To Cluster(array=w2417) -> (cluster=w2415:T9)
                n1333 = Reshape Array(w2445, w2423) -> (w2430:string[])
                n1334 = Subtract(x=w2423, y=20) -> (x-y=w2422:i32)
                n1335 = local write "New: STS"(w2377) -> ()
                n1336 = property on="Slide" class="Slide (strict)"("Scale.Maximum"=w2422) -> ()  [unwired: 2 in, 2 out]
                n1337 = call "Trap Density_VT.vi"("VT"=w2343, "Dielectric"=w2375) -> ("Trap Density-VT"=w2347:dbl)
                n1338 = Unbundle(w2429) -> ("[0]"=w2428:cluster{dbl[], dbl[]})  [unwired: 8 out]
                n1339 = Unbundle(w2415) -> ("[0]"=w2416:cluster{dbl[], dbl[]})  [unwired: 8 out]
                n1340 = Search 1D Array(1D array=w2430, element="Index:") -> (index of element=w2439:i32)  [unwired: 1 in]
                n1341 = local write "New: Trap Density-VT"(w2347) -> ()
                n1342 = local write "Calc: Trap Density-VT"(w2347) -> ()
                n1343 = Unbundle(w2428) -> (w2419:dbl[], w2418:dbl[])
                n1344 = Unbundle(w2416) -> (w2414:dbl[], w2413:dbl[])
                n1345 = Increment(x=w2439) -> (x+1=w2440:i32)
                n1346 = Array Subset(array=w2419, index=w2376, length=w2396) -> (w2426:dbl[])
                n1347 = Array Subset(array=w2418, index=w2376, length=w2396) -> (w2425:dbl[])
                n1348 = Array Subset(array=w2414, index=w2394, length=w2395) -> (w2421:dbl[])
                n1349 = Array Subset(array=w2413, index=w2394, length=w2395) -> (w2420:dbl[])
                n1350 = Index Array(array=w2430, index=w2440) -> (element=w2435:string)
                n1351 = local write "Vg Array-Log-Used"(w2420) -> ()
                n1352 = local write "Sat Id-Log-Used"(w2421) -> ()
                n1353 = local write "Sat Id-Used"(w2425) -> ()
                n1354 = local write "Index"(w2435) -> ()
                n1355 = local write "Sat Vg Array-Used"(w2426) -> ()
                n1356 = while {
                  tunnel: w2437 -> [w2467]
                  tunnel: w2435 -> [w2465]
                  tunnel: [w2464] -> _
                  tunnel: [w2464] -> w2436
                  tunnel: w2423 -> [w2463]
                  i -> [w2464]
                  stop <- w2460 stop-if-true
                  n1357 = Index Array(array=w2467, index=w2464) -> (element=w2468:string)
                  n1358 = xnode "Match Regular Expression"("input string"=w2468, "regular expression"=w2465) -> ("whole match"=w2466:string)  [unwired: 4 in, 4 out]
                  n1359 = Equal?(x=w2466, y=w2465) -> (x = y?=w2462:bool)
                  n1360 = Equal?(x=w2463, y=w2464) -> (x = y?=w2461:bool)
                  n1361 = Or(x=w2462, y=w2461) -> (x .or. y?=w2460:bool)
                }
                n1362 = Path To String(path=w2432) -> (string=w2434:string)
                n1363 = Index Array(array=w2437, index=w2436) -> (element=w2411:string)
                n1364 = local write "Image Name"(w2411) -> ()
                n1365 = Empty String/Path?(string/path=w2411) -> (empty?=w2412:bool)
                n1366 = Concatenate Strings(w2434, "\\", w2411) -> (w2433:string)
                n1367 = String To Path(string=w2433) -> (path=w2410:path)
                n1368 = local read "No Image"() -> (w2409:path)
                n1369 = Select(t=w2409, s=w2412, f=w2410) -> (s? t:f=w2403:path)
                n1370 = local write "Image File"(w2403) -> ()
                n1371 = local read "Image Out"() -> (w2401:T2)
                n1372 = call "IMAQ ReadFile"("File Path"=w2403, "Image"=w2401) -> ("Image Out"=w2402:T2)  [unwired: 5 in, 4 out]
                n1373 = local write "Image Out"(w2402) -> ()
                n1374 = local write "Image Out 2"(w2402) -> ()
              }
              frame #4 {
                # "Output ROI data"
                n1375 = local read "Image Folder"() -> (w2583:path)
                n1376 = Build Path(base path=w2583, name or relative path="ROI") -> (appended path=w2585:path)
                n1377 = local read "Index"() -> (w2584:string)
                n1378 = Build Path(base path=w2585, name or relative path=w2584) -> (appended path=w2590:path)
                n1379 = invoke on="Image Out" class="ImageControl" method="Clear ROI"() -> (error out=w2589:errorcluster)  [unwired: 3 in, 2 out]
                n1380 = call <vilib>:"Check if File or Folder Exists.vi"("error in (no error)"=w2589, "path"=w2590) -> ("file or folder exists?"=w2587:bool, "dup path"=w2588:path)  [unwired: 7 in, 1 out]
                n1381 = case shown="True" w2587 {
                  tunnel: w2588 -> [_ w2591]
                  frame False {
                  }
                  frame True {
                    n1382 = Read from Text File(file (use dialog)=w2591) -> (text=w2595:string)  [unwired: 3 in, 3 out]
                    n1383 = property on="Image Out" class="ImageControl"() -> ("ROI"=w2592:T10)  [unwired: 2 in, 2 out]
                    n1384 = Unflatten From String(type=w2592, binary string=w2595) -> (value=w2593:T10, error out=w2594:errorcluster)  [unwired: 3 in, 1 out]
                    n1385 = property on="Image Out" class="ImageControl"(error in=w2594, "ROI"=w2593) -> ()  [unwired: 1 in, 2 out]
                  }
                }
              }
            }
            n1386 = flat-sequence {
              tunnel: [w2055] -> w2042
              tunnel: w2042 -> [w2069]
              frame #0 {
                # "Makes Empty File for Transformer Data"
                n1387 = local read "Data Folder"() -> (w2044:path)
                n1388 = Build Path(base path=w2044, name or relative path="Stats") -> (appended path=w2046:path)
                n1389 = call <vilib>:"Check if File or Folder Exists.vi"("path"=w2046) -> ("file or folder exists?"=w2047:bool, "dup path"=w2048:path)  [unwired: 8 in, 1 out]
                n1390 = case shown="False" w2047 {
                  tunnel: [w2052 w2054] -> w2049
                  tunnel: w2048 -> [w2053 w2054]
                  frame False {
                    n1391 = Create Folder(path (use dialog)=w2053) -> (created path=w2052:path)  [unwired: 2 in, 2 out]
                  }
                  frame True {
                  }
                }
                n1392 = Build Path(base path=w2049, name or relative path="Tranformer Data.txt") -> (appended path=w2051:path)
                n1393 = call-poly <vilib>:"Write To Spreadsheet File.vi"("append to file? (new file:F)"=TRUE, "file path (dialog if empty)"=w2051) -> ()  [unwired: 6 in, 1 out]
              }
              frame #1 {
                # "Adds Headers if they don't exist"
                n1394 = Concatenate Strings("Stats\\", "Tranformer Data.txt") -> (w2062:string)
                n1395 = local read "Data Folder"() -> (w2061:path)
                n1396 = Build Path(base path=w2061, name or relative path=w2062) -> (appended path=w2055:path)
                n1397 = call-poly <vilib>:"Read From Spreadsheet File.vi"("file path (dialog if empty)"=w2055) -> ("first row"=w2060:string[])  [unwired: 6 in, 4 out]
                n1398 = Search 1D Array(1D array=w2060, element="DeviceID") -> (index of element=w2058:i32)  [unwired: 1 in]
                n1399 = Equal?(x=w2058, y=0) -> (x = y?=w2056:bool)
                n1400 = case shown="False" w2056 {
                  tunnel: w2055 -> [w2066 _]
                  frame False {
                    n1401 = local read "Transformer \nHeaders"() -> (w2065:string[])
                    n1402 = call-poly <vilib>:"Write To Spreadsheet File.vi"("1D data"=w2065, "file path (dialog if empty)"=w2066) -> ()  [unwired: 6 in, 1 out]
                  }
                  frame True {
                  }
                }
              }
              frame #2 {
                # "Adds current device if it doesn't exist"
                n1403 = local read "Current \nRecord"() -> (w2072:string[])
                n1404 = Index Array(array=w2072, index=0) -> (element=w2071:string)
                n1405 = Concatenate Strings("Stats\\", "Tranformer Data.txt") -> (w2075:string)
                n1406 = local read "Data Folder"() -> (w2074:path)
                n1407 = local write "Current Device ID"(w2071) -> ()
                n1408 = local read "Current Device ID"() -> (w2081:string)
                n1409 = Build Path(base path=w2074, name or relative path=w2075) -> (appended path=w2073:path)
                n1410 = call-poly <vilib>:"Read From Spreadsheet File.vi"("file path (dialog if empty)"=w2073) -> ("all rows"=w2068:string[][])  [unwired: 6 in, 4 out]
                n1411 = Index Array(array=w2068, index (col)=0) -> (element=w2079:string[])  [unwired: 1 in]
                n1412 = Search 1D Array(1D array=w2079, element=w2081) -> (index of element=w2067:i32)  [unwired: 1 in]
                n1413 = Equal?(x=w2067, y=-1) -> (x = y?=w2070:bool)
                n1414 = case shown="False" w2070 {
                  tunnel: w2069 -> [w2083 w2096]
                  tunnel: w2067 -> [w2088 _]
                  tunnel: w2068 -> [w2089 _]
                  frame False {
                    n1415 = local read "Current \nRecord"() -> (w2087:string[])
                    n1416 = Replace Array Subset(array=w2089, new element=w2087, index (row)=w2088) -> (w2084:string[][])  [unwired: 1 in]
                    n1417 = flat-sequence {
                      tunnel: [w2090] -> _
                      tunnel: [w2091] -> _
                      tunnel: [w2091] -> w2086
                      tunnel: [w2090] -> w2085
                      tunnel: w2084 -> [w2091]
                      tunnel: w2083 -> [w2090]
                      tunnel: w2086 -> [w2093]
                      tunnel: w2085 -> [w2092]
                      frame #0 {
                        n1418 = Delete(path (use dialog)=w2090) -> ()  [unwired: 4 in, 3 out]
                      }
                      frame #1 {
                        n1419 = call-poly <vilib>:"Write To Spreadsheet File.vi"("append to file? (new file:F)"=TRUE, "2D data"=w2093, "file path (dialog if empty)"=w2092) -> ()  [unwired: 5 in, 1 out]
                      }
                    }
                  }
                  frame True {
                    n1420 = local read "Current \nRecord"() -> (w2095:string[])
                    n1421 = call-poly <vilib>:"Write To Spreadsheet File.vi"("append to file? (new file:F)"=TRUE, "1D data"=w2095, "file path (dialog if empty)"=w2096) -> ()  [unwired: 5 in, 1 out]
                  }
                }
              }
            }
          }
          event "Export": Mouse Down {
            n1422 = event-data() -> ()  [unwired: 1 in, 7 out]
            n1423 = local read "Data Folder"() -> (w2599:path)
            n1424 = Build Path(base path=w2599, name or relative path="Stats") -> (appended path=w2600:path)
            n1425 = call <vilib>:"Check if File or Folder Exists.vi"("path"=w2600) -> ("file or folder exists?"=w2616:bool, "dup path"=w2615:path)  [unwired: 8 in, 1 out]
            n1426 = local read "Project"() -> (w2612:path)
            n1427 = call <userlib>:"OA_ConnectToOrigin.vi"() -> ("error out"=w2613:errorcluster, "Origin.IOApplication"=w2614:refnum<k7>)  [unwired: 8 in]
            n1428 = case shown="False" w2616 {
              tunnel: w2615 -> [w2725 w2726]
              tunnel: [w2724 w2726] -> w2598
              frame False {
                n1429 = Create Folder(path (use dialog)=w2725) -> (created path=w2724:path)  [unwired: 2 in, 2 out]
              }
              frame True {
              }
            }
            n1430 = call <userlib>:"OA_Load.vi"("error in (no error)"=w2613, "Path"=w2612, "Origin.IOApplication"=w2614) -> ("error out"=w2610:errorcluster, "Origin.IOApplication"=w2611:refnum<k7>)  [unwired: 1 out]
            n1431 = call <userlib>:"OAExecute.vi"("script"="document -m 3;", "Error IO"=w2610, "Origin.IOApplication"=w2611) -> ("Error IO Out"=w2608:errorcluster, "Origin.IOApplication"=w2609:refnum<k7>)  [unwired: 1 in, 1 out]
            n1432 = stacked-sequence {
              tunnel: w2599 -> [w2628 w2631 w2644 w2657 w2670 w2683 w2697 w2711]
              tunnel: w2598 -> [w2627 w2632 w2645 w2658 w2671 w2684 w2696 w2712]
              tunnel: w2609 -> [w2624 w2634 w2647 w2660 w2673 w2686 w2699 w2714]
              tunnel: w2608 -> [w2626 w2633 w2646 w2659 w2672 w2685 w2698 w2713]
              tunnel: [_ _ _ _ _ _ _ w2709] -> w2597
              tunnel: [_ _ _ _ _ _ _ w2710] -> w2596
              frame #0 {
                n1433 = call "Param_Analysis_7_24b_JW.vi"("error in (no error)"=w2626, "Data Folder"=w2628, "Parameter String"="Mobility-Sat (cm^2/Vs):", "Parameter Name"="Mobility-Sat", "Stats Folder"=w2627) -> ("error out"=w2620:errorcluster, "Output Array"=w2618:string[][])  [unwired: 4 in, 1 out]
                n1434 = call "Origin_Export_7_24a_JW.vi"("Analysis Array"=w2618, "error in (no error)"=w2620, "Parameter Worksheet Name"="[MOBSvsLTable]Mobilities", "Parameter Folder Script"="pe_cd \"Mobility-Sat\";", "Origin.IOApplication"=w2624) -> ("error out"=w2619:errorcluster, "reference out"=w2621:refnum<k7>)  [unwired: 4 in, 1 out]
                n1435 = call <userlib>:"OAExecute.vi"("script"="window -a MOBSvsLTable;\nwindow -s TV;", "Error IO"=w2619, "Origin.IOApplication"=w2621) -> ()  [unwired: 1 in, 3 out]
              }
              frame #1 {
                n1436 = call "Param_Analysis_7_24b_JW.vi"("error in (no error)"=w2633, "Data Folder"=w2631, "Parameter String"="Mobility-Lin (cm^2/Vs):", "Parameter Name"="Mobility-Lin", "Stats Folder"=w2632) -> ("error out"=w2636:errorcluster, "Output Array"=w2638:string[][])  [unwired: 4 in, 1 out]
                n1437 = call "Origin_Export_7_24a_JW.vi"("Analysis Array"=w2638, "error in (no error)"=w2636, "Parameter Worksheet Name"="[MOBLvsLTable]Mobilities", "Parameter Folder Script"="pe_cd \"Mobility-Lin\";", "Origin.IOApplication"=w2634) -> ("error out"=w2635:errorcluster, "reference out"=w2637:refnum<k7>)  [unwired: 4 in, 1 out]
                n1438 = call <userlib>:"OAExecute.vi"("script"="window -a MOBLvsLTable;\nwindow -s TV;", "Error IO"=w2635, "Origin.IOApplication"=w2637) -> ()  [unwired: 1 in, 3 out]
              }
              frame #2 {
                n1439 = call "Param_Analysis_7_24b_JW.vi"("error in (no error)"=w2646, "Data Folder"=w2644, "Parameter String"="Off I-Sat (A):", "Parameter Name"="Off I-Sat", "Stats Folder"=w2645) -> ("error out"=w2650:errorcluster, "Output Array"=w2648:string[][])  [unwired: 4 in, 1 out]
                n1440 = call "Origin_Export_7_24a_JW.vi"("Analysis Array"=w2648, "error in (no error)"=w2650, "Parameter Worksheet Name"="[OffItable]OffCurrents", "Parameter Folder Script"="pe_cd \"Off I-Sat\";", "Origin.IOApplication"=w2647) -> ("error out"=w2649:errorcluster, "reference out"=w2651:refnum<k7>)  [unwired: 4 in, 1 out]
                n1441 = call <userlib>:"OAExecute.vi"("script"="window -a OffItable;\nwindow -s TV;", "Error IO"=w2649, "Origin.IOApplication"=w2651) -> ()  [unwired: 1 in, 3 out]
              }
              frame #3 {
                n1442 = call "Param_Analysis_7_24b_JW.vi"("error in (no error)"=w2659, "Data Folder"=w2657, "Parameter String"="On/Off I-Sat:", "Parameter Name"="OnOff Ratio", "Stats Folder"=w2658) -> ("error out"=w2663:errorcluster, "Output Array"=w2661:string[][])  [unwired: 4 in, 1 out]
                n1443 = call "Origin_Export_7_24a_JW.vi"("Analysis Array"=w2661, "error in (no error)"=w2663, "Parameter Worksheet Name"="[OnOffTable]On/Off Ratios", "Parameter Folder Script"="pe_cd \"On Off Ratio\";", "Origin.IOApplication"=w2660) -> ("error out"=w2662:errorcluster, "reference out"=w2664:refnum<k7>)  [unwired: 4 in, 1 out]
                n1444 = call <userlib>:"OAExecute.vi"("script"="window -a OnOffTable;\nwindow -s TV;", "Error IO"=w2662, "Origin.IOApplication"=w2664) -> ()  [unwired: 1 in, 3 out]
              }
              frame #4 {
                n1445 = call "Param_Analysis_7_24b_JW.vi"("error in (no error)"=w2672, "Data Folder"=w2670, "Parameter String"="STS-Sat (V/decade):", "Parameter Name"="STS-Sat", "Stats Folder"=w2671) -> ("error out"=w2676:errorcluster, "Output Array"=w2674:string[][])  [unwired: 4 in, 1 out]
                n1446 = call "Origin_Export_7_24a_JW.vi"("Analysis Array"=w2674, "error in (no error)"=w2676, "Parameter Worksheet Name"="[STable]Threshold Swing", "Parameter Folder Script"="pe_cd \"STS-Sat\";", "Origin.IOApplication"=w2673) -> ("error out"=w2675:errorcluster, "reference out"=w2677:refnum<k7>)  [unwired: 4 in, 1 out]
                n1447 = call <userlib>:"OAExecute.vi"("script"="window -a STable;\nwindow -s TV;", "Error IO"=w2675, "Origin.IOApplication"=w2677) -> ()  [unwired: 1 in, 3 out]
              }
              frame #5 {
                n1448 = call "Param_Analysis_7_24b_JW.vi"("error in (no error)"=w2685, "Data Folder"=w2683, "Parameter String"="Trap Density-STS (Traps/Vcm^2):", "Parameter Name"="Trap Density-STS", "Stats Folder"=w2684) -> ("error out"=w2689:errorcluster, "Output Array"=w2687:string[][])  [unwired: 4 in, 1 out]
                n1449 = call "Origin_Export_7_24a_JW.vi"("Analysis Array"=w2687, "error in (no error)"=w2689, "Parameter Worksheet Name"="[NSTSTable]Trap Densities", "Parameter Folder Script"="pe_cd \"Trap Density-STS\";", "Origin.IOApplication"=w2686) -> ("error out"=w2688:errorcluster, "reference out"=w2690:refnum<k7>)  [unwired: 4 in, 1 out]
                n1450 = call <userlib>:"OAExecute.vi"("script"="window -a NSTSTable;\nwindow -s TV;", "Error IO"=w2688, "Origin.IOApplication"=w2690) -> ()  [unwired: 1 in, 3 out]
              }
              frame #6 {
                n1451 = call "Param_Analysis_7_24b_JW.vi"("error in (no error)"=w2698, "Data Folder"=w2697, "Parameter String"="Trap Density-Vt (Traps/Vcm^2):", "Parameter Name"="Trap Density-Vt", "Stats Folder"=w2696) -> ("error out"=w2702:errorcluster, "Output Array"=w2700:string[][])  [unwired: 4 in, 1 out]
                n1452 = call "Origin_Export_7_24a_JW.vi"("Analysis Array"=w2700, "error in (no error)"=w2702, "Parameter Worksheet Name"="[NVTTable]Trap Densities", "Parameter Folder Script"="pe_cd \"Trap Density-Vt\";", "Origin.IOApplication"=w2699) -> ("error out"=w2701:errorcluster, "reference out"=w2703:refnum<k7>)  [unwired: 4 in, 1 out]
                n1453 = call <userlib>:"OAExecute.vi"("script"="window -a NVTTable;\nwindow -s TV;", "Error IO"=w2701, "Origin.IOApplication"=w2703) -> ()  [unwired: 1 in, 3 out]
              }
              frame #7 {
                n1454 = call "Param_Analysis_7_24b_JW.vi"("error in (no error)"=w2713, "Data Folder"=w2711, "Parameter String"="Vt-Sat (V):", "Parameter Name"="Vt-Sat", "Stats Folder"=w2712) -> ("error out"=w2717:errorcluster, "Output Array"=w2715:string[][])  [unwired: 4 in, 1 out]
                n1455 = call "Origin_Export_7_24a_JW.vi"("Analysis Array"=w2715, "error in (no error)"=w2717, "Parameter Worksheet Name"="[VtTable]Threshold Voltages", "Parameter Folder Script"="pe_cd \"Vt-Sat\";", "Origin.IOApplication"=w2714) -> ("error out"=w2716:errorcluster, "reference out"=w2718:refnum<k7>)  [unwired: 4 in, 1 out]
                n1456 = call <userlib>:"OAExecute.vi"("script"="window -a VtTable;\nwindow -s TV;", "Error IO"=w2716, "Origin.IOApplication"=w2718) -> ("Error IO Out"=w2709:errorcluster, "Origin.IOApplication"=w2710:refnum<k7>)  [unwired: 1 in, 1 out]
              }
            }
            n1457 = call "File Dialog"("start path"=w2600) -> ("selected path"=w2603:path)  [unwired: 11 in, 3 out]
            n1458 = Path To String(path=w2603) -> (string=w2602:string)
            n1459 = call <userlib>:"OAExecute.vi"("script"="pe_cd /; ", "Error IO"=w2597, "Origin.IOApplication"=w2596) -> ("Error IO Out"=w2604:errorcluster, "Origin.IOApplication"=w2605:refnum<k7>)  [unwired: 1 in, 1 out]
            n1460 = call <userlib>:"OASaveProject.vi"("path"=w2602, "Error IO"=w2604, "Origin.IOApplication"=w2605) -> ()  [unwired: 3 out]
          }
          event "Blank Button": Mouse Down {
            n1461 = event-data() -> ()  [unwired: 1 in, 7 out]
            n1462 = local read "Data File"() -> (w2734:path)
            n1463 = Strip Path(path=w2734) -> (stripped path=w2730:path, name=w2732:string)
            n1464 = Path To String(path=w2730) -> (string=w2729:string)
            n1465 = Concatenate Strings(w2729, "\\", "X_", w2732) -> (w2728:string)
            n1466 = String To Path(string=w2728) -> (path=w2727:path)
            n1467 = Move(source path=w2734, 10:w2727) -> ()  [unwired: 3 in, 3 out]
            n1468 = local write "Data File"(w2727) -> ()
          }
          event "Cancel Button": Mouse Down {
            (unwired) 6
            n1469 = event-data() -> ()  [unwired: 1 in, 7 out]
            n1470 = call "Simulate_Keyboard.vi"("Action"=2, "Virtual Key"=162) -> ()  [unwired: 7 in, 1 out]
          }
        }
        n1471 = Multiply(x=w523, y=10) -> (x*y=w525:sgl)
        n1472 = case shown="\"0\"" w564 {
          tunnel: w538 -> [w617 w623 w627 w629 w633 w635 w637 w639 w641 w643 w645 w647 w649 w651 w653 w655 w657 w659 w661 w663 w665 w667 w669 w671 w673 w675 w677 w679 w681 w683 w685 w687 w689 w691 w693 w695 w697 w699 w701 w703 w705 w707 w709 w711 w713 w715 w717 w719 w721 w723 w725 w727 w729 w731 w733 w735 w737 w739 w741 w743 w745 w747 w749 w751 w753 w755 w757 w759 w761 w763 w765 w767 w769 w771 w773 w775 w777 w779 w781 w783 w785 w787 w789 w791 w793 w795 w797 w799 w801 w803 w805 w807 w809 w811 w813 w815 w817 w819 w821 w823 w825 w827 w829 w831 w833]
          tunnel: [w617 w622 w626 w629 w633 w635 w637 w639 w641 w643 w645 w647 w649 w651 w653 w655 w657 w659 w661 w663 w665 w667 w669 w671 w673 w675 w677 w679 w681 w683 w685 w687 w689 w691 w693 w695 w697 w699 w701 w703 w705 w707 w709 w711 w713 w715 w717 w719 w721 w723 w725 w727 w729 w731 w733 w735 w737 w739 w741 w743 w745 w747 w749 w751 w753 w755 w757 w759 w761 w763 w765 w767 w769 w771 w773 w775 w777 w779 w781 w783 w785 w787 w789 w791 w793 w795 w797 w799 w801 w803 w805 w807 w809 w811 w813 w815 w817 w819 w821 w823 w825 w827 w829 w831 w833] -> w563
          tunnel: w539 -> [w619 w621 w625 w631 w632 w634 w636 w638 w640 w642 w644 w646 w648 w650 w652 w654 w656 w658 w660 w662 w664 w666 w668 w670 w672 w674 w676 w678 w680 w682 w684 w686 w688 w690 w692 w694 w696 w698 w700 w702 w704 w706 w708 w710 w712 w714 w716 w718 w720 w722 w724 w726 w728 w730 w732 w734 w736 w738 w740 w742 w744 w746 w748 w750 w752 w754 w756 w758 w760 w762 w764 w766 w768 w770 w772 w774 w776 w778 w780 w782 w784 w786 w788 w790 w792 w794 w796 w798 w800 w802 w804 w806 w808 w810 w812 w814 w816 w818 w820 w822 w824 w826 w828 w830 w832]
          tunnel: [w618 w621 w625 w630 w632 w634 w636 w638 w640 w642 w644 w646 w648 w650 w652 w654 w656 w658 w660 w662 w664 w666 w668 w670 w672 w674 w676 w678 w680 w682 w684 w686 w688 w690 w692 w694 w696 w698 w700 w702 w704 w706 w708 w710 w712 w714 w716 w718 w720 w722 w724 w726 w728 w730 w732 w734 w736 w738 w740 w742 w744 w746 w748 w750 w752 w754 w756 w758 w760 w762 w764 w766 w768 w770 w772 w774 w776 w778 w780 w782 w784 w786 w788 w790 w792 w794 w796 w798 w800 w802 w804 w806 w808 w810 w812 w814 w816 w818 w820 w822 w824 w826 w828 w830 w832] -> w562
          tunnel: w525 -> [w616 w620 w624 w628 _ _ _ _ _ _ _ _ _ _ _ _ _ _ _ _ _ _ _ _ _ _ _ _ _ _ _ _ _ _ _ _ _ _ _ _ _ _ _ _ _ _ _ _ _ _ _ _ _ _ _ _ _ _ _ _ _ _ _ _ _ _ _ _ _ _ _ _ _ _ _ _ _ _ _ _ _ _ _ _ _ _ _ _ _ _ _ _ _ _ _ _ _ _ _ _ _ _ _ _ _]
          frame "DOWN" {
            n1473 = Add(x=w619, y=w616) -> (x+y=w618:sgl)
          }
          frame "LEFT" {
            n1474 = Subtract(x=w623, y=w620) -> (x-y=w622:sgl)
          }
          frame "RIGHT" {
            n1475 = Add(x=w627, y=w624) -> (x+y=w626:sgl)
          }
          frame "UP" {
            n1476 = Subtract(x=w631, y=w628) -> (x-y=w630:sgl)
          }
          frame "ENTER (num pad)" {
          }
          frame "' (quote)" {
          }
          frame "END" {
          }
          frame "EQUALS" {
          }
          frame "ESCAPE" {
          }
          frame "GRAVE (`)" {
          }
          frame "HOME" {
          }
          frame "INSERT" {
          }
          frame "LBRACKET" {
          }
          frame "LCONTROL" {
          }
          frame "L ALT" {
          }
          frame "LSHIFT" {
          }
          frame "LWIN" {
          }
          frame "MINUS" {
          }
          frame "MULTIPLY" {
          }
          frame "NEXT" {
          }
          frame "NUMLOCK" {
          }
          frame "NUMPAD_0" {
          }
          frame "NUMPAD_1" {
          }
          frame "NUMPAD_2" {
          }
          frame "NUMPAD_3" {
          }
          frame "NUMPAD_4" {
          }
          frame "NUMPAD_5" {
          }
          frame "NUMPAD_6" {
          }
          frame "NUMPAD_7" {
          }
          frame "NUMPAD_8" {
          }
          frame "NUMPAD_9" {
          }
          frame "PAUSE" {
          }
          frame "PERIOD" {
          }
          frame "PRIOR (PG UP)" {
          }
          frame "RBRACKET" {
          }
          frame "RCONTROL" {
          }
          frame "RETURN" {
          }
          frame "R ALT" {
          }
          frame "RSHIFT" {
          }
          frame "RWIN" {
          }
          frame "SCROLL" {
          }
          frame "SEMICOLON" {
          }
          frame "SLASH" {
          }
          frame "SPACE" {
          }
          frame "SUBTRACT" {
          }
          frame "TAB" {
          }
          frame "DIVIDE" {
          }
          frame "DELETE" {
          }
          frame "DECIMAL" {
          }
          frame "COMMA" {
          }
          frame "CAPITAL" {
          }
          frame "BACKSLASH" {
          }
          frame "BACK" {
          }
          frame "ADD" {
          }
          frame "F15" {
          }
          frame "F14" {
          }
          frame "F13" {
          }
          frame "F12" {
          }
          frame "F11" {
          }
          frame "F10" {
          }
          frame "F9" {
          }
          frame "F8" {
          }
          frame "F7" {
          }
          frame "F6" {
          }
          frame "F5" {
          }
          frame "F4" {
          }
          frame "F3" {
          }
          frame "F2" {
          }
          frame "F1" {
          }
          frame "Z" {
          }
          frame "Y" {
          }
          frame "X" {
          }
          frame "W" {
          }
          frame "V" {
          }
          frame "U" {
          }
          frame "T" {
          }
          frame "S" {
          }
          frame "R" {
          }
          frame "Q" {
          }
          frame "P" {
          }
          frame "O" {
          }
          frame "N" {
          }
          frame "M" {
          }
          frame "L" {
          }
          frame "K" {
          }
          frame "J" {
          }
          frame "I" {
          }
          frame "H" {
          }
          frame "G" {
          }
          frame "F" {
          }
          frame "E" {
          }
          frame "D" {
          }
          frame "C" {
          }
          frame "B" {
          }
          frame "A" {
          }
          frame "9" {
          }
          frame "8" {
          }
          frame "7" {
          }
          frame "6" {
          }
          frame "5" {
          }
          frame "4" {
          }
          frame "3" {
          }
          frame "2" {
          }
          frame "1" {
          }
          frame "0" {
          }
        }
        n1477 = Bundle(w541, w540, w555, w554, 0.0) -> (w553:cluster{dbl, dbl, dbl, dbl, dbl})  [unwired: 1 in]
        n1478 = Bundle("X"=w563, "Y"=w562) -> (w557:cluster{"X":sgl, "Y":sgl})  [unwired: 1 in]
        n1479 = Divide(x=20, y=w524) -> (x/y=w527:sgl)
        n1480 = property on="Image Out" class="ImageControl"("Image Center Position"=w557) -> ()  [unwired: 2 in, 2 out]
        n1481 = call "IMAQ Convert Rectangle to ROI (Polygon)"("Rectangle"=w553) -> ("ROI Descriptor"=w551:T3)  [unwired: 7 in, 2 out]
        n1482 = Bundle("Application Font", w527, w531, w531, w531, w531, w531, TRUE, w529) -> (w533:T16)  [unwired: 1 in]
        n1483 = property on="Image Out 2" class="ImageControl"("ROI"=w551) -> ()  [unwired: 2 in, 2 out]
        n1484 = Bundle(w529, w533, w529, w529) -> (w532:T17)  [unwired: 1 in]
        n1485 = property on="Image Out" class="ImageControl"() -> ("ROI"=w516:T10)  [unwired: 2 in, 2 out]
        n1486 = Unbundle By Name(w516) -> ("Contours"=w580:T14)
        n1487 = local read "Image Out"() -> (w535:T2)
        n1488 = call "IMAQ Clear Overlay"("Image"=w535) -> ("Image Out"=w534:T2)  [unwired: 9 in, 1 out]
        n1489 = Initialize Array(0) -> (w578:i32[])  [unwired: 1 in]
        n1490 = local read "Magnification"() -> (w569:u16)
        n1491 = Array Size(array=w580) -> (size(s)=w579:i32)
        n1492 = Build Array(0.505025, 0.252522, 0.127742, 0.050345, 0.031129) -> (w570:dbl[])
        n1493 = Array Subset(array=w570, index=w569, length=1) -> (w567:dbl[])
        n1494 = property on="Image Out" class="ImageControl"() -> ("ZoomInteger"=w559:cluster{"X":i32, "Y":i32})  [unwired: 2 in, 2 out]
        n1495 = To Double Precision Float(number=w567) -> (double precision float=w566:dbl[])
        n1496 = for {
          N: w579 -> [_]
          shift-right: [w856] -> _
          shift-left: w580 -> [w856]
          shift-right: [w854] -> w565
          shift-left: w578 -> [w853]
          tunnel: w566 -> [w852]
          shift-right: [w849] -> _
          shift-left: w534 -> [w851]
          tunnel: w532 -> [w844]
          i -> [w848]
          n1497 = Index Array(array=w856, index=w848) -> (element=w865:T18)
          n1498 = Unbundle(w865) -> ("Points"=w864:i32[])  [unwired: 2 out]
          n1499 = Array To Cluster(array=w864) -> (cluster=w863:T19)
          n1500 = Unbundle(w863) -> ("Points[0]"=w843:i32, "Points[1]"=w840:i32, "Points[2]"=w855:i32, "Points[3]"=w861:i32)  [unwired: 5 out]
          n1501 = Add(x=w843, y=10) -> (x+y=w841:i32)
          n1502 = Subtract(x=w840, y=w861) -> (x-y=w860:i32)
          n1503 = Subtract(x=w843, y=w855) -> (x-y=w862:i32)
          n1504 = Square(x=w860) -> (x^2=w858:i32)
          n1505 = Square(x=w862) -> (x^2=w859:i32)
          n1506 = Add(x=w859, y=w858) -> (x+y=w857:i32)
          n1507 = Square Root(x=w857) -> (sqrt(x)=w834:dbl)
          n1508 = Multiply(x=w834, y=0.5) -> (x*y=w837:dbl)
          n1509 = Add(x=w837, y=w840) -> (x+y=w839:dbl)
          n1510 = Bundle(w841, w839) -> (w850:cluster{i32, dbl})  [unwired: 1 in]
          n1511 = Multiply(x=w834, y=w852) -> (x*y=w847:dbl[])
          n1512 = Index Array(array=w847) -> (element=w846:dbl)  [unwired: 1 in]
          n1513 = Number To Fractional String(number=w846) -> (F-format string=w845:string)  [unwired: 3 in]
          n1514 = call "IMAQ Overlay Text"("BG Color (Transparent)"=u32 0, "Text Color (black)"=u32 16448250, "Font, Size & Style"=w844, "String"=w845, "Origin"=w850, "Image"=w851) -> ("Image Out"=w849:T2)  [unwired: 4 in, 1 out]
          n1515 = Build Array (concatenate)(w853, w847) -> (w854:dbl[])
          n1516 = local write "Numeric 3"(w834) -> ()
        }
        n1517 = local write "ROI Descriptor"(w516) -> ()
        n1518 = Unbundle(w559) -> ("X"=w558:i32)  [unwired: 1 out]
        n1519 = Add Array Elements(numeric array=w565) -> (sum=w576:dbl)
        n1520 = local write "Distances"(w565) -> ()
        n1521 = local write "Total Width"(w576) -> ()
        n1522 = local write "Zoom"(w558) -> ()
        n1523 = local read "Manual-Width"() -> (w515:bool)
        n1524 = local read "Total Width"() -> (w519:dbl)
        n1525 = local read "Rec: Width"() -> (w517:dbl)
        n1526 = Not(x=w515) -> (.not. x?=w513:bool)
        n1527 = Equal To 0?(x=w519) -> (x = 0?=w514:bool)
        n1528 = Or(x=w514, y=w515) -> (x .or. y?=w518:bool)
        n1529 = And(x=w514, y=w513) -> (x .and. y?=w512:bool)
        n1530 = case shown="True" w512 {
          tunnel: w517 -> [_ w594]
          frame False {
          }
          frame True {
            n1531 = local write "New: Width"(w594) -> ()
          }
        }
        n1532 = case shown="False" w518 {
          tunnel: w519 -> [w595 _]
          frame False {
            n1533 = local write "New: Width"(w595) -> ()
          }
          frame True {
          }
        }
        n1534 = local read "Manuel-Dielectric"() -> (w441:bool)
        n1535 = local read "Rec: Dielectric (d)"() -> (w440:dbl)
        n1536 = local read "Manuel-Length"() -> (w442:bool)
        n1537 = local read "Rec: Length"() -> (w443:dbl)
        n1538 = case shown="False" w442 {
          tunnel: w443 -> [w585 _]
          frame False {
            n1539 = local write "New: Length"(w585) -> ()
          }
          frame True {
          }
        }
        n1540 = case shown="False" w441 {
          tunnel: w440 -> [w584 _]
          frame False {
            n1541 = local write "New: Dielectric"(w584) -> ()
          }
          frame True {
          }
        }
      }
    }
  }
  n1542 = Build Array("DeviceID", "Fabricator", "Deposition", "Date", "Sample", "Row", "Column", "L (um)", "W (um)", "Material", "Treatment", "TC (mM)", "Solvent", "C (%)", "ST (C)", "Drops", "Wait (s)", "RT (F)", "RH (%)", "Ramp (s)", "RPM", "Accel (RPM/s)", "Time (s)", "Mobility", "On/Off", "Vt", "S.T.S") -> (→"Transformer \nHeaders":string[])
